vi "EC_Applied_XYZ_MM_BR_RES_2_NC_GR_pxi_Acc3_preset_LIM.vi"() -> ()   [LabVIEW 2009]
uses:
  <vilib>/Utility/file.llb/Read From Spreadsheet File (I64).vi
  <vilib>/Utility/file.llb/Read From Spreadsheet File (string).vi
  <vilib>/Instr/_visa.llb/VISA Configure Serial Port (Instr).vi
  <vilib>/Utility/file.llb/Write To Spreadsheet File (I64).vi
  <vilib>/Utility/file.llb/Write To Spreadsheet File (string).vi
panel:
  out "R Velocity MVdeg/sec":dbl format="%.3f"
  out "R Position MV deg":dbl
  out "Z Velocity MV mm/sec":dbl format="%.3f"
  out "Z Position MV mm":dbl
  out "Y Velocity MV mm/sec":dbl format="%.3f"
  out "Y Position MV mm":dbl
  out "X Velocity MV mm/sec":dbl format="%.3f"
  out "X Position MV mm":dbl
  out "Presets":i32[][](array[numeric])
  in  "stop":bool
  in  "Tab Control 3":enum32{"Status", "Reset"}(tab)
  out "Y in Range":bool
  out "Y Scan":bool
  out "Y in Motion":bool
  out "Y Backlash corr":bool
  out "X  in Range":bool
  out "X Scan":bool
  out "X  in Motion":bool
  out "X Backlash corr":bool
  out "Z in Range":bool
  out "Z Scan":bool
  out "Z in Motion":bool
  out "Z Backlash corr":bool
  out "R in Range":bool
  out "R Scan":bool
  out "R in Motion":bool
  out "R Backlash corr":bool
  out "X Ready":bool
  out "Y Ready":bool
  out "Z Ready":bool
  out "R Ready":bool
  in  "Reset Y Position mm":dbl
  out "Reset Y Motor Steps":i32
  in  "Reset X Position mm":dbl
  out "Reset X Motor Steps":i32
  in  "Reset Z Position mm":dbl
  out "Reset Z Motor Steps":i32
  in  "Reset R Position deg":dbl
  out "Reset R Motor Steps":i32
  in  "Reset":bool
  in  "Tab Control 2":enum32{"mm", "step"}(tab)
  in  "X Scan Length SP mm":dbl
  in  "X Scan Velocity SP mm/sec":dbl
  in  "X Scan set":bool
  in  "Y Scan Length SP mm":dbl
  in  "Y Scan Velocity SP mm/sec":dbl
  in  "Y Scan set":bool
  in  "Z Scan Length SP mm":dbl
  in  "Z Scan Velocity SP mm/sec":dbl
  in  "Z Scan set":bool
  in  "R Scan Length SP deg":dbl
  in  "R Scan Velocity SP deg/sec":dbl
  in  "R Scan set":bool
  in  "X Scan Velocity SP steps/sec":i32=1 min=1 max=102400 step=1
  in  "X Scan Length SP steps":i32 min=-500000 max=500000 step=100
  out "X Scan length MV mm":dbl
  out "X Scan velocity MV mm/sec":dbl format="%#_6f"
  in  "Y Scan Velocity SP steps/sec":i32=1 min=1 max=102400 step=1
  in  "Y Scan Length SP steps":i32 min=-1000000 max=0 step=100
  out "Y Scan length MV mm":dbl
  out "Y Scan velocity MV mm/sec":dbl format="%#_6f"
  in  "Z Scan Velocity SP steps/sec":i32=1 min=1 max=102400 step=1
  in  "Z Scan Length SP steps":i32 min=-204724 max=102195276 step=100
  out "Z Scan length MV mm":dbl
  out "Z Scan velocity MV mm/sec":dbl format="%#_6f"
  in  "R Scan Velocity SP steps/sec":i32=1 min=1 max=102400 step=1
  in  "R Scan Length SP steps":i32 min=-6144000 max=0 step=100
  out "R Scan length MV deg":dbl
  out "R Scan velocity MV deg/sec":dbl format="%#_6f"
  out "atan Y/Z":dbl
  in  "Tab Control":enum32{"mm", "preset", "step"}(tab)
  in  "X Position SP mm":dbl
  in  "X Velocity SP mm/sec":dbl
  in  "X Move Set":bool
  in  "Y Move Set":bool
  in  "Y Position SP mm":dbl
  in  "Y Velocity SP mm/sec":dbl
  in  "Z Position SP mm":dbl
  in  "Z Velocity SP mm/sec":dbl
  in  "Z Move Set":bool
  in  "R Position SP deg":dbl
  in  "R Velocity SP deg/sec":dbl
  in  "R Move Set":bool
  in  "Add Button":bool
  in  "String":string
  in  "Delete Button":bool
  in  "Preset positions":i32(ring) items=["ZERO", "Default", "CDOSE", "QMS", "test", "test2", "test3"]
  in  "Set Button":bool
  in  "X Velocity SP step/sec":i32 min=1 max=50000
  in  "Y Velocity SP step/sec":i32 min=1 max=50000
  in  "Z Velocity SP step/sec":i32 min=1 max=5000
  in  "R Velocity SP step/sec":i32 min=1 max=10000
  in  "Y Step SP":i32=-20000 min=-800000 max=800000 step=500
  in  "X Step SP":i32=-20000 min=-800000 max=800000 step=500
  in  "Z Step SP":i32=-20000 min=0 max=102400000 step=500
  in  "R Step SP":i32=-20000 min=-6144000 max=0 step=500
  out "X Step PV":i32 max=2000
  out "Y Step PV":i32 max=2000
  out "Z Step PV":i32 max=2000
  out "R Step PV":i32 max=2000
  in  "Clear ZY":bool
  out "ZY Graph":cluster{"Y":dbl[], "Y":dbl[]}[](graph)
  out "ZR Graph":cluster{"Y":dbl[], "Y":dbl[]}[](graph)
  out "XY Graph":cluster{"Y":dbl[], "Y":dbl[]}[](graph)
  out "X Scan Duration":dbl
  out "Y Scan Duration":dbl
  out "Z Scan Duration":dbl
  out "R Scan Duration":dbl
  out "R Backlash steps/sec":i32
  out "R Backlash":i32
  out "R Holding Current %":i32
  out "R Run Current %":i32
  out "R offset deg":dbl
  out "R deg/rev":dbl
  out "R steps/rev":u32
  out "R velocity PV step/sec":i32
  out "R MINPOS":i32=-94296
  out "R MAXPOS":i32=-34296
  out "R COM PORT":refnum<visa-resource-name>="COM5"
  in  "R Scan OK":bool
  in  "R Go":bool
  out "R Position deg PV":dbl
  out "Z COM PORT":refnum<visa-resource-name>="COM5"
  out "Z Backlash steps/sec":i32
  out "Z Backlash":i32
  out "Z Holding Current %":i32
  out "Z Run Current %":i32
  out "Z offset mm":dbl
  out "Z mm/rev":dbl
  out "Z steps/rev":u32
  out "Z  velocity PV step/sec":i32
  out "Z MINPOS":i32=-94296
  out "Z MAXPOS":i32=-34296
  in  "Z Scan OK":bool
  in  "Z Go":bool
  out "Z Position mm PV":dbl
  out "X Position mm PV":dbl
  out "X velocity PV step/sec":i32
  in  "X Scan OK":bool
  in  "X Go":bool
  out "X Backlash steps/sec":i32
  out "X Backlash":i32
  out "X Holding Current %":i32
  out "X Run Current %":i32
  out "X offset mm":dbl
  out "X mm/rev":dbl
  out "X steps/rev":u32
  out "X MAXPOS":i32=-34296
  out "X MINPOS":i32=-94296
  out "X COM PORT":refnum<visa-resource-name>="COM5"
  out "Y Backlash steps/sec":i32
  out "Y Backlash":i32
  out "Y Holding Current %":i32
  out "Y Run Current %":i32
  in  "Scan Cancel":bool
  out "Y Position mm PV":dbl
  out "Y offset mm":dbl
  out "Y mm/rev":dbl
  out "Y steps/rev":u32
  out "Y velocity PV step/sec":i32
  in  "Y Scan OK":bool
  in  "Scan Go":bool
  in  "Stop":bool
  in  "Y Go":bool
  out "Y MINPOS":i32=-94296
  out "Y MAXPOS":i32=-34296
  out "Y COM PORT":refnum<visa-resource-name>="COM5"
  # "Current position"
  # "Goto position"
  # "RX"
  # "RY"
  # "RZ"
  # "RR"
  # "L"
  # "M"
  # "B"
  # "S"
  # "R"
  # "Preset position"
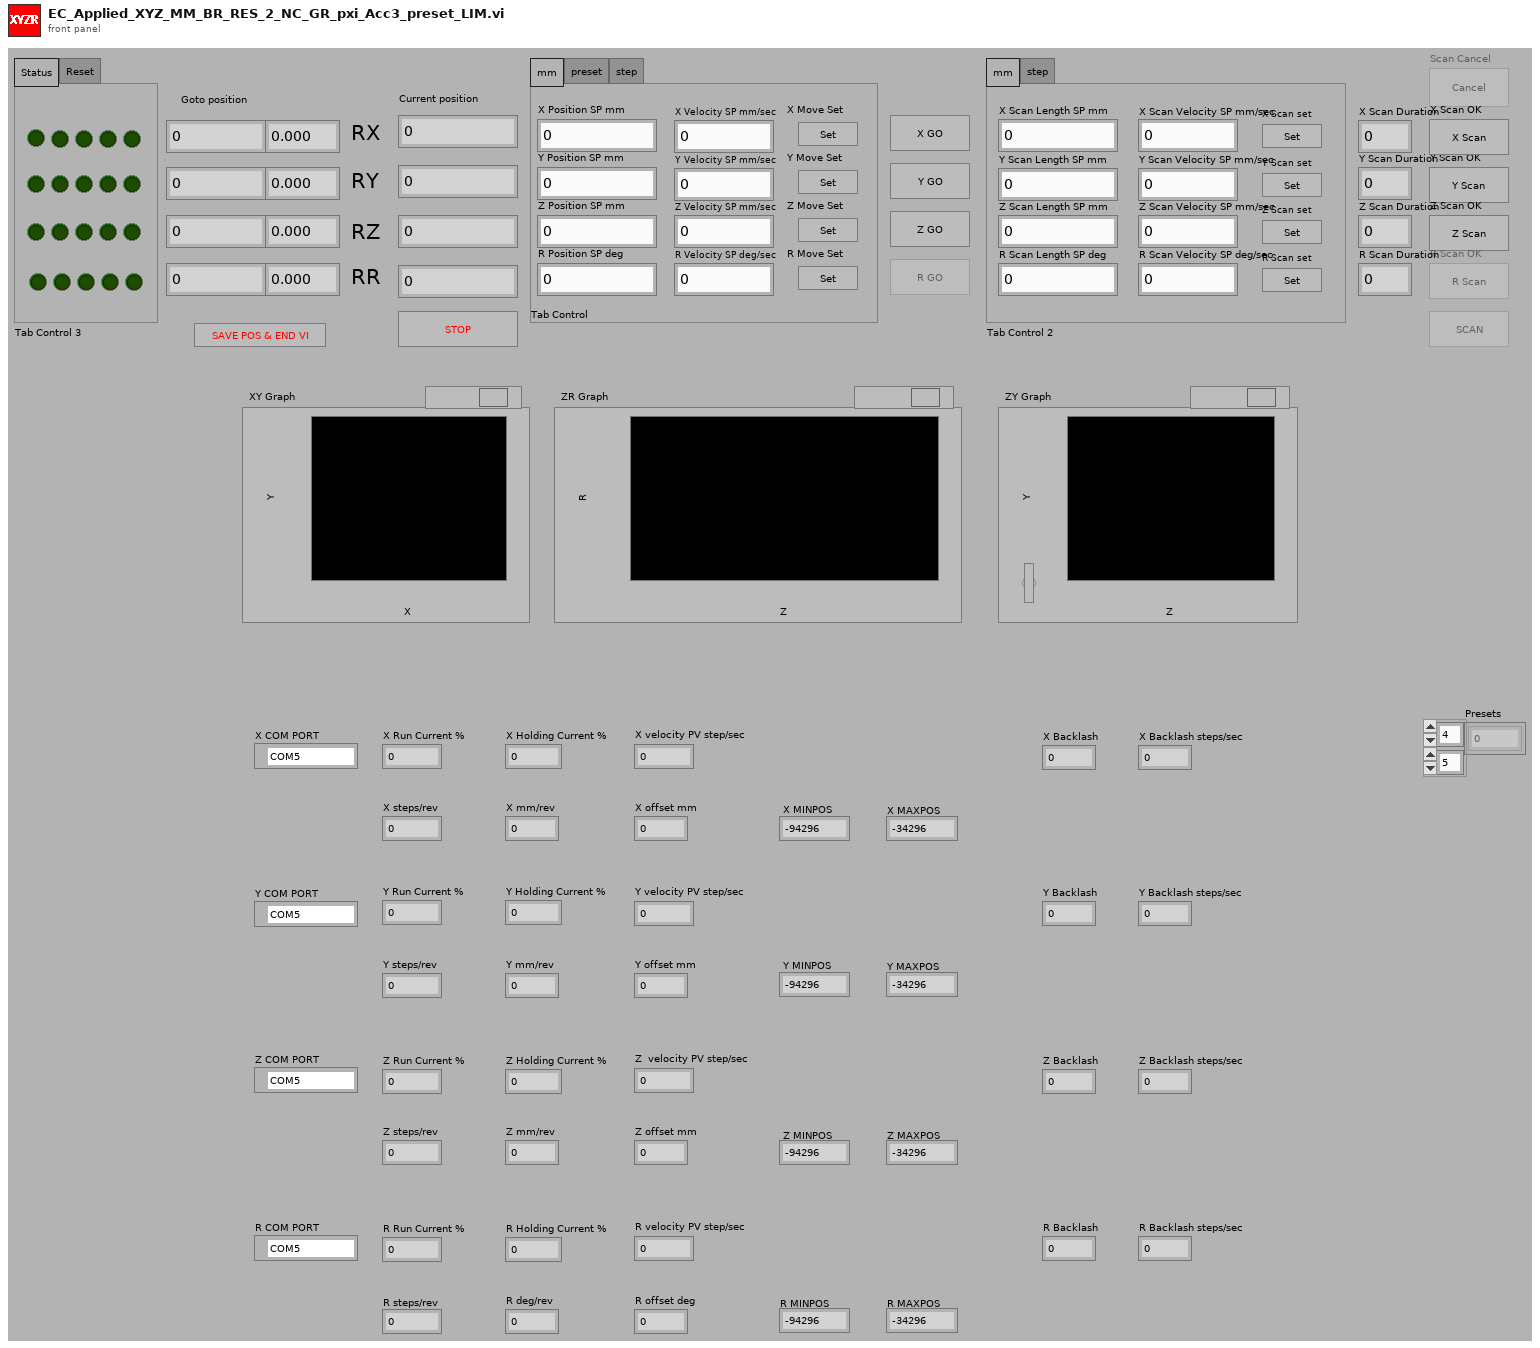
[diagram p1: front panel]
types:
  T1 = enum16{"Power-up Signature", "Accel Rate", "Accel Max", "Bit Rate", "Buffer Status", "Change Current", "Commence Jogging", "Change Jog Speed", "Continue", "Define Address", "Distance for FC,FM,FO,FY", "Decel Rate", "Distance or Position", "Define Limits", "Encoder Deadband", "Encoder Function", "Encoder Position", "Encoder Ratio", "Feed to Length with Speed Change", "Feed to Length", "Feed to Sensor with Mask Dist", "Feed to Length & Set Output", "Feed to Position", "Feed to Sensor", "Feed to Sensor w/safety", "Follow Handwheel", "Immediate Distance?", "Immediate Encoder?", "Immediate Low Output", "Immediate High Output", "Immediate Position?", "Input Status?", "Jog Accel/Decel", "Jog Disable", "Jog Enable", "Jog Speed", "Motor Disable", "Motor Enable", "Microstep Resolution", "Power up Current", "Power up Mode", "Pause", "Request Status", "Revision Level?", "Seek Home", "Stop Jogging", "Stop & Kill Buffer", "Set Output", "Set ABS Position", "Send String", "Stop", "Velocity for Speed Change", "Velocity Setting", "Wait for Input", "Wait Time"}
  T2 = enum8{"Enabled", "Disabled", "Disabled and Grayed Out"}
  T3 = cluster{"first row[0]":i64, "first row[1]":i64, "first row[2]":i64, "first row[3]":i64, "first row[4]":i64, "first row[5]":i64, "first row[6]":i64, "first row[7]":i64, "first row[8]":i64}
  T4 = cluster{"Value[0]":i32, "Value[1]":i32, "Value[2]":i32, "Value[3]":i32, "Value[4]":i32, "Value[5]":i32, "Value[6]":i32, "Value[7]":i32, "Value[8]":i32}
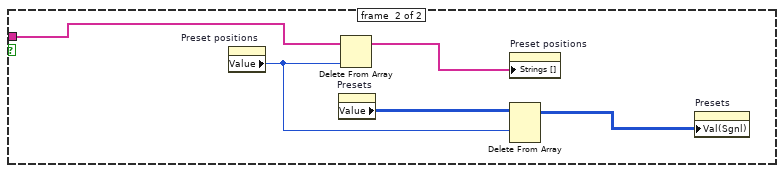
[diagram p2: hidden frame]
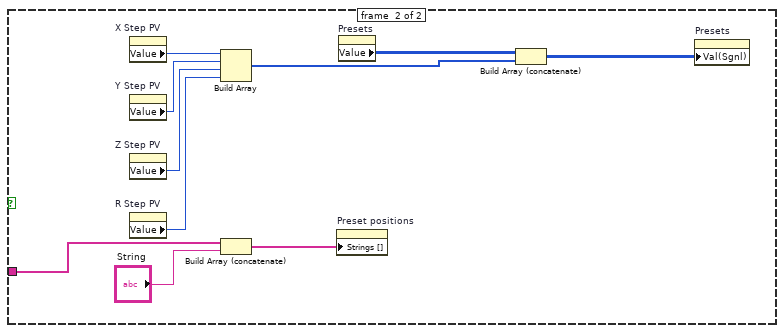
[diagram p3: hidden frame]
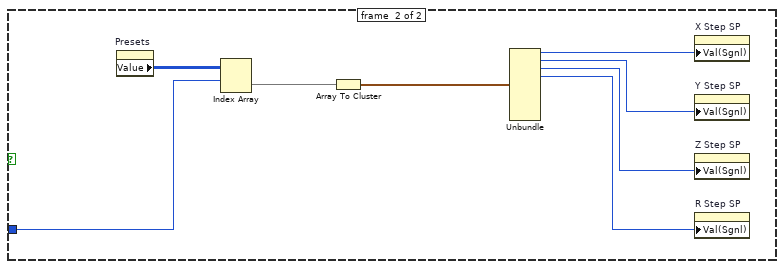
[diagram p4: hidden frame]
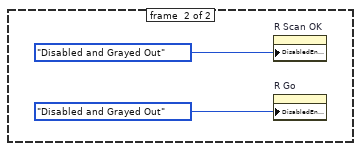
[diagram p5: hidden frame]
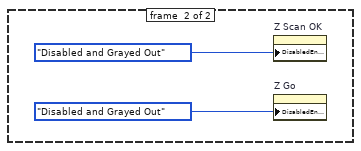
[diagram p8: hidden frame]
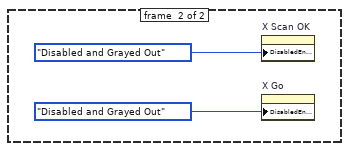
[diagram p11: hidden frame]
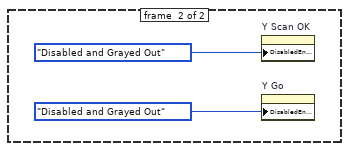
[diagram p14: hidden frame]
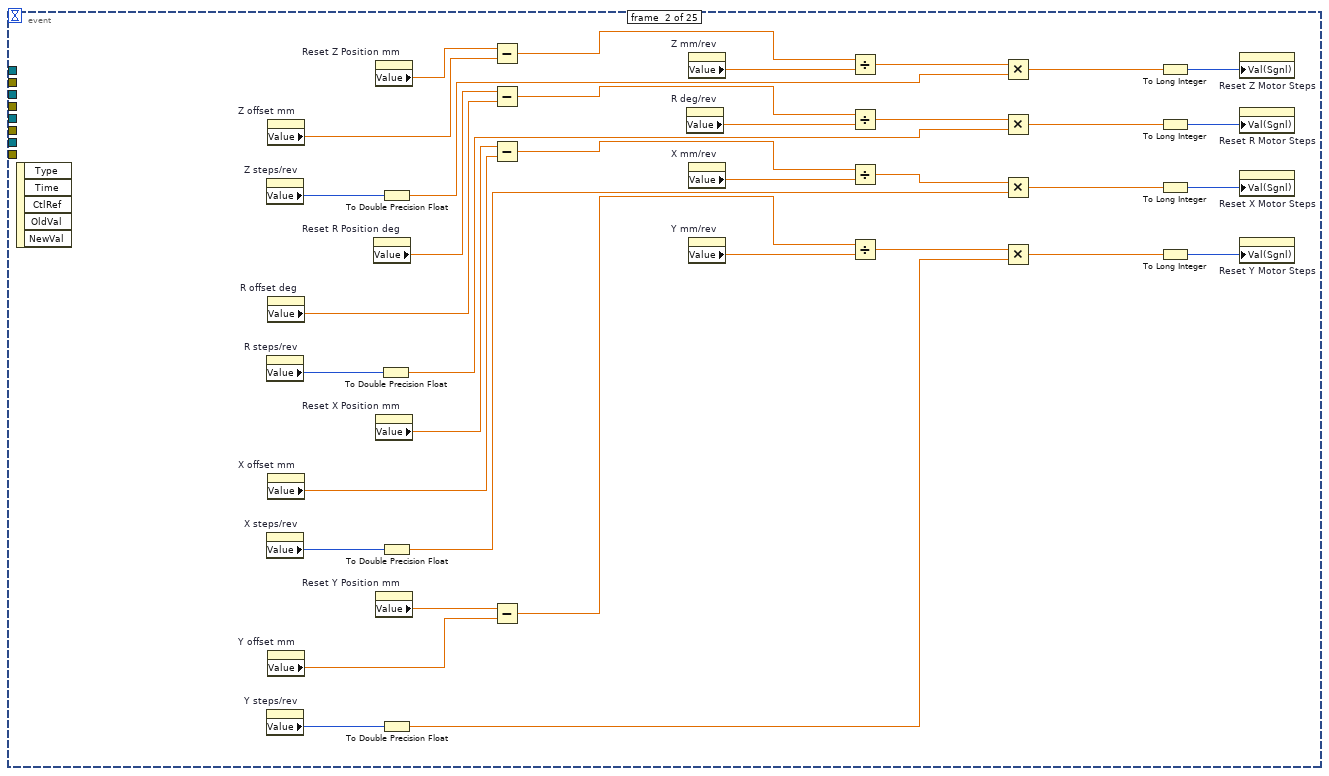
[diagram p17: hidden frame]
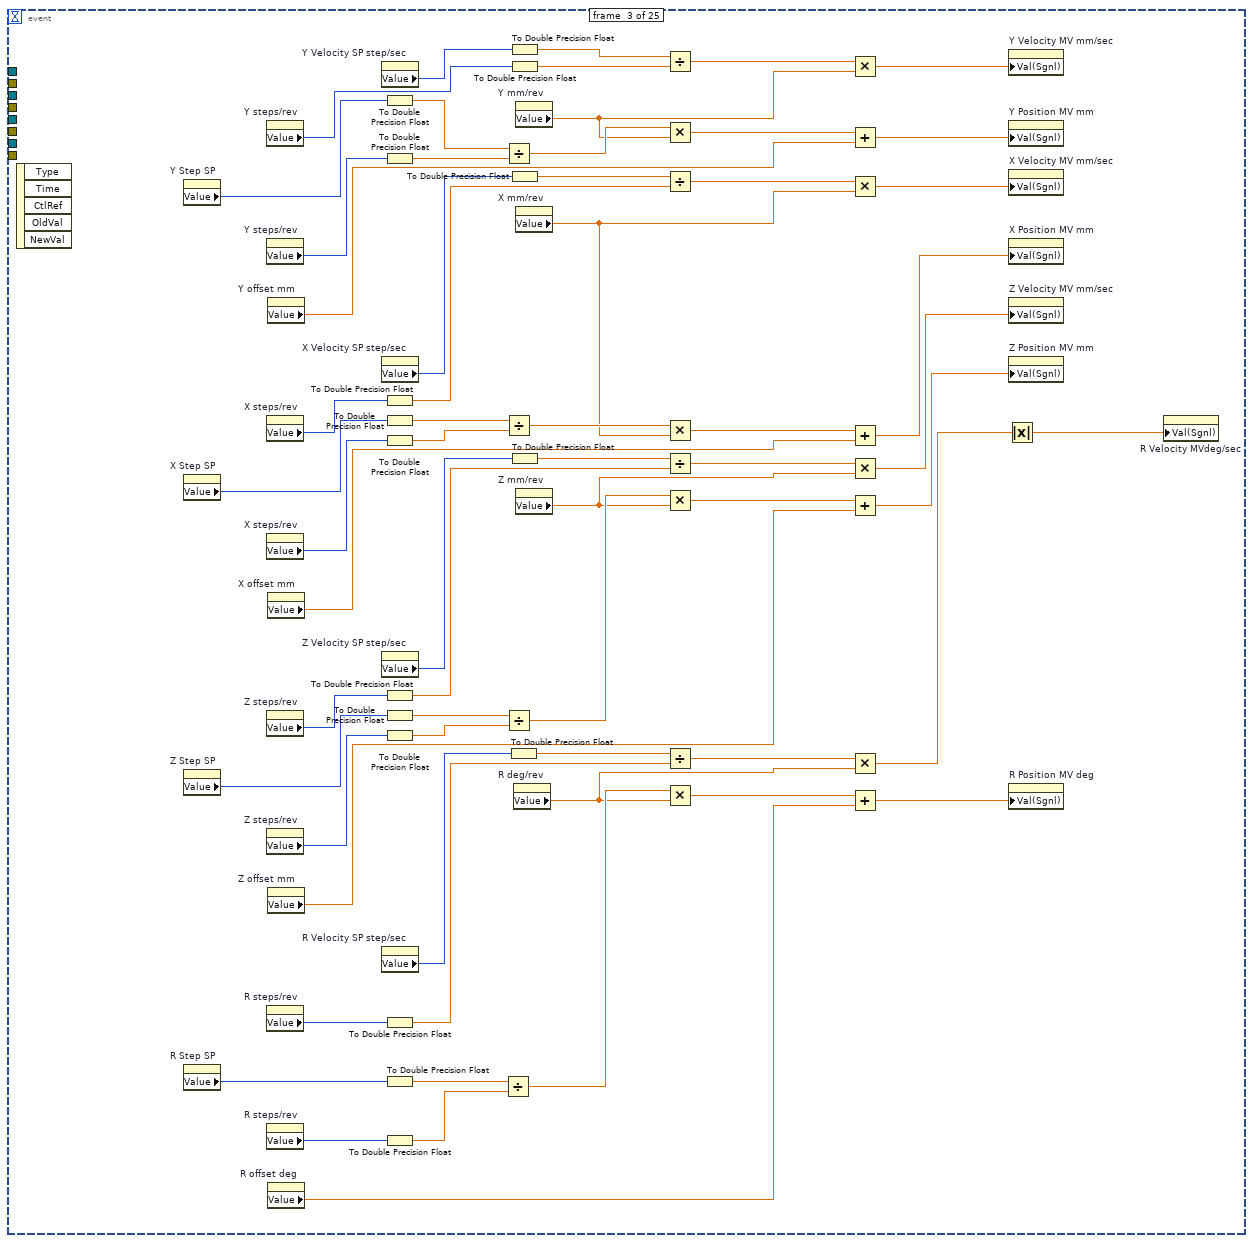
[diagram p18: hidden frame]
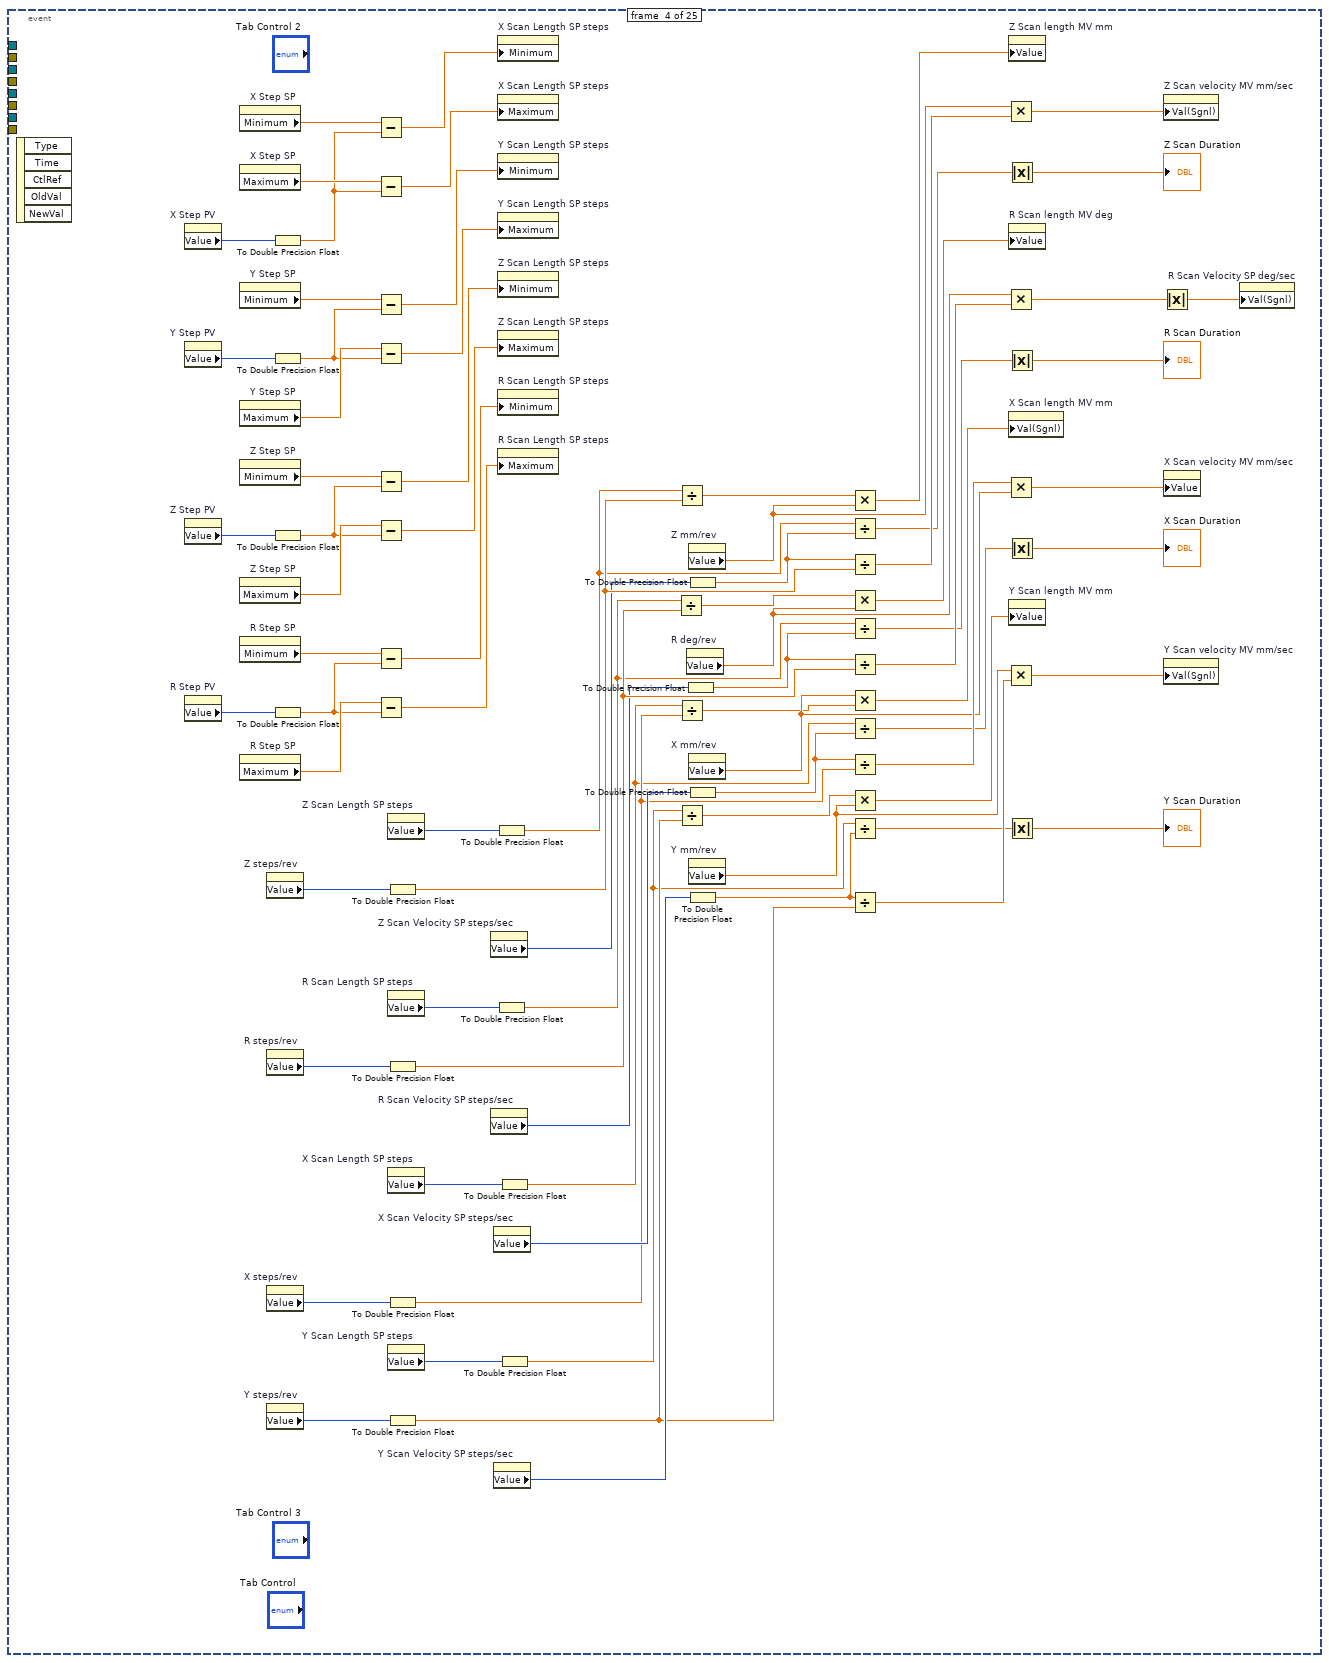
[diagram p19: hidden frame]
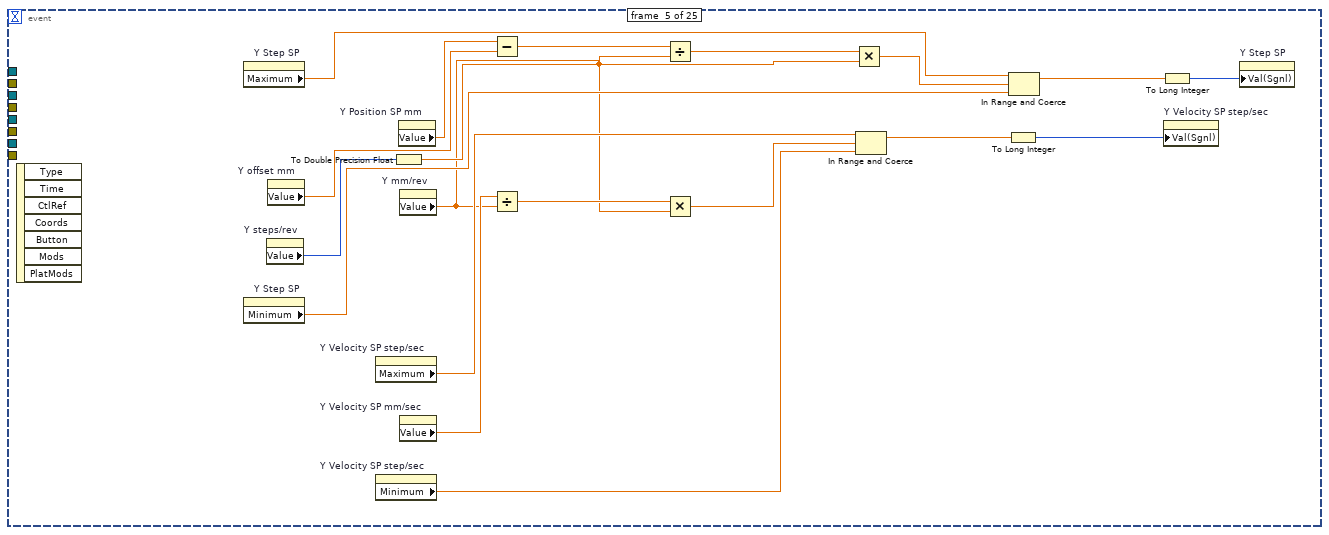
[diagram p20: hidden frame]
diagram:
  w24 = 0 ("dimension size")
  n1 = flat-sequence {
    tunnel: [w93] -> w10
    tunnel: [w92] -> w9
    tunnel: w10 -> [w104]
    tunnel: w9 -> [w103]
    tunnel: [w102] -> w8
    tunnel: [w101] -> w7
    tunnel: [w113] -> w64
    tunnel: [w112] -> w63
    tunnel: w8 -> [w115]
    tunnel: w7 -> [w114]
    tunnel: w64 -> [w130]
    tunnel: w63 -> [w129]
    tunnel: [w131] -> w62
    tunnel: [w132] -> w61
    tunnel: [w133] -> w6
    tunnel: [w144] -> w55
    tunnel: [w145] -> w56
    tunnel: w62 -> [w145]
    tunnel: w61 -> [w144]
    tunnel: w6 -> [w142]
    frame #0 {
      "Z Run Current %" <- 100 ("Z Run Current %")
      "Z Holding Current %" <- 50 ("Z Holding Current %")
    }
    frame #1 {
      "Z Backlash steps/sec" <- 1000 ("Z Backlash steps/sec")
      "Z Backlash" <- -5000 ("Z Backlash")
    }
    frame #2 {
      w83 = 2.54 ("Z mm/rev")
      w82 = u32 20000 ("step/rev")
      w84 = 5000 ("Value (Signaling)")
      n2 = property on="Z Velocity SP step/sec" class="DigNum (strict)"("Minimum"=1.0 ("Data Entry Limits:Minimum")) -> ()  [unwired: 2 in, 2 out]
      n3 = property on="Z Scan Velocity SP mm/sec" class="DigNum (strict)"("Val(Sgnl)"=0.1 ("Value (Signaling)")) -> ()  [unwired: 2 in, 2 out]
      n4 = property on="Z Velocity SP step/sec" class="DigNum (strict)"("Val(Sgnl)"=w84) -> ()  [unwired: 2 in, 2 out]
      n5 = To Double Precision Float(number=w82) -> (double precision float=w87:dbl)
      n6 = To Double Precision Float(number=w84) -> (double precision float=w88:dbl)
      n7 = Divide(x=w88, y=w87) -> (x/y=w85:dbl)
      n8 = property on="Z Velocity SP step/sec" class="DigNum (strict)"("Maximum"=w88) -> ()  [unwired: 2 in, 2 out]
      n9 = Multiply(x=w85, y=w83) -> (x*y=w86:dbl)
      n10 = property on="Z Velocity SP mm/sec" class="DigNum (strict)"("Val(Sgnl)"=w86) -> ()  [unwired: 2 in, 2 out]
      "Z mm/rev" <- w83
      "Z steps/rev" <- w82
    }
    frame #3 {
      w90 = 0 ("lower limit")
      w89 = 102400000 ("upper limit")
      n11 = property on="Z Step SP" class="DigNum (strict)"("Minimum"=w90) -> ()  [unwired: 2 in, 2 out]
      n12 = property on="Z Step SP" class="DigNum (strict)"("Maximum"=w89) -> ()  [unwired: 2 in, 2 out]
      "Z offset mm" <- 0.0 ("Z offset mm")
      "Z MINPOS" <- w90
      "Z MAXPOS" <- w89
    }
    frame #4 {
      w100 = refnum<visa-resource-name> "COM5" ("COM PORT")
      w98 = u16 0 items=["None", "XON/XOFF", "RTS/CTS", "XON/XOFF & RTS/CTS", "DTR/DSR", "XON/XOFF & DTR/DSR"] ("flow control (0:none)")
      w97 = u16 10 items=["1.0"=10, "1.5"=15, "2.0"=20] ("stop bits (10: 1 bit)")
      # "Stop bits"
      n13 = call-poly "VISA Configure Serial Port"("VISA resource name"=w100, "timeout (10sec)"=u32 10000, "baud rate (9600)"=u32 9600, "data bits (8)"=u16 8, "parity (0:none)"=enum16{"None", "Odd", "Even", "Mark", "Space"}."None", "stop bits (10: 1 bit)"=w97, "flow control (0:none)"=w98) -> ("VISA resource name out"=w93:refnum<visa-resource-name>, "error out"=w92:errorcluster)  [unwired: 7 in]
      "Z COM PORT" <- w100
    }
    frame #5 {
      # "Run Current %"
      n14 = property on="Z Run Current %" class="DigNum (strict)"() -> ("Value"=w105:i32)  [unwired: 2 in, 2 out]
      n15 = Divide(x=w105, y=3.5) -> (x/y=w107:dbl)
      n16 = Number To Fractional String(number=w107) -> (F-format string=w108:string)  [unwired: 3 in]
      n17 = call "Applied Send Command.vi"("error in (no error)"=w103, "Extra"=w108, "Command"=T1."Change Current", "VISA resource name"=w104) -> ("error out"=w101:errorcluster, "VISA resource name out"=w102:refnum<visa-resource-name>)  [unwired: 3 in, 1 out]
    }
    frame #6 {
      # "VELOCITY"
      n18 = property on="Z steps/rev" class="DigNum (strict)"() -> ("Value"=w111:u32)  [unwired: 2 in, 2 out]
      n19 = property on="Z Velocity SP step/sec" class="DigNum (strict)"() -> ("Value"=w110:i32)  [unwired: 2 in, 2 out]
      n20 = Divide(x=w110, y=w111) -> (x/y=w118:dbl)
      n21 = Number To Fractional String(number=w118) -> (F-format string=w120:string)  [unwired: 3 in]
      n22 = call "Applied Send Command.vi"("error in (no error)"=w114, "Extra"=w120, "Command"=T1."Velocity Setting", "VISA resource name"=w115) -> ("error out"=w121:errorcluster, "VISA resource name out"=w128:refnum<visa-resource-name>)  [unwired: 3 in, 1 out]
      n23 = call "Time Delay2"("error in (no error)"=w121, "Delay Time (s)"=0.1) -> ("error out"=w126:errorcluster)  [unwired: 9 in]
      n24 = call "Applied Send Command.vi"("error in (no error)"=w126, "Extra"="", "Command"=T1."Velocity Setting", "VISA resource name"=w128) -> ("error out"=w112:errorcluster, "read buffer"=w124:string, "VISA resource name out"=w113:refnum<visa-resource-name>)  [unwired: 3 in]
      n25 = Fract/Exp String To Number(string=w124, offset=3) -> (number=w119:dbl)  [unwired: 2 in, 1 out]
      n26 = Multiply(x=w119, y=w111) -> (x*y=w116:dbl)
      n27 = property on="Z  velocity PV step/sec" class="DigNum (strict)"("Val(Sgnl)"=w116) -> ()  [unwired: 2 in, 2 out]
    }
    frame #7 {
      # "GET CURRENT POSITION"
      n28 = call "Applied Send Command.vi"("error in (no error)"=w129, "Extra"="", "Command"=T1."Immediate Position?", "VISA resource name"=w130) -> ("error out"=w135:errorcluster, "read buffer"=w137:string, "VISA resource name out"=w131:refnum<visa-resource-name>)  [unwired: 3 in]
      n29 = call "Time Delay8"("error in (no error)"=w135, "Delay Time (s)"=0.1) -> ("error out"=w132:errorcluster)  [unwired: 9 in]
      n30 = Hexadecimal String To Number(string=w137, offset=3) -> (number=w133:u32)  [unwired: 1 in, 1 out]
    }
    frame #8 {
      n31 = property on="Z Step SP" class="DigNum (strict)"("Val(Sgnl)"=w142) -> ()  [unwired: 2 in, 2 out]
      n32 = property on="Z Step SP" class="DigNum (strict)"() -> ("Maximum"=w141:dbl)  [unwired: 2 in, 2 out]
      n33 = property on="Z Step SP" class="DigNum (strict)"() -> ("Minimum"=w140:dbl)  [unwired: 2 in, 2 out]
      n34 = In Range and Coerce(upper limit=w141, x=w142, lower limit=w140) -> (In Range?=w143:bool)  [unwired: 1 out]
      n35 = property on="Z in Range" class="Bool (strict)"("Val(Sgnl)"=w143) -> ()  [unwired: 2 in, 2 out]
    }
  }
  n36 = flat-sequence {
    tunnel: [w164] -> w3
    tunnel: [w163] -> w2
    tunnel: [w175] -> w5
    tunnel: [w174] -> w4
    tunnel: w3 -> [w173]
    tunnel: w2 -> [w172]
    tunnel: [w183] -> w60
    tunnel: [w184] -> w59
    tunnel: w5 -> [w181]
    tunnel: w4 -> [w182]
    tunnel: w60 -> [w201]
    tunnel: w59 -> [w200]
    tunnel: [w202] -> w58
    tunnel: [w204] -> w57
    tunnel: [w203] -> w1
    tunnel: [w215] -> w53
    tunnel: [w216] -> w54
    tunnel: w58 -> [w215]
    tunnel: w57 -> [w213]
    tunnel: w1 -> [w216]
    frame #0 {
      "R Run Current %" <- 100 ("R Run Current %")
      "R Holding Current %" <- 50 ("R Holding Current %")
    }
    frame #1 {
      "R Backlash" <- -12800 ("R Backlash")
      "R Backlash steps/sec" <- 6400 ("R Backlash steps/sec")
    }
    frame #2 {
      w154 = -3.0 ("R deg/rev")
      w156 = u32 20000 ("step/rev")
      w152 = 10000 ("Value (Signaling)")
      n37 = property on="R Velocity SP deg/sec" class="DigNum (strict)"("Val(Sgnl)"=0.1 ("Value (Signaling)")) -> ()  [unwired: 2 in, 2 out]
      n38 = property on="R Velocity SP step/sec" class="DigNum (strict)"("Val(Sgnl)"=w152) -> ()  [unwired: 2 in, 2 out]
      n39 = property on="R Velocity SP step/sec" class="DigNum (strict)"("Minimum"=1.0 ("Data Entry Limits:Minimum")) -> ()  [unwired: 2 in, 2 out]
      n40 = To Double Precision Float(number=w156) -> (double precision float=w155:dbl)
      n41 = To Double Precision Float(number=w152) -> (double precision float=w150:dbl)
      n42 = Divide(x=w150, y=w155) -> (x/y=w151:dbl)
      n43 = property on="R Velocity SP step/sec" class="DigNum (strict)"("Maximum"=w150) -> ()  [unwired: 2 in, 2 out]
      n44 = Multiply(x=w151, y=w154) -> (x*y=w153:dbl)
      n45 = Absolute Value(x=w153) -> (abs(x)=w158:dbl)
      n46 = property on="R Velocity SP deg/sec" class="DigNum (strict)"("Val(Sgnl)"=w158) -> ()  [unwired: 2 in, 2 out]
      "R deg/rev" <- w154
      "R steps/rev" <- w156
    }
    frame #3 {
      w161 = 0 ("upper limit")
      w162 = -6144000 ("lower limit")
      n47 = property on="R Step SP" class="DigNum (strict)"("Minimum"=w162) -> ()  [unwired: 2 in, 2 out]
      n48 = property on="R Step SP" class="DigNum (strict)"("Maximum"=w161) -> ()  [unwired: 2 in, 2 out]
      "R MINPOS" <- w161
      "R MAXPOS" <- w162
      "R offset deg" <- 0.0 ("R offset deg")
    }
    frame #4 {
      w171 = refnum<visa-resource-name> "COM6" ("COM PORT")
      w169 = u16 0 items=["None", "XON/XOFF", "RTS/CTS", "XON/XOFF & RTS/CTS", "DTR/DSR", "XON/XOFF & DTR/DSR"] ("flow control (0:none)")
      w168 = u16 10 items=["1.0"=10, "1.5"=15, "2.0"=20] ("stop bits (10: 1 bit)")
      # "Stop bits"
      n49 = call-poly "VISA Configure Serial Port"("VISA resource name"=w171, "timeout (10sec)"=u32 10000, "baud rate (9600)"=u32 9600, "data bits (8)"=u16 8, "parity (0:none)"=enum16{"None", "Odd", "Even", "Mark", "Space"}."None", "stop bits (10: 1 bit)"=w168, "flow control (0:none)"=w169) -> ("VISA resource name out"=w164:refnum<visa-resource-name>, "error out"=w163:errorcluster)  [unwired: 7 in]
      "R COM PORT" <- w171
    }
    frame #5 {
      # "Run Current %"
      n50 = property on="R Run Current %" class="DigNum (strict)"() -> ("Value"=w176:i32)  [unwired: 2 in, 2 out]
      n51 = Divide(x=w176, y=3.5) -> (x/y=w178:dbl)
      n52 = Number To Fractional String(number=w178) -> (F-format string=w179:string)  [unwired: 3 in]
      n53 = call "Applied Send Command.vi"("error in (no error)"=w172, "Extra"=w179, "Command"=T1."Change Current", "VISA resource name"=w173) -> ("error out"=w174:errorcluster, "VISA resource name out"=w175:refnum<visa-resource-name>)  [unwired: 3 in, 1 out]
    }
    frame #6 {
      # "VELOCITY"
      n54 = property on="R steps/rev" class="DigNum (strict)"() -> ("Value"=w187:u32)  [unwired: 2 in, 2 out]
      n55 = property on="R Velocity SP step/sec" class="DigNum (strict)"() -> ("Value"=w185:i32)  [unwired: 2 in, 2 out]
      n56 = Divide(x=w185, y=w187) -> (x/y=w189:dbl)
      n57 = Number To Fractional String(number=w189) -> (F-format string=w191:string)  [unwired: 3 in]
      n58 = call "Applied Send Command.vi"("error in (no error)"=w182, "Extra"=w191, "Command"=T1."Velocity Setting", "VISA resource name"=w181) -> ("error out"=w192:errorcluster, "VISA resource name out"=w199:refnum<visa-resource-name>)  [unwired: 3 in, 1 out]
      n59 = call "Time Delay43"("error in (no error)"=w192, "Delay Time (s)"=0.1) -> ("error out"=w197:errorcluster)  [unwired: 9 in]
      n60 = call "Applied Send Command.vi"("error in (no error)"=w197, "Extra"="", "Command"=T1."Velocity Setting", "VISA resource name"=w199) -> ("error out"=w184:errorcluster, "read buffer"=w195:string, "VISA resource name out"=w183:refnum<visa-resource-name>)  [unwired: 3 in]
      n61 = Fract/Exp String To Number(string=w195, offset=3) -> (number=w190:dbl)  [unwired: 2 in, 1 out]
      n62 = Multiply(x=w190, y=w187) -> (x*y=w186:dbl)
      n63 = property on="R velocity PV step/sec" class="DigNum (strict)"("Val(Sgnl)"=w186) -> ()  [unwired: 2 in, 2 out]
    }
    frame #7 {
      # "GET CURRENT POSITION"
      n64 = call "Applied Send Command.vi"("error in (no error)"=w200, "Extra"="", "Command"=T1."Immediate Position?", "VISA resource name"=w201) -> ("error out"=w206:errorcluster, "read buffer"=w208:string, "VISA resource name out"=w203:refnum<visa-resource-name>)  [unwired: 3 in]
      n65 = call "Time Delay42"("error in (no error)"=w206, "Delay Time (s)"=0.1) -> ("error out"=w202:errorcluster)  [unwired: 9 in]
      n66 = Hexadecimal String To Number(string=w208, offset=3) -> (number=w204:u32)  [unwired: 1 in, 1 out]
    }
    frame #8 {
      n67 = property on="R Step SP" class="DigNum (strict)"("Val(Sgnl)"=w213) -> ()  [unwired: 2 in, 2 out]
      n68 = property on="R Step SP" class="DigNum (strict)"() -> ("Maximum"=w211:dbl)  [unwired: 2 in, 2 out]
      n69 = property on="R Step SP" class="DigNum (strict)"() -> ("Minimum"=w212:dbl)  [unwired: 2 in, 2 out]
      n70 = In Range and Coerce(upper limit=w211, x=w213, lower limit=w212) -> (In Range?=w214:bool)  [unwired: 1 out]
      n71 = property on="R in Range" class="Bool (strict)"("Val(Sgnl)"=w214) -> ()  [unwired: 2 in, 2 out]
    }
  }
  n72 = flat-sequence {
    frame #0 {
      n73 = property on="R Scan" class="Bool (strict)"("Val(Sgnl)"=FALSE ("Value (Signaling)")) -> ()  [unwired: 2 in, 2 out]
      n74 = property on="Z Scan" class="Bool (strict)"("Val(Sgnl)"=FALSE ("Value (Signaling)")) -> ()  [unwired: 2 in, 2 out]
      n75 = property on="Y Scan" class="Bool (strict)"("Val(Sgnl)"=FALSE ("Value (Signaling)")) -> ()  [unwired: 2 in, 2 out]
      n76 = property on="X Scan" class="Bool (strict)"("Val(Sgnl)"=FALSE ("Value (Signaling)")) -> ()  [unwired: 2 in, 2 out]
      n77 = property on="Scan Cancel" class="Bool"("DisabledEnum"=T2."Disabled and Grayed Out" ("Disabled")) -> ()  [unwired: 2 in, 2 out]
      n78 = property on="Scan Go" class="Bool"("DisabledEnum"=T2."Disabled and Grayed Out" ("Disabled")) -> ()  [unwired: 2 in, 2 out]
    }
    frame #1 {
      n79 = property on="Z Backlash corr" class="Bool (strict)"("Val(Sgnl)"=FALSE ("Value (Signaling)")) -> ()  [unwired: 2 in, 2 out]
      n80 = property on="X Backlash corr" class="Bool (strict)"("Val(Sgnl)"=FALSE ("Value (Signaling)")) -> ()  [unwired: 2 in, 2 out]
      n81 = property on="R Backlash corr" class="Bool (strict)"("Val(Sgnl)"=FALSE ("Value (Signaling)")) -> ()  [unwired: 2 in, 2 out]
      n82 = property on="Y Backlash corr" class="Bool (strict)"("Val(Sgnl)"=FALSE ("Value (Signaling)")) -> ()  [unwired: 2 in, 2 out]
    }
  }
  n83 = flat-sequence {
    tunnel: [w244] -> w23
    tunnel: [w243] -> w22
    tunnel: w23 -> [w259]
    tunnel: w22 -> [w258]
    tunnel: [w257] -> w21
    tunnel: [w256] -> w20
    tunnel: [w262] -> w73
    tunnel: w21 -> [w270]
    tunnel: w20 -> [w269]
    tunnel: [w263] -> w19
    tunnel: w73 -> [w284]
    tunnel: [w283] -> w67
    tunnel: [w281] -> w66
    tunnel: [w286] -> w65
    tunnel: w19 -> [w285]
    tunnel: [w295] -> w71
    tunnel: [w296] -> w72
    tunnel: w67 -> [w296]
    tunnel: w66 -> [w295]
    tunnel: w65 -> [w291]
    frame #0 {
      "X Run Current %" <- 100 ("Run Current %")
      "X Holding Current %" <- 50 ("Holding Current %")
    }
    frame #1 {
      "X Backlash steps/sec" <- 10000 ("Value (Signaling)")
      "X Backlash" <- 5000 ("Backlash2")
    }
    frame #2 {
      w233 = 0.21167 ("MM/rev")
      w236 = u32 20000 ("step/rev")
      w231 = 50000 ("Value (Signaling)")
      n84 = property on="X Scan Velocity SP mm/sec" class="DigNum (strict)"("Val(Sgnl)"=0.1 ("Value (Signaling)")) -> ()  [unwired: 2 in, 2 out]
      n85 = property on="X Velocity SP step/sec" class="DigNum (strict)"("Minimum"=1.0 ("Data Entry Limits:Minimum")) -> ()  [unwired: 2 in, 2 out]
      n86 = property on="X Velocity SP step/sec" class="DigNum (strict)"("Val(Sgnl)"=w231) -> ()  [unwired: 2 in, 2 out]
      n87 = To Double Precision Float(number=w236) -> (double precision float=w235:dbl)
      n88 = To Double Precision Float(number=w231) -> (double precision float=w237:dbl)
      n89 = Divide(x=w237, y=w235) -> (x/y=w232:dbl)
      n90 = property on="X Velocity SP step/sec" class="DigNum (strict)"("Maximum"=w237) -> ()  [unwired: 2 in, 2 out]
      n91 = Multiply(x=w232, y=w233) -> (x*y=w234:dbl)
      n92 = property on="X Velocity SP mm/sec" class="DigNum (strict)"("Val(Sgnl)"=w234) -> ()  [unwired: 2 in, 2 out]
      "X steps/rev" <- w236
      "X mm/rev" <- w233
    }
    frame #3 {
      w242 = -750000 ("lower limit")
      w241 = 750000 ("upper limit")
      n93 = property on="X Step SP" class="DigNum (strict)"("Minimum"=w242) -> ()  [unwired: 2 in, 2 out]
      n94 = property on="X Step SP" class="DigNum (strict)"("Maximum"=w241) -> ()  [unwired: 2 in, 2 out]
      "X offset mm" <- 0.0 ("offset")
      "X MAXPOS" <- w241
      "X MINPOS" <- w242
    }
    frame #4 {
      w251 = refnum<visa-resource-name> "COM3" ("COM PORT")
      w249 = u16 0 items=["None", "XON/XOFF", "RTS/CTS", "XON/XOFF & RTS/CTS", "DTR/DSR", "XON/XOFF & DTR/DSR"] ("flow control (0:none)")
      w248 = u16 10 items=["1.0"=10, "1.5"=15, "2.0"=20] ("stop bits (10: 1 bit)")
      # "Stop bits"
      n95 = call-poly "VISA Configure Serial Port"("VISA resource name"=w251, "timeout (10sec)"=u32 10000, "baud rate (9600)"=u32 9600, "data bits (8)"=u16 8, "parity (0:none)"=enum16{"None", "Odd", "Even", "Mark", "Space"}."None", "stop bits (10: 1 bit)"=w248, "flow control (0:none)"=w249) -> ("VISA resource name out"=w244:refnum<visa-resource-name>, "error out"=w243:errorcluster)  [unwired: 7 in]
      "X COM PORT" <- w251
    }
    frame #5 {
      n96 = property on="X Run Current" class="DigNum (strict)"() -> ("Value"=w252:i32)  [unwired: 2 in, 2 out]
      n97 = Divide(x=w252, y=3.5) -> (x/y=w254:dbl)
      n98 = Number To Fractional String(number=w254) -> (F-format string=w255:string)  [unwired: 3 in]
      n99 = call "Applied Send Command.vi"("error in (no error)"=w258, "Extra"=w255, "Command"=T1."Change Current", "VISA resource name"=w259) -> ("error out"=w257:errorcluster, "VISA resource name out"=w256:refnum<visa-resource-name>)  [unwired: 3 in, 1 out]
    }
    frame #6 {
      # "VELOCITY"
      n100 = property on="X steps/rev" class="DigNum (strict)"() -> ("Value"=w265:u32)  [unwired: 2 in, 2 out]
      n101 = property on="X Velocity SP step/sec" class="DigNum (strict)"() -> ("Value"=w266:i32)  [unwired: 2 in, 2 out]
      n102 = Divide(x=w266, y=w265) -> (x/y=w264:dbl)
      n103 = Number To Fractional String(number=w264) -> (F-format string=w271:string)  [unwired: 3 in]
      n104 = call "Applied Send Command.vi"("error in (no error)"=w270, "Extra"=w271, "Command"=T1."Velocity Setting", "VISA resource name"=w269) -> ("error out"=w272:errorcluster, "VISA resource name out"=w279:refnum<visa-resource-name>)  [unwired: 3 in, 1 out]
      n105 = call "Time Delay30"("error in (no error)"=w272, "Delay Time (s)"=0.1) -> ("error out"=w277:errorcluster)  [unwired: 9 in]
      n106 = call "Applied Send Command.vi"("error in (no error)"=w277, "Extra"="", "Command"=T1."Velocity Setting", "VISA resource name"=w279) -> ("error out"=w262:errorcluster, "read buffer"=w275:string, "VISA resource name out"=w263:refnum<visa-resource-name>)  [unwired: 3 in]
      n107 = Fract/Exp String To Number(string=w275, offset=3) -> (number=w268:dbl)  [unwired: 2 in, 1 out]
      n108 = Multiply(x=w268, y=w265) -> (x*y=w267:dbl)
      n109 = property on="X velocity PV step/sec" class="DigNum (strict)"("Val(Sgnl)"=w267) -> ()  [unwired: 2 in, 2 out]
    }
    frame #7 {
      # "GET CURRENT POSITION"
      n110 = call "Applied Send Command.vi"("error in (no error)"=w284, "Extra"="", "Command"=T1."Immediate Position?", "VISA resource name"=w285) -> ("error out"=w282:errorcluster, "read buffer"=w288:string, "VISA resource name out"=w283:refnum<visa-resource-name>)  [unwired: 3 in]
      n111 = call "Time Delay13"("error in (no error)"=w282, "Delay Time (s)"=0.1) -> ("error out"=w281:errorcluster)  [unwired: 9 in]
      n112 = Hexadecimal String To Number(string=w288, offset=3) -> (number=w286:u32)  [unwired: 1 in, 1 out]
    }
    frame #8 {
      n113 = property on="X Step SP" class="DigNum (strict)"("Val(Sgnl)"=w291) -> ()  [unwired: 2 in, 2 out]
      n114 = property on="X Step SP" class="DigNum (strict)"() -> ("Maximum"=w294:dbl)  [unwired: 2 in, 2 out]
      n115 = property on="X Step SP" class="DigNum (strict)"() -> ("Minimum"=w293:dbl)  [unwired: 2 in, 2 out]
      n116 = In Range and Coerce(upper limit=w294, x=w291, lower limit=w293) -> (In Range?=w292:bool)  [unwired: 1 out]
      n117 = property on="X  in Range" class="Bool (strict)"("Val(Sgnl)"=w292) -> ()  [unwired: 2 in, 2 out]
    }
  }
  n118 = flat-sequence {
    tunnel: [w314] -> w18
    tunnel: [w313] -> w17
    tunnel: w18 -> [w325]
    tunnel: w17 -> [w324]
    tunnel: [w323] -> w16
    tunnel: [w322] -> w15
    tunnel: w16 -> [w334]
    tunnel: w15 -> [w333]
    tunnel: [w332] -> w14
    tunnel: [w331] -> w13
    tunnel: [w351] -> w68
    tunnel: w14 -> [w354]
    tunnel: w13 -> [w353]
    tunnel: [w352] -> w12
    tunnel: [w350] -> w11
    tunnel: [w363] -> w74
    tunnel: [w366] -> w75
    tunnel: w68 -> [w363]
    tunnel: w12 -> [w366]
    tunnel: w11 -> [w364]
    frame #0 {
      "Y Run Current %" <- 100 ("Run Current %")
      "Y Holding Current %" <- 50 ("Holding Current %")
    }
    frame #1 {
      "Y Backlash" <- 5000 ("Backlash2")
      "Y Backlash steps/sec" <- 10000 ("Value (Signaling)")
    }
    frame #2 {
      w304 = 0.21167 ("MM/rev")
      w307 = u32 20000 ("step/rev")
      w302 = 50000 ("Value (Signaling)")
      n119 = property on="Y Velocity SP step/sec" class="DigNum (strict)"("Minimum"=1.0 ("Data Entry Limits:Minimum")) -> ()  [unwired: 2 in, 2 out]
      n120 = property on="Y Scan Velocity SP mm/sec" class="DigNum (strict)"("Val(Sgnl)"=0.1 ("Value (Signaling)")) -> ()  [unwired: 2 in, 2 out]
      n121 = property on="Y Velocity SP step/sec" class="DigNum (strict)"("Val(Sgnl)"=w302) -> ()  [unwired: 2 in, 2 out]
      n122 = To Double Precision Float(number=w307) -> (double precision float=w306:dbl)
      n123 = To Double Precision Float(number=w302) -> (double precision float=w308:dbl)
      n124 = Divide(x=w308, y=w306) -> (x/y=w303:dbl)
      n125 = property on="Y Velocity SP step/sec" class="DigNum (strict)"("Maximum"=w308) -> ()  [unwired: 2 in, 2 out]
      n126 = Multiply(x=w303, y=w304) -> (x*y=w305:dbl)
      n127 = property on="Y Velocity SP mm/sec" class="DigNum (strict)"("Val(Sgnl)"=w305) -> ()  [unwired: 2 in, 2 out]
      "Y steps/rev" <- w307
      "Y mm/rev" <- w304
    }
    frame #3 {
      w311 = -750000 ("lower limit")
      w312 = 750000 ("upper limit")
      n128 = property on="Y Step SP" class="DigNum (strict)"("Minimum"=w311) -> ()  [unwired: 2 in, 2 out]
      n129 = property on="Y Step SP" class="DigNum (strict)"("Maximum"=w312) -> ()  [unwired: 2 in, 2 out]
      "Y MAXPOS" <- w312
      "Y MINPOS" <- w311
      "Y offset mm" <- 0.0 ("offset")
    }
    frame #4 {
      w321 = refnum<visa-resource-name> "COM4" ("COM PORT")
      w319 = u16 0 items=["None", "XON/XOFF", "RTS/CTS", "XON/XOFF & RTS/CTS", "DTR/DSR", "XON/XOFF & DTR/DSR"] ("flow control (0:none)")
      w318 = u16 10 items=["1.0"=10, "1.5"=15, "2.0"=20] ("stop bits (10: 1 bit)")
      # "Stop bits"
      n130 = call-poly "VISA Configure Serial Port"("VISA resource name"=w321, "timeout (10sec)"=u32 10000, "baud rate (9600)"=u32 9600, "data bits (8)"=u16 8, "parity (0:none)"=enum16{"None", "Odd", "Even", "Mark", "Space"}."None", "stop bits (10: 1 bit)"=w318, "flow control (0:none)"=w319) -> ("VISA resource name out"=w314:refnum<visa-resource-name>, "error out"=w313:errorcluster)  [unwired: 7 in]
      "Y COM PORT" <- w321
    }
    frame #5 {
      n131 = property on="Y Run Current %" class="DigNum (strict)"() -> ("Value"=w326:i32)  [unwired: 2 in, 2 out]
      n132 = Divide(x=w326, y=3.5) -> (x/y=w328:dbl)
      n133 = Number To Fractional String(number=w328) -> (F-format string=w329:string)  [unwired: 3 in]
      n134 = call "Applied Send Command.vi"("error in (no error)"=w324, "Extra"=w329, "Command"=T1."Change Current", "VISA resource name"=w325) -> ("error out"=w322:errorcluster, "VISA resource name out"=w323:refnum<visa-resource-name>)  [unwired: 3 in, 1 out]
    }
    frame #6 {
      # "VELOCITY"
      n135 = property on="Y steps/rev" class="DigNum (strict)"() -> ("Value"=w338:u32)  [unwired: 2 in, 2 out]
      n136 = property on="Y Velocity SP step/sec" class="DigNum (strict)"() -> ("Value"=w335:i32)  [unwired: 2 in, 2 out]
      n137 = Divide(x=w335, y=w338) -> (x/y=w337:dbl)
      n138 = Number To Fractional String(number=w337) -> (F-format string=w341:string)  [unwired: 3 in]
      n139 = call "Applied Send Command.vi"("error in (no error)"=w333, "Extra"=w341, "Command"=T1."Velocity Setting", "VISA resource name"=w334) -> ("error out"=w342:errorcluster, "VISA resource name out"=w349:refnum<visa-resource-name>)  [unwired: 3 in, 1 out]
      n140 = call "Time Delay36"("error in (no error)"=w342, "Delay Time (s)"=0.1) -> ("error out"=w347:errorcluster)  [unwired: 9 in]
      n141 = call "Applied Send Command.vi"("error in (no error)"=w347, "Extra"="", "Command"=T1."Velocity Setting", "VISA resource name"=w349) -> ("error out"=w331:errorcluster, "read buffer"=w345:string, "VISA resource name out"=w332:refnum<visa-resource-name>)  [unwired: 3 in]
      n142 = Fract/Exp String To Number(string=w345, offset=3) -> (number=w340:dbl)  [unwired: 2 in, 1 out]
      n143 = Multiply(x=w340, y=w338) -> (x*y=w339:dbl)
      n144 = property on="Y velocity PV step/sec" class="DigNum (strict)"("Val(Sgnl)"=w339) -> ()  [unwired: 2 in, 2 out]
    }
    frame #7 {
      # "GET CURRENT POSITION"
      n145 = call "Applied Send Command.vi"("error in (no error)"=w353, "Extra"="", "Command"=T1."Immediate Position?", "VISA resource name"=w354) -> ("error out"=w356:errorcluster, "read buffer"=w358:string, "VISA resource name out"=w352:refnum<visa-resource-name>)  [unwired: 3 in]
      n146 = call "Time Delay37"("error in (no error)"=w356, "Delay Time (s)"=0.1) -> ("error out"=w351:errorcluster)  [unwired: 9 in]
      n147 = Hexadecimal String To Number(string=w358, offset=3) -> (number=w350:u32)  [unwired: 1 in, 1 out]
    }
    frame #8 {
      n148 = property on="Y Step SP" class="DigNum (strict)"("Val(Sgnl)"=w364) -> ()  [unwired: 2 in, 2 out]
      n149 = property on="Y Step SP" class="DigNum (strict)"() -> ("Maximum"=w362:dbl)  [unwired: 2 in, 2 out]
      n150 = property on="Y Step SP" class="DigNum (strict)"() -> ("Minimum"=w361:dbl)  [unwired: 2 in, 2 out]
      n151 = In Range and Coerce(upper limit=w362, x=w364, lower limit=w361) -> (In Range?=w365:bool)  [unwired: 1 out]
      n152 = property on="Y in Range" class="Bool (strict)"("Val(Sgnl)"=w365) -> ()  [unwired: 2 in, 2 out]
    }
  }
  n153 = call-poly <vilib>:"Read From Spreadsheet File.vi"("file path (dialog if empty)"=path "S:/LV codes/SCL2/POS.TXT") -> ("first row"=w42:i64[])  [unwired: 6 in, 4 out]
  n154 = call-poly <vilib>:"Read From Spreadsheet File.vi"("file path (dialog if empty)"=path "S:/LV codes/SCL2/PRESET.TXT") -> ("all rows"=w30:string[][])  [unwired: 6 in, 4 out]
  n155 = Array To Cluster(array=w42) -> (cluster=w41:T3)
  n156 = Transpose 2D Array(2D array=w30) -> (transposed array=w31:string[][])
  n157 = Unbundle(w41) -> ("first row[0]"=w39:i64, "first row[1]"=w38:i64, "first row[2]"=w37:i64, "first row[3]"=w36:i64)  [unwired: 5 out]
  n158 = Delete From Array(array=w31, index (row)=0) -> (deleted portion=w32:string[], array with subset deleted=w34:string[][])  [unwired: 2 in]
  n159 = property on="Reset X Motor Steps" class="DigNum (strict)"("Val(Sgnl)"=w39) -> ()  [unwired: 2 in, 2 out]
  n160 = property on="Reset Y Motor Steps" class="DigNum (strict)"("Val(Sgnl)"=w38) -> ()  [unwired: 2 in, 2 out]
  n161 = property on="Reset Z Motor Steps" class="DigNum (strict)"("Val(Sgnl)"=w37) -> ()  [unwired: 2 in, 2 out]
  n162 = property on="Reset R Motor Steps" class="DigNum (strict)"("Val(Sgnl)"=w36) -> ()  [unwired: 2 in, 2 out]
  n163 = Transpose 2D Array(2D array=w34) -> (transposed array=w35:string[][])
  n164 = property on="Preset positions" class="Ring (strict)"("Strings []"=w32) -> ()  [unwired: 2 in, 2 out]
  n165 = Decimal String To Number(string=w35) -> (number=w33:i32[][])  [unwired: 2 in, 1 out]
  n166 = Initialize Array(w24, w24, 4 ("dimension size")) -> (w27:i32[][])
  n167 = Build Array (concatenate)(w27, w33) -> (→"Presets":i32[][])
  n168 = while {
    tunnel: w75 -> [w385]
    tunnel: w74 -> [w388]
    tunnel: [w389] -> w49
    tunnel: [w387] -> w50
    tunnel: w72 -> [w384]
    tunnel: w71 -> [w383]
    tunnel: [w382] -> w70
    tunnel: [w381] -> w69
    tunnel: w56 -> [w380]
    tunnel: w55 -> [w379]
    tunnel: [w378] -> w52
    tunnel: [w377] -> w51
    tunnel: w54 -> [w376]
    tunnel: w53 -> [w375]
    tunnel: [w374] -> w48
    tunnel: [w373] -> w47
    stop <- "stop" stop-if-true
    n169 = flat-sequence {
      frame #0 {
      }
      frame #1 {
      }
    }
    n170 = flat-sequence {
      frame #0 {
      }
      frame #1 {
      }
    }
    n171 = property on="Preset positions" class="Ring (strict)"() -> ("Strings []"=w369:string[])  [unwired: 2 in, 2 out]
    n172 = event shown="[0] Timeout" {
      selector: _ -> [_ _ _ _ _ _ _ _ _ _ _ _ _ _ _ _ _ _ _ _ _ _ _ _ _]
      dyn-events: _ -> [_ _ _ _ _ _ _ _ _ _ _ _ _ _ _ _ _ _ _ _ _ _ _ _ _]
      timeout: 200 -> [_ _ _ _ _ _ _ _ _ _ _ _ _ _ _ _ _ _ _ _ _ _ _ _ _]
      tunnel: w388 -> [w509 _ _ _ _ _ _ _ _ _ _ _ w1239 _ _ _ _ w1532 _ _ w1636 w1652 w1696 w1784 w1929]
      tunnel: [w508 _ _ _ _ _ _ _ _ _ _ _ w1245 _ _ _ _ w1530 _ _ w1636 w1650 w1698 w1778 w1927] -> w389
      tunnel: w385 -> [w447 _ _ _ _ _ _ _ _ _ _ _ w1240 _ _ _ _ w1531 _ _ w1637 w1653 w1697 w1785 w1930]
      tunnel: [w507 _ _ _ _ _ _ _ _ _ _ _ w1246 _ _ _ _ w1527 _ _ w1637 w1651 w1699 w1779 w1928] -> w387
      tunnel: w384 -> [w446 _ _ _ _ _ _ _ _ _ _ _ _ _ _ w1433 w1493 _ _ _ _ w1647 w1689 w1787 w1926]
      tunnel: w383 -> [w484 _ _ _ _ _ _ _ _ _ _ _ _ _ _ w1432 w1492 _ _ _ _ w1646 w1688 w1786 w1925]
      tunnel: [w483 _ _ _ _ _ _ _ _ _ _ _ _ _ _ w1431 w1491 _ _ _ _ w1649 w1687 w1773 w1924] -> w382
      tunnel: [w482 _ _ _ _ _ _ _ _ _ _ _ _ _ _ w1430 w1490 _ _ _ _ w1648 w1686 w1772 w1923] -> w381
      tunnel: w380 -> [w456 _ _ _ _ _ _ _ _ _ _ _ _ w1302 _ _ _ _ w1565 _ _ w1645 w1683 w1783 w1922]
      tunnel: w379 -> [w459 _ _ _ _ _ _ _ _ _ _ _ _ w1301 _ _ _ _ w1564 _ _ w1644 w1682 w1782 w1921]
      tunnel: [w458 _ _ _ _ _ _ _ _ _ _ _ _ w1299 _ _ _ _ w1562 _ _ w1643 w1681 w1777 w1918] -> w378
      tunnel: [w457 _ _ _ _ _ _ _ _ _ _ _ _ w1300 _ _ _ _ w1563 _ _ w1642 w1680 w1776 w1917] -> w377
      tunnel: w376 -> [w455 _ _ _ _ _ _ _ _ _ _ _ _ _ w1366 _ _ _ _ w1602 _ w1641 w1677 w1781 w1920]
      tunnel: w375 -> [w454 _ _ _ _ _ _ _ _ _ _ _ _ _ w1365 _ _ _ _ w1601 _ w1640 w1676 w1780 w1919]
      tunnel: [w453 _ _ _ _ _ _ _ _ _ _ _ _ _ w1363 _ _ _ _ w1600 _ w1639 w1675 w1775 w1916] -> w374
      tunnel: [w452 _ _ _ _ _ _ _ _ _ _ _ _ _ w1364 _ _ _ _ w1599 _ w1638 w1674 w1774 w1915] -> w373
      event #0 {
        n173 = event-data() -> ()  [unwired: 1 in, 2 out]
        n174 = flat-sequence {
          tunnel: [w618] -> w481
          tunnel: [w631] -> w480
          tunnel: [w641] -> w479
          tunnel: [w611] -> w478
          tunnel: w456 -> [w626]
          tunnel: w459 -> [w627]
          tunnel: w481 -> [w651]
          tunnel: [w651] -> w477
          tunnel: w480 -> [w650]
          tunnel: [w650] -> w476
          tunnel: w479 -> [w649]
          tunnel: [w649] -> w475
          tunnel: w478 -> [w646]
          tunnel: [w646] -> w474
          tunnel: w477 -> [w658]
          tunnel: [w659] -> w473
          tunnel: w476 -> [w661]
          tunnel: [w660] -> w472
          tunnel: w475 -> [w657]
          tunnel: [w656] -> w471
          tunnel: w474 -> [w656]
          tunnel: w473 -> [w671]
          tunnel: w472 -> [w672]
          tunnel: w471 -> [w674]
          tunnel: [w670] -> w457
          tunnel: [w669] -> w458
          frame #0 {
            w630 = 0.2 ("Delay Time (s)")
            n175 = property on="Z Step SP" class="DigNum (strict)"() -> ("Maximum"=w643:dbl)  [unwired: 2 in, 2 out]
            n176 = property on="Z Step SP" class="DigNum (strict)"() -> ("Minimum"=w645:dbl)  [unwired: 2 in, 2 out]
            n177 = property on="Z steps/rev" class="DigNum (strict)"() -> ("Value"=w639:u32)  [unwired: 2 in, 2 out]
            n178 = property on="Z offset mm" class="DigNum (strict)"() -> ("Value"=w635:dbl)  [unwired: 2 in, 2 out]
            n179 = To Long Integer(number=w643) -> (32bit integer=w642:i32)
            n180 = To Long Integer(number=w645) -> (32bit integer=w644:i32)
            n181 = To Double Precision Float(number=w639) -> (double precision float=w640:dbl)
            n182 = call "Applied Send Command.vi"("error in (no error)"=w627, "Command"=T1."Immediate Position?", "VISA resource name"=w626) -> ("error out"=w625:errorcluster, "read buffer"=w622:string, "VISA resource name out"=w620:refnum<visa-resource-name>)  [unwired: 4 in]
            n183 = call "Time Delay17"("error in (no error)"=w625, "Delay Time (s)"=w630) -> ("error out"=w610:errorcluster)  [unwired: 9 in]
            n184 = Hexadecimal String To Number(string=w622, offset=3) -> (number=w623:u32)  [unwired: 1 in, 1 out]
            n185 = To Long Integer(number=w623) -> (32bit integer=w633:i32)
            n186 = call "Applied Send Command.vi"("error in (no error)"=w610, "Command"=T1."Request Status", "VISA resource name"=w620) -> ("error out"=w619:errorcluster, "read buffer"=w615:string, "VISA resource name out"=w618:refnum<visa-resource-name>)  [unwired: 4 in]
            n187 = property on="Z Step PV" class="DigNum (strict)"("Val(Sgnl)"=w633) -> ()  [unwired: 2 in, 2 out]
            n188 = call "Time Delay16"("error in (no error)"=w619, "Delay Time (s)"=w630) -> ("error out"=w631:errorcluster)  [unwired: 9 in]
            n189 = String Subset(string=w615, offset (0)=0, length (rest)=1 ("length (rest)")) -> (substring=w612:string)
            n190 = In Range and Coerce(upper limit=w642, x=w633, lower limit=w644) -> (In Range?=w641:bool)  [unwired: 1 out]
            n191 = To Double Precision Float(number=w633) -> (double precision float=w634:dbl)
            n192 = Not Equal?(x=w612, y="R") -> (x != y?=w611:bool)
            n193 = Equal?(x=w612, y="R") -> (x = y?=w629:bool)
            n194 = property on="Z in Range" class="Bool (strict)"("Val(Sgnl)"=w641) -> ()  [unwired: 2 in, 2 out]
            n195 = property on="Z in Motion" class="Bool (strict)"("Val(Sgnl)"=w611) -> ()  [unwired: 2 in, 2 out]
            n196 = property on="Z Ready" class="Bool (strict)"("Val(Sgnl)"=w629) -> ()  [unwired: 2 in, 2 out]
            n197 = Divide(x=w634, y=w640) -> (x/y=w638:dbl)
            n198 = property on="Z mm/rev" class="DigNum (strict)"() -> ("Value"=w637:dbl)  [unwired: 2 in, 2 out]
            n199 = Multiply(x=w638, y=w637) -> (x*y=w636:dbl)
            n200 = Add(x=w636, y=w635) -> (x+y=w632:dbl)
            n201 = property on="Z Position mm PV" class="DigNum (strict)"("Val(Sgnl)"=w632) -> ()  [unwired: 2 in, 2 out]
          }
          frame #1 {
            n202 = property on="Z Scan" class="Bool (strict)"() -> ("Value"=w647:bool)  [unwired: 2 in, 2 out]
            n203 = Or(x=w646, y=w647) -> (x .or. y?=w648:bool)
            n204 = case shown="True" w648 {
              frame #0 {
                n205 = property on="Z Scan OK" class="Bool"("DisabledEnum"=T2."Enabled" ("Disabled")) -> ()  [unwired: 2 in, 2 out]
                n206 = property on="Z Go" class="Bool"("DisabledEnum"=T2."Enabled" ("Disabled")) -> ()  [unwired: 2 in, 2 out]
              }
              frame #1 {
                n207 = property on="Z Scan OK" class="Bool"("DisabledEnum"=T2."Disabled and Grayed Out" ("Disabled")) -> ()  [unwired: 2 in, 2 out]
                n208 = property on="Z Go" class="Bool"("DisabledEnum"=T2."Disabled and Grayed Out" ("Disabled")) -> ()  [unwired: 2 in, 2 out]
              }
            }
          }
          frame #2 {
            n209 = case shown="False" w657 {
              tunnel: w658 -> [w665 w668]
              tunnel: [w663 w668] -> w659
              tunnel: [w662 w667] -> w660
              tunnel: w661 -> [w664 w667]
              frame #0 {
                n210 = call "Applied Send Command.vi"("error in (no error)"=w664, "Command"=T1."Stop & Kill Buffer", "VISA resource name"=w665) -> ("error out"=w662:errorcluster, "VISA resource name out"=w663:refnum<visa-resource-name>)  [unwired: 4 in, 1 out]
              }
              frame #1 {
              }
            }
          }
          frame #3 {
            n211 = property on="Z Backlash corr" class="Bool (strict)"() -> ("Value"=w675:bool)  [unwired: 2 in, 2 out]
            n212 = Implies(1:w674, 2:w675) -> (0:w673:bool)
            n213 = case shown="False" w673 {
              tunnel: w672 -> [w676 w708]
              tunnel: w671 -> [w677 w709]
              tunnel: [w678 w708] -> w670
              tunnel: [w679 w709] -> w669
              frame #0 {
                w705 = 0.1 ("Delay Time (s)")
                # "Backlash"
                # "Backlash"
                n214 = property on="Z Backlash" class="DigNum (strict)"() -> ("Value"=w683:i32)  [unwired: 2 in, 2 out]
                n215 = property on="Z steps/rev" class="DigNum (strict)"() -> ("Value"=w681:u32)  [unwired: 2 in, 2 out]
                n216 = To Long Integer(number=w683) -> (32bit integer=w686:i32)
                n217 = property on="Z Backlash corr" class="Bool (strict)"("Val(Sgnl)"=FALSE ("Value (Signaling)")) -> ()  [unwired: 2 in, 2 out]
                n218 = Number To Decimal String(number=w683) -> (decimal integer string=w691:string)  [unwired: 1 in]
                n219 = property on="Z Backlash steps/sec" class="DigNum (strict)"() -> ("Value"=w682:i32)  [unwired: 2 in, 2 out]
                n220 = Negate(x=w686) -> (-x=w685:i32)
                n221 = Divide(x=w682, y=w681) -> (x/y=w706:dbl)
                n222 = Number To Decimal String(number=w685) -> (decimal integer string=w692:string)  [unwired: 1 in]
                n223 = Number To Fractional String(number=w706) -> (F-format string=w707:string)  [unwired: 3 in]
                n224 = call "Applied Send Command.vi"("error in (no error)"=w676, "Extra"=w707, "Command"=T1."Velocity Setting", "VISA resource name"=w677) -> ("error out"=w703:errorcluster, "VISA resource name out"=w696:refnum<visa-resource-name>)  [unwired: 3 in, 1 out]
                n225 = call "Time Delay47"("error in (no error)"=w703, "Delay Time (s)"=w705) -> ("error out"=w704:errorcluster)  [unwired: 9 in]
                n226 = call "Applied Send Command.vi"("error in (no error)"=w704, "Extra"=w691, "Command"=T1."Distance or Position", "VISA resource name"=w696) -> ("error out"=w697:errorcluster, "VISA resource name out"=w690:refnum<visa-resource-name>)  [unwired: 3 in, 1 out]
                n227 = call "Time Delay44"("error in (no error)"=w697, "Delay Time (s)"=w705) -> ("error out"=w698:errorcluster)  [unwired: 9 in]
                n228 = call "Applied Send Command.vi"("error in (no error)"=w698, "Command"=T1."Feed to Length", "VISA resource name"=w690) -> ("error out"=w699:errorcluster, "VISA resource name out"=w693:refnum<visa-resource-name>)  [unwired: 4 in, 1 out]
                n229 = call "Time Delay45"("error in (no error)"=w699, "Delay Time (s)"=w705) -> ("error out"=w700:errorcluster)  [unwired: 9 in]
                n230 = call "Applied Send Command.vi"("error in (no error)"=w700, "Extra"=w692, "Command"=T1."Distance or Position", "VISA resource name"=w693) -> ("error out"=w701:errorcluster, "VISA resource name out"=w694:refnum<visa-resource-name>)  [unwired: 3 in, 1 out]
                n231 = call "Time Delay46"("error in (no error)"=w701, "Delay Time (s)"=w705) -> ("error out"=w702:errorcluster)  [unwired: 9 in]
                n232 = call "Applied Send Command.vi"("error in (no error)"=w702, "Command"=T1."Feed to Length", "VISA resource name"=w694) -> ("error out"=w678:errorcluster, "VISA resource name out"=w679:refnum<visa-resource-name>)  [unwired: 4 in, 1 out]
              }
              frame #1 {
              }
            }
          }
        }
        n233 = flat-sequence {
          tunnel: [w519] -> w470
          tunnel: [w531] -> w469
          tunnel: [w541] -> w468
          tunnel: [w510] -> w467
          tunnel: w455 -> [w528]
          tunnel: w454 -> [w527]
          tunnel: w470 -> [w551]
          tunnel: [w551] -> w466
          tunnel: w469 -> [w550]
          tunnel: [w550] -> w465
          tunnel: w468 -> [w549]
          tunnel: [w549] -> w464
          tunnel: w467 -> [w546]
          tunnel: [w546] -> w463
          tunnel: w466 -> [w558]
          tunnel: [w559] -> w462
          tunnel: w465 -> [w561]
          tunnel: [w560] -> w461
          tunnel: w464 -> [w557]
          tunnel: [w556] -> w460
          tunnel: w463 -> [w556]
          tunnel: w462 -> [w571]
          tunnel: w461 -> [w572]
          tunnel: w460 -> [w574]
          tunnel: [w570] -> w452
          tunnel: [w569] -> w453
          frame #0 {
            w530 = 0.2 ("Delay Time (s)")
            n234 = property on="R Step SP" class="DigNum (strict)"() -> ("Maximum"=w543:dbl)  [unwired: 2 in, 2 out]
            n235 = property on="R Step SP" class="DigNum (strict)"() -> ("Minimum"=w545:dbl)  [unwired: 2 in, 2 out]
            n236 = property on="R steps/rev" class="DigNum (strict)"() -> ("Value"=w539:u32)  [unwired: 2 in, 2 out]
            n237 = property on="R offset deg" class="DigNum (strict)"() -> ("Value"=w535:dbl)  [unwired: 2 in, 2 out]
            n238 = To Long Integer(number=w543) -> (32bit integer=w542:i32)
            n239 = To Long Integer(number=w545) -> (32bit integer=w544:i32)
            n240 = To Double Precision Float(number=w539) -> (double precision float=w540:dbl)
            n241 = call "Applied Send Command.vi"("error in (no error)"=w527, "Command"=T1."Immediate Position?", "VISA resource name"=w528) -> ("error out"=w523:errorcluster, "read buffer"=w524:string, "VISA resource name out"=w521:refnum<visa-resource-name>)  [unwired: 4 in]
            n242 = call "Time Delay21"("error in (no error)"=w523, "Delay Time (s)"=w530) -> ("error out"=w520:errorcluster)  [unwired: 9 in]
            n243 = Hexadecimal String To Number(string=w524, offset=3) -> (number=w525:u32)  [unwired: 1 in, 1 out]
            n244 = To Long Integer(number=w525) -> (32bit integer=w533:i32)
            n245 = call "Applied Send Command.vi"("error in (no error)"=w520, "Command"=T1."Request Status", "VISA resource name"=w521) -> ("error out"=w518:errorcluster, "read buffer"=w515:string, "VISA resource name out"=w519:refnum<visa-resource-name>)  [unwired: 4 in]
            n246 = property on="R Step PV" class="DigNum (strict)"("Val(Sgnl)"=w533) -> ()  [unwired: 2 in, 2 out]
            n247 = call "Time Delay20"("error in (no error)"=w518, "Delay Time (s)"=w530) -> ("error out"=w531:errorcluster)  [unwired: 9 in]
            n248 = String Subset(string=w515, offset (0)=0, length (rest)=1 ("length (rest)")) -> (substring=w511:string)
            n249 = In Range and Coerce(upper limit=w542, x=w533, lower limit=w544) -> (In Range?=w541:bool)  [unwired: 1 out]
            n250 = To Double Precision Float(number=w533) -> (double precision float=w534:dbl)
            n251 = Not Equal?(x=w511, y="R") -> (x != y?=w510:bool)
            n252 = Equal?(x=w511, y="R") -> (x = y?=w512:bool)
            n253 = property on="R in Range" class="Bool (strict)"("Val(Sgnl)"=w541) -> ()  [unwired: 2 in, 2 out]
            n254 = property on="R in Motion" class="Bool (strict)"("Val(Sgnl)"=w510) -> ()  [unwired: 2 in, 2 out]
            n255 = property on="R Ready" class="Bool (strict)"("Val(Sgnl)"=w512) -> ()  [unwired: 2 in, 2 out]
            n256 = Divide(x=w534, y=w540) -> (x/y=w538:dbl)
            n257 = property on="R deg/rev" class="DigNum (strict)"() -> ("Value"=w537:dbl)  [unwired: 2 in, 2 out]
            n258 = Multiply(x=w538, y=w537) -> (x*y=w536:dbl)
            n259 = Add(x=w536, y=w535) -> (x+y=w532:dbl)
            n260 = property on="R Position deg PV" class="DigNum (strict)"("Val(Sgnl)"=w532) -> ()  [unwired: 2 in, 2 out]
          }
          frame #1 {
            n261 = property on="R Scan" class="Bool (strict)"() -> ("Value"=w547:bool)  [unwired: 2 in, 2 out]
            n262 = Or(x=w546, y=w547) -> (x .or. y?=w548:bool)
            n263 = case shown="True" w548 {
              frame #0 {
                n264 = property on="R Scan OK" class="Bool"("DisabledEnum"=T2."Enabled" ("Disabled")) -> ()  [unwired: 2 in, 2 out]
                n265 = property on="R Go" class="Bool"("DisabledEnum"=T2."Enabled" ("Disabled")) -> ()  [unwired: 2 in, 2 out]
              }
              frame #1 {
                n266 = property on="R Scan OK" class="Bool"("DisabledEnum"=T2."Disabled and Grayed Out" ("Disabled")) -> ()  [unwired: 2 in, 2 out]
                n267 = property on="R Go" class="Bool"("DisabledEnum"=T2."Disabled and Grayed Out" ("Disabled")) -> ()  [unwired: 2 in, 2 out]
              }
            }
          }
          frame #2 {
            n268 = case shown="False" w557 {
              tunnel: w558 -> [w565 w568]
              tunnel: [w563 w568] -> w559
              tunnel: [w562 w567] -> w560
              tunnel: w561 -> [w564 w567]
              frame #0 {
                n269 = call "Applied Send Command.vi"("error in (no error)"=w564, "Command"=T1."Stop & Kill Buffer", "VISA resource name"=w565) -> ("error out"=w562:errorcluster, "VISA resource name out"=w563:refnum<visa-resource-name>)  [unwired: 4 in, 1 out]
              }
              frame #1 {
              }
            }
          }
          frame #3 {
            n270 = property on="R Backlash corr" class="Bool (strict)"() -> ("Value"=w575:bool)  [unwired: 2 in, 2 out]
            n271 = Implies(1:w574, 2:w575) -> (0:w573:bool)
            n272 = case shown="False" w573 {
              tunnel: w572 -> [w579 w608]
              tunnel: w571 -> [w578 w609]
              tunnel: [w576 w608] -> w570
              tunnel: [w577 w609] -> w569
              frame #0 {
                w586 = 0.1 ("Delay Time (s)")
                # "Backlash"
                # "Backlash"
                n273 = property on="R Backlash" class="DigNum (strict)"() -> ("Value"=w580:i32)  [unwired: 2 in, 2 out]
                n274 = property on="R steps/rev" class="DigNum (strict)"() -> ("Value"=w581:u32)  [unwired: 2 in, 2 out]
                n275 = To Long Integer(number=w580) -> (32bit integer=w605:i32)
                n276 = property on="R Backlash corr" class="Bool (strict)"("Val(Sgnl)"=FALSE ("Value (Signaling)")) -> ()  [unwired: 2 in, 2 out]
                n277 = Number To Decimal String(number=w580) -> (decimal integer string=w600:string)  [unwired: 1 in]
                n278 = property on="R Backlash steps/sec" class="DigNum (strict)"() -> ("Value"=w583:i32)  [unwired: 2 in, 2 out]
                n279 = Negate(x=w605) -> (-x=w606:i32)
                n280 = Divide(x=w583, y=w581) -> (x/y=w582:dbl)
                n281 = Number To Decimal String(number=w606) -> (decimal integer string=w599:string)  [unwired: 1 in]
                n282 = Number To Fractional String(number=w582) -> (F-format string=w585:string)  [unwired: 3 in]
                n283 = call "Applied Send Command.vi"("error in (no error)"=w579, "Extra"=w585, "Command"=T1."Velocity Setting", "VISA resource name"=w578) -> ("error out"=w588:errorcluster, "VISA resource name out"=w595:refnum<visa-resource-name>)  [unwired: 3 in, 1 out]
                n284 = call "Time Delay49"("error in (no error)"=w588, "Delay Time (s)"=w586) -> ("error out"=w587:errorcluster)  [unwired: 9 in]
                n285 = call "Applied Send Command.vi"("error in (no error)"=w587, "Extra"=w600, "Command"=T1."Distance or Position", "VISA resource name"=w595) -> ("error out"=w594:errorcluster, "VISA resource name out"=w601:refnum<visa-resource-name>)  [unwired: 3 in, 1 out]
                n286 = call "Time Delay18"("error in (no error)"=w594, "Delay Time (s)"=w586) -> ("error out"=w593:errorcluster)  [unwired: 9 in]
                n287 = call "Applied Send Command.vi"("error in (no error)"=w593, "Command"=T1."Feed to Length", "VISA resource name"=w601) -> ("error out"=w592:errorcluster, "VISA resource name out"=w598:refnum<visa-resource-name>)  [unwired: 4 in, 1 out]
                n288 = call "Time Delay19"("error in (no error)"=w592, "Delay Time (s)"=w586) -> ("error out"=w591:errorcluster)  [unwired: 9 in]
                n289 = call "Applied Send Command.vi"("error in (no error)"=w591, "Extra"=w599, "Command"=T1."Distance or Position", "VISA resource name"=w598) -> ("error out"=w590:errorcluster, "VISA resource name out"=w597:refnum<visa-resource-name>)  [unwired: 3 in, 1 out]
                n290 = call "Time Delay48"("error in (no error)"=w590, "Delay Time (s)"=w586) -> ("error out"=w589:errorcluster)  [unwired: 9 in]
                n291 = call "Applied Send Command.vi"("error in (no error)"=w589, "Command"=T1."Feed to Length", "VISA resource name"=w597) -> ("error out"=w576:errorcluster, "VISA resource name out"=w577:refnum<visa-resource-name>)  [unwired: 4 in, 1 out]
              }
              frame #1 {
              }
            }
          }
        }
        n292 = property on="X Step PV" class="DigNum (strict)"() -> ("Value"=w423:i32)  [unwired: 2 in, 2 out]
        n293 = property on="Y Step PV" class="DigNum (strict)"() -> ("Value"=w422:i32)  [unwired: 2 in, 2 out]
        n294 = property on="X Step SP" class="DigNum (strict)"() -> ("Maximum"=w424:dbl)  [unwired: 2 in, 2 out]
        n295 = property on="X Step SP" class="DigNum (strict)"() -> ("Minimum"=w425:dbl)  [unwired: 2 in, 2 out]
        n296 = property on="Y Step SP" class="DigNum (strict)"() -> ("Maximum"=w429:dbl)  [unwired: 2 in, 2 out]
        n297 = property on="Y Step SP" class="DigNum (strict)"() -> ("Minimum"=w428:dbl)  [unwired: 2 in, 2 out]
        n298 = Absolute Value(x=w423) -> (abs(x)=w420:i32)
        n299 = Absolute Value(x=w422) -> (abs(x)=w421:i32)
        n300 = property on="X Position mm PV" class="DigNum (strict)"() -> ("Value"=w448:dbl)  [unwired: 2 in, 2 out]
        n301 = property on="Y Position mm PV" class="DigNum (strict)"() -> ("Value"=w441:dbl)  [unwired: 2 in, 2 out]
        n302 = property on="Z Position mm PV" class="DigNum (strict)"() -> ("Value"=w442:dbl)  [unwired: 2 in, 2 out]
        n303 = property on="R Position deg PV" class="DigNum (strict)"() -> ("Value"=w449:dbl)  [unwired: 2 in, 2 out]
        n304 = Subtract(x=w424, y=w425) -> (x-y=w426:dbl)
        n305 = Multiply(x=w420, y=w421) -> (x*y=w415:i32)
        n306 = Subtract(x=w429, y=w428) -> (x-y=w430:dbl)
        n307 = property on="Y Scan Length SP steps" class="DigNum (strict)"() -> ("Value"=w433:i32)  [unwired: 2 in, 2 out]
        n308 = property on="Z Scan Length SP steps" class="DigNum (strict)"() -> ("Value"=w434:i32)  [unwired: 2 in, 2 out]
        n309 = Divide(x=w430, y=2.0) -> (x/y=w418:dbl)
        n310 = Divide(x=w426, y=2.0) -> (x/y=w419:dbl)
        n311 = Divide(x=w433, y=w434) -> (x/y=w435:dbl)
        n312 = call "Build XY Graph"("Reset"=TRUE, "Y Input"=w441, "X Input"=w448) -> ("XY Graph"=→"XY Graph":cluster{"Y":dbl[], "Y":dbl[]}[])  [unwired: 7 in, 1 out]
        n313 = call "Build XY Graph2"("Reset"=TRUE, "Y Input"=w449, "X Input"=w442) -> ("XY Graph"=→"ZR Graph":cluster{"Y":dbl[], "Y":dbl[]}[])  [unwired: 7 in, 1 out]
        n314 = property on="Clear ZY" class="Bool (strict)"() -> ("Value"=w432:bool)  [unwired: 2 in, 2 out]
        n315 = Absolute Value(x=w418) -> (abs(x)=w416:dbl)
        n316 = Absolute Value(x=w419) -> (abs(x)=w417:dbl)
        n317 = call "Build XY Graph3"("Reset"=w432, "Y Input"=w441, "X Input"=w442) -> ("XY Graph"=→"ZY Graph":cluster{"Y":dbl[], "Y":dbl[]}[])  [unwired: 7 in, 1 out]
        n318 = Inverse Tangent(1:w435) -> (0:w436:dbl)
        n319 = Multiply(x=w416, y=w417) -> (x*y=w414:dbl)
        n320 = Divide(x=w436, y=6.283185307179586) -> (x/y=w437:dbl)
        n321 = Less Or Equal?(x=w415, y=w414) -> (x <= y?=w413:bool)
        n322 = Multiply(x=360.0, y=w437) -> (x*y=w440:dbl)
        n323 = property on="atan Y/Z" class="DigNum (strict)"("Val(Sgnl)"=w440) -> ()  [unwired: 2 in, 2 out]
        n324 = flat-sequence {
          tunnel: [w722] -> w495
          tunnel: [w733] -> w494
          tunnel: [w711] -> w493
          tunnel: [w718] -> w492
          tunnel: w446 -> [w729]
          tunnel: w484 -> [w717]
          tunnel: w424 -> [w713]
          tunnel: w425 -> [w712]
          tunnel: w413 -> [w710]
          tunnel: w495 -> [w753]
          tunnel: [w753] -> w491
          tunnel: w494 -> [w752]
          tunnel: [w752] -> w490
          tunnel: w493 -> [w751]
          tunnel: [w751] -> w489
          tunnel: w492 -> [w748]
          tunnel: [w748] -> w488
          tunnel: w491 -> [w762]
          tunnel: [w759] -> w487
          tunnel: w490 -> [w761]
          tunnel: [w760] -> w486
          tunnel: w489 -> [w758]
          tunnel: [w763] -> w485
          tunnel: w488 -> [w763]
          tunnel: w487 -> [w774]
          tunnel: w486 -> [w775]
          tunnel: w485 -> [w776]
          tunnel: [w773] -> w482
          tunnel: [w772] -> w483
          frame #0 {
            w732 = 0.2 ("Delay Time (s)")
            n325 = To Long Integer(number=w713) -> (32bit integer=w745:i32)
            n326 = To Long Integer(number=w712) -> (32bit integer=w746:i32)
            n327 = property on="X steps/rev" class="DigNum (strict)"() -> ("Value"=w742:u32)  [unwired: 2 in, 2 out]
            n328 = property on="X offset mm" class="DigNum (strict)"() -> ("Value"=w738:dbl)  [unwired: 2 in, 2 out]
            n329 = To Double Precision Float(number=w742) -> (double precision float=w743:dbl)
            n330 = call "Applied Send Command.vi"("error in (no error)"=w717, "Command"=T1."Immediate Position?", "VISA resource name"=w729) -> ("error out"=w727:errorcluster, "read buffer"=w728:string, "VISA resource name out"=w723:refnum<visa-resource-name>)  [unwired: 4 in]
            n331 = call "Time Delay12"("error in (no error)"=w727, "Delay Time (s)"=w732) -> ("error out"=w720:errorcluster)  [unwired: 9 in]
            n332 = Hexadecimal String To Number(string=w728, offset=3) -> (number=w734:u32)  [unwired: 1 in, 1 out]
            n333 = To Long Integer(number=w734) -> (32bit integer=w736:i32)
            n334 = call "Applied Send Command.vi"("error in (no error)"=w720, "Command"=T1."Request Status", "VISA resource name"=w723) -> ("error out"=w721:errorcluster, "read buffer"=w725:string, "VISA resource name out"=w722:refnum<visa-resource-name>)  [unwired: 4 in]
            n335 = property on="X Step PV" class="DigNum (strict)"("Val(Sgnl)"=w736) -> ()  [unwired: 2 in, 2 out]
            n336 = call "Time Delay11"("error in (no error)"=w721, "Delay Time (s)"=w732) -> ("error out"=w733:errorcluster)  [unwired: 9 in]
            n337 = String Subset(string=w725, offset (0)=0, length (rest)=1 ("length (rest)")) -> (substring=w714:string)
            n338 = In Range and Coerce(upper limit=w745, x=w736, lower limit=w746) -> (In Range?=w744:bool)  [unwired: 1 out]
            n339 = To Double Precision Float(number=w736) -> (double precision float=w737:dbl)
            n340 = Not Equal?(x=w714, y="R") -> (x != y?=w718:bool)
            n341 = Equal?(x=w714, y="R") -> (x = y?=w731:bool)
            n342 = property on="X  in Motion" class="Bool (strict)"("Val(Sgnl)"=w718) -> ()  [unwired: 2 in, 2 out]
            n343 = property on="X Ready" class="Bool (strict)"("Val(Sgnl)"=w731) -> ()  [unwired: 2 in, 2 out]
            n344 = Divide(x=w737, y=w743) -> (x/y=w741:dbl)
            n345 = And(x=w710, y=w744) -> (x .and. y?=w711:bool)
            n346 = property on="X  in Range" class="Bool (strict)"("Val(Sgnl)"=w711) -> ()  [unwired: 2 in, 2 out]
            n347 = property on="X mm/rev" class="DigNum (strict)"() -> ("Value"=w740:dbl)  [unwired: 2 in, 2 out]
            n348 = Multiply(x=w741, y=w740) -> (x*y=w739:dbl)
            n349 = Add(x=w739, y=w738) -> (x+y=w735:dbl)
            n350 = property on="X Position mm PV" class="DigNum (strict)"("Val(Sgnl)"=w735) -> ()  [unwired: 2 in, 2 out]
          }
          frame #1 {
            n351 = property on="X Scan" class="Bool (strict)"() -> ("Value"=w749:bool)  [unwired: 2 in, 2 out]
            n352 = Or(x=w748, y=w749) -> (x .or. y?=w750:bool)
            n353 = case shown="True" w750 {
              frame #0 {
                n354 = property on="X Scan OK" class="Bool"("DisabledEnum"=T2."Enabled" ("Disabled")) -> ()  [unwired: 2 in, 2 out]
                n355 = property on="X Go" class="Bool"("DisabledEnum"=T2."Enabled" ("Disabled")) -> ()  [unwired: 2 in, 2 out]
              }
              frame #1 {
                n356 = property on="X Scan OK" class="Bool"("DisabledEnum"=T2."Disabled and Grayed Out" ("Disabled")) -> ()  [unwired: 2 in, 2 out]
                n357 = property on="X Go" class="Bool"("DisabledEnum"=T2."Disabled and Grayed Out" ("Disabled")) -> ()  [unwired: 2 in, 2 out]
              }
            }
          }
          frame #2 {
            n358 = case shown="False" w758 {
              tunnel: w762 -> [w765 w770]
              tunnel: [w767 w770] -> w759
              tunnel: [w768 w769] -> w760
              tunnel: w761 -> [w764 w769]
              frame #0 {
                n359 = call "Applied Send Command.vi"("error in (no error)"=w764, "Command"=T1."Stop & Kill Buffer", "VISA resource name"=w765) -> ("error out"=w768:errorcluster, "VISA resource name out"=w767:refnum<visa-resource-name>)  [unwired: 4 in, 1 out]
              }
              frame #1 {
              }
            }
          }
          frame #3 {
            n360 = property on="X Backlash corr" class="Bool (strict)"() -> ("Value"=w777:bool)  [unwired: 2 in, 2 out]
            n361 = Implies(1:w776, 2:w777) -> (0:w771:bool)
            n362 = case shown="False" w771 {
              tunnel: w775 -> [w791 w810]
              tunnel: w774 -> [w792 w811]
              tunnel: [w794 w810] -> w773
              tunnel: [w793 w811] -> w772
              frame #0 {
                w782 = 0.1 ("Delay Time (s)")
                # "Backlash"
                n363 = property on="X Backlash" class="DigNum (strict)"() -> ("Value"=w797:i32)  [unwired: 2 in, 2 out]
                n364 = property on="X steps/rev" class="DigNum (strict)"() -> ("Value"=w780:u32)  [unwired: 2 in, 2 out]
                n365 = To Long Integer(number=w797) -> (32bit integer=w806:i32)
                n366 = property on="X Backlash corr" class="Bool (strict)"("Val(Sgnl)"=FALSE ("Value (Signaling)")) -> ()  [unwired: 2 in, 2 out]
                n367 = Number To Decimal String(number=w797) -> (decimal integer string=w801:string)  [unwired: 1 in]
                n368 = property on="X Backlash steps/sec" class="DigNum (strict)"() -> ("Value"=w781:i32)  [unwired: 2 in, 2 out]
                n369 = Negate(x=w806) -> (-x=w807:i32)
                n370 = Divide(x=w781, y=w780) -> (x/y=w779:dbl)
                n371 = Number To Decimal String(number=w807) -> (decimal integer string=w800:string)  [unwired: 1 in]
                n372 = Number To Fractional String(number=w779) -> (F-format string=w778:string)  [unwired: 3 in]
                n373 = call "Applied Send Command.vi"("error in (no error)"=w791, "Extra"=w778, "Command"=T1."Velocity Setting", "VISA resource name"=w792) -> ("error out"=w784:errorcluster, "VISA resource name out"=w795:refnum<visa-resource-name>)  [unwired: 3 in, 1 out]
                n374 = call "Time Delay35"("error in (no error)"=w784, "Delay Time (s)"=w782) -> ("error out"=w783:errorcluster)  [unwired: 9 in]
                n375 = call "Applied Send Command.vi"("error in (no error)"=w783, "Extra"=w801, "Command"=T1."Distance or Position", "VISA resource name"=w795) -> ("error out"=w790:errorcluster, "VISA resource name out"=w802:refnum<visa-resource-name>)  [unwired: 3 in, 1 out]
                n376 = call "Time Delay32"("error in (no error)"=w790, "Delay Time (s)"=w782) -> ("error out"=w789:errorcluster)  [unwired: 9 in]
                n377 = call "Applied Send Command.vi"("error in (no error)"=w789, "Command"=T1."Feed to Length", "VISA resource name"=w802) -> ("error out"=w788:errorcluster, "VISA resource name out"=w799:refnum<visa-resource-name>)  [unwired: 4 in, 1 out]
                n378 = call "Time Delay33"("error in (no error)"=w788, "Delay Time (s)"=w782) -> ("error out"=w787:errorcluster)  [unwired: 9 in]
                n379 = call "Applied Send Command.vi"("error in (no error)"=w787, "Extra"=w800, "Command"=T1."Distance or Position", "VISA resource name"=w799) -> ("error out"=w786:errorcluster, "VISA resource name out"=w798:refnum<visa-resource-name>)  [unwired: 3 in, 1 out]
                n380 = call "Time Delay34"("error in (no error)"=w786, "Delay Time (s)"=w782) -> ("error out"=w785:errorcluster)  [unwired: 9 in]
                n381 = call "Applied Send Command.vi"("error in (no error)"=w785, "Command"=T1."Feed to Length", "VISA resource name"=w798) -> ("error out"=w794:errorcluster, "VISA resource name out"=w793:refnum<visa-resource-name>)  [unwired: 4 in, 1 out]
              }
              frame #1 {
              }
            }
          }
        }
        n382 = flat-sequence {
          tunnel: w509 -> [w828]
          tunnel: w447 -> [w829]
          tunnel: [w825] -> w506
          tunnel: [w835] -> w504
          tunnel: [w814] -> w502
          tunnel: [w816] -> w500
          tunnel: w429 -> [w815]
          tunnel: w428 -> [w812]
          tunnel: w413 -> [w813]
          tunnel: w506 -> [w855]
          tunnel: [w855] -> w505
          tunnel: w504 -> [w854]
          tunnel: [w854] -> w503
          tunnel: w502 -> [w853]
          tunnel: [w853] -> w501
          tunnel: w500 -> [w850]
          tunnel: [w850] -> w496
          tunnel: w505 -> [w862]
          tunnel: [w863] -> w499
          tunnel: w503 -> [w865]
          tunnel: [w864] -> w498
          tunnel: w501 -> [w861]
          tunnel: [w860] -> w497
          tunnel: w496 -> [w860]
          tunnel: w499 -> [w875]
          tunnel: w498 -> [w876]
          tunnel: w497 -> [w878]
          tunnel: [w874] -> w508
          tunnel: [w873] -> w507
          frame #0 {
            w834 = 0.2 ("Delay Time (s)")
            n383 = To Long Integer(number=w815) -> (32bit integer=w847:i32)
            n384 = To Long Integer(number=w812) -> (32bit integer=w848:i32)
            n385 = property on="Y steps/rev" class="DigNum (strict)"() -> ("Value"=w844:u32)  [unwired: 2 in, 2 out]
            n386 = property on="Y offset mm" class="DigNum (strict)"() -> ("Value"=w840:dbl)  [unwired: 2 in, 2 out]
            n387 = To Double Precision Float(number=w844) -> (double precision float=w845:dbl)
            n388 = call "Applied Send Command.vi"("error in (no error)"=w828, "Command"=T1."Immediate Position?", "VISA resource name"=w829) -> ("error out"=w831:errorcluster, "read buffer"=w832:string, "VISA resource name out"=w826:refnum<visa-resource-name>)  [unwired: 4 in]
            n389 = call "Time Delay4"("error in (no error)"=w831, "Delay Time (s)"=w834) -> ("error out"=w824:errorcluster)  [unwired: 9 in]
            n390 = Hexadecimal String To Number(string=w832, offset=3) -> (number=w836:u32)  [unwired: 1 in, 1 out]
            n391 = To Long Integer(number=w836) -> (32bit integer=w838:i32)
            n392 = call "Applied Send Command.vi"("error in (no error)"=w824, "Command"=T1."Request Status", "VISA resource name"=w826) -> ("error out"=w823:errorcluster, "read buffer"=w820:string, "VISA resource name out"=w825:refnum<visa-resource-name>)  [unwired: 4 in]
            n393 = property on="Y Step PV" class="DigNum (strict)"("Val(Sgnl)"=w838) -> ()  [unwired: 2 in, 2 out]
            n394 = call "Time Delay3"("error in (no error)"=w823, "Delay Time (s)"=w834) -> ("error out"=w835:errorcluster)  [unwired: 9 in]
            n395 = String Subset(string=w820, offset (0)=0, length (rest)=1 ("length (rest)")) -> (substring=w818:string)
            n396 = In Range and Coerce(upper limit=w847, x=w838, lower limit=w848) -> (In Range?=w846:bool)  [unwired: 1 out]
            n397 = To Double Precision Float(number=w838) -> (double precision float=w839:dbl)
            n398 = Not Equal?(x=w818, y="R") -> (x != y?=w816:bool)
            n399 = Equal?(x=w818, y="R") -> (x = y?=w833:bool)
            n400 = property on="Y in Motion" class="Bool (strict)"("Val(Sgnl)"=w816) -> ()  [unwired: 2 in, 2 out]
            n401 = property on="Y Ready" class="Bool (strict)"("Val(Sgnl)"=w833) -> ()  [unwired: 2 in, 2 out]
            n402 = Divide(x=w839, y=w845) -> (x/y=w843:dbl)
            n403 = And(x=w846, y=w813) -> (x .and. y?=w814:bool)
            n404 = property on="Y in Range" class="Bool (strict)"("Val(Sgnl)"=w814) -> ()  [unwired: 2 in, 2 out]
            n405 = property on="Y mm/rev" class="DigNum (strict)"() -> ("Value"=w842:dbl)  [unwired: 2 in, 2 out]
            n406 = Multiply(x=w843, y=w842) -> (x*y=w841:dbl)
            n407 = Add(x=w841, y=w840) -> (x+y=w837:dbl)
            n408 = property on="Y Position mm PV" class="DigNum (strict)"("Val(Sgnl)"=w837) -> ()  [unwired: 2 in, 2 out]
          }
          frame #1 {
            n409 = property on="Y Scan" class="Bool (strict)"() -> ("Value"=w851:bool)  [unwired: 2 in, 2 out]
            n410 = Or(x=w850, y=w851) -> (x .or. y?=w852:bool)
            n411 = case shown="True" w852 {
              frame #0 {
                n412 = property on="Y Scan OK" class="Bool"("DisabledEnum"=T2."Enabled" ("Disabled")) -> ()  [unwired: 2 in, 2 out]
                n413 = property on="Y Go" class="Bool"("DisabledEnum"=T2."Enabled" ("Disabled")) -> ()  [unwired: 2 in, 2 out]
              }
              frame #1 {
                n414 = property on="Y Scan OK" class="Bool"("DisabledEnum"=T2."Disabled and Grayed Out" ("Disabled")) -> ()  [unwired: 2 in, 2 out]
                n415 = property on="Y Go" class="Bool"("DisabledEnum"=T2."Disabled and Grayed Out" ("Disabled")) -> ()  [unwired: 2 in, 2 out]
              }
            }
          }
          frame #2 {
            n416 = case shown="False" w861 {
              tunnel: w862 -> [w867 w872]
              tunnel: [w869 w872] -> w863
              tunnel: [w868 w871] -> w864
              tunnel: w865 -> [w866 w871]
              frame #0 {
                n417 = call "Applied Send Command.vi"("error in (no error)"=w866, "Command"=T1."Stop & Kill Buffer", "VISA resource name"=w867) -> ("error out"=w868:errorcluster, "VISA resource name out"=w869:refnum<visa-resource-name>)  [unwired: 4 in, 1 out]
              }
              frame #1 {
              }
            }
          }
          frame #3 {
            n418 = property on="Y Backlash corr" class="Bool (strict)"() -> ("Value"=w879:bool)  [unwired: 2 in, 2 out]
            n419 = Implies(1:w878, 2:w879) -> (0:w877:bool)
            n420 = case shown="False" w877 {
              tunnel: w876 -> [w882 w911]
              tunnel: w875 -> [w883 w912]
              tunnel: [w880 w911] -> w874
              tunnel: [w881 w912] -> w873
              frame #0 {
                w889 = 0.1 ("Delay Time (s)")
                # "Backlash"
                n421 = property on="Y Backlash" class="DigNum (strict)"() -> ("Value"=w884:i32)  [unwired: 2 in, 2 out]
                n422 = property on="Y steps/rev" class="DigNum (strict)"() -> ("Value"=w888:u32)  [unwired: 2 in, 2 out]
                n423 = To Long Integer(number=w884) -> (32bit integer=w907:i32)
                n424 = property on="Y Backlash corr" class="Bool (strict)"("Val(Sgnl)"=FALSE ("Value (Signaling)")) -> ()  [unwired: 2 in, 2 out]
                n425 = Number To Decimal String(number=w884) -> (decimal integer string=w902:string)  [unwired: 1 in]
                n426 = property on="Y Backlash steps/sec" class="DigNum (strict)"() -> ("Value"=w885:i32)  [unwired: 2 in, 2 out]
                n427 = Negate(x=w907) -> (-x=w908:i32)
                n428 = Divide(x=w885, y=w888) -> (x/y=w887:dbl)
                n429 = Number To Decimal String(number=w908) -> (decimal integer string=w901:string)  [unwired: 1 in]
                n430 = Number To Fractional String(number=w887) -> (F-format string=w886:string)  [unwired: 3 in]
                n431 = call "Applied Send Command.vi"("error in (no error)"=w882, "Extra"=w886, "Command"=T1."Velocity Setting", "VISA resource name"=w883) -> ("error out"=w891:errorcluster, "VISA resource name out"=w897:refnum<visa-resource-name>)  [unwired: 3 in, 1 out]
                n432 = call "Time Delay41"("error in (no error)"=w891, "Delay Time (s)"=w889) -> ("error out"=w890:errorcluster)  [unwired: 9 in]
                n433 = call "Applied Send Command.vi"("error in (no error)"=w890, "Extra"=w902, "Command"=T1."Distance or Position", "VISA resource name"=w897) -> ("error out"=w896:errorcluster, "VISA resource name out"=w903:refnum<visa-resource-name>)  [unwired: 3 in, 1 out]
                n434 = call "Time Delay38"("error in (no error)"=w896, "Delay Time (s)"=w889) -> ("error out"=w895:errorcluster)  [unwired: 9 in]
                n435 = call "Applied Send Command.vi"("error in (no error)"=w895, "Command"=T1."Feed to Length", "VISA resource name"=w903) -> ("error out"=w894:errorcluster, "VISA resource name out"=w900:refnum<visa-resource-name>)  [unwired: 4 in, 1 out]
                n436 = call "Applied Send Command.vi"("Extra"=w901, "Command"=T1."Distance or Position", "VISA resource name"=w900) -> ("error out"=w893:errorcluster, "VISA resource name out"=w899:refnum<visa-resource-name>)  [unwired: 4 in, 1 out]
                n437 = call "Time Delay39"("error in (no error)"=w894, "Delay Time (s)"=w889) -> ()  [unwired: 9 in, 1 out]
                n438 = call "Time Delay40"("error in (no error)"=w893, "Delay Time (s)"=w889) -> ("error out"=w892:errorcluster)  [unwired: 9 in]
                n439 = call "Applied Send Command.vi"("error in (no error)"=w892, "Command"=T1."Feed to Length", "VISA resource name"=w899) -> ("error out"=w880:errorcluster, "VISA resource name out"=w881:refnum<visa-resource-name>)  [unwired: 4 in, 1 out]
              }
              frame #1 {
              }
            }
          }
        }
      }
      event #1 {
        n440 = event-data() -> ()  [unwired: 1 in, 5 out]
        n441 = property on="Z steps/rev" class="DigNum (strict)"() -> ("Value"=w924:u32)  [unwired: 2 in, 2 out]
        n442 = property on="R steps/rev" class="DigNum (strict)"() -> ("Value"=w915:u32)  [unwired: 2 in, 2 out]
        n443 = property on="X steps/rev" class="DigNum (strict)"() -> ("Value"=w933:u32)  [unwired: 2 in, 2 out]
        n444 = property on="Y steps/rev" class="DigNum (strict)"() -> ("Value"=w942:u32)  [unwired: 2 in, 2 out]
        n445 = property on="Z offset mm" class="DigNum (strict)"() -> ("Value"=w922:dbl)  [unwired: 2 in, 2 out]
        n446 = property on="R offset deg" class="DigNum (strict)"() -> ("Value"=w913:dbl)  [unwired: 2 in, 2 out]
        n447 = property on="X offset mm" class="DigNum (strict)"() -> ("Value"=w931:dbl)  [unwired: 2 in, 2 out]
        n448 = property on="Y offset mm" class="DigNum (strict)"() -> ("Value"=w940:dbl)  [unwired: 2 in, 2 out]
        n449 = property on="Reset R Position deg" class="DigNum (strict)"() -> ("Value"=w921:dbl)  [unwired: 2 in, 2 out]
        n450 = property on="Reset Z Position mm" class="DigNum (strict)"() -> ("Value"=w930:dbl)  [unwired: 2 in, 2 out]
        n451 = property on="Reset X Position mm" class="DigNum (strict)"() -> ("Value"=w939:dbl)  [unwired: 2 in, 2 out]
        n452 = property on="Reset Y Position mm" class="DigNum (strict)"() -> ("Value"=w948:dbl)  [unwired: 2 in, 2 out]
        n453 = To Double Precision Float(number=w915) -> (double precision float=w918:dbl)
        n454 = To Double Precision Float(number=w924) -> (double precision float=w927:dbl)
        n455 = To Double Precision Float(number=w933) -> (double precision float=w936:dbl)
        n456 = To Double Precision Float(number=w942) -> (double precision float=w945:dbl)
        n457 = Subtract(x=w930, y=w922) -> (x-y=w929:dbl)
        n458 = Subtract(x=w921, y=w913) -> (x-y=w920:dbl)
        n459 = Subtract(x=w939, y=w931) -> (x-y=w938:dbl)
        n460 = Subtract(x=w948, y=w940) -> (x-y=w947:dbl)
        n461 = property on="R deg/rev" class="DigNum (strict)"() -> ("Value"=w914:dbl)  [unwired: 2 in, 2 out]
        n462 = property on="Z mm/rev" class="DigNum (strict)"() -> ("Value"=w923:dbl)  [unwired: 2 in, 2 out]
        n463 = property on="X mm/rev" class="DigNum (strict)"() -> ("Value"=w932:dbl)  [unwired: 2 in, 2 out]
        n464 = property on="Y mm/rev" class="DigNum (strict)"() -> ("Value"=w941:dbl)  [unwired: 2 in, 2 out]
        n465 = Divide(x=w929, y=w923) -> (x/y=w928:dbl)
        n466 = Divide(x=w920, y=w914) -> (x/y=w919:dbl)
        n467 = Divide(x=w938, y=w932) -> (x/y=w937:dbl)
        n468 = Divide(x=w947, y=w941) -> (x/y=w946:dbl)
        n469 = Multiply(x=w928, y=w927) -> (x*y=w926:dbl)
        n470 = Multiply(x=w919, y=w918) -> (x*y=w917:dbl)
        n471 = Multiply(x=w937, y=w936) -> (x*y=w935:dbl)
        n472 = Multiply(x=w946, y=w945) -> (x*y=w944:dbl)
        n473 = To Long Integer(number=w926) -> (32bit integer=w925:i32)
        n474 = To Long Integer(number=w917) -> (32bit integer=w916:i32)
        n475 = To Long Integer(number=w935) -> (32bit integer=w934:i32)
        n476 = To Long Integer(number=w944) -> (32bit integer=w943:i32)
        n477 = property on="Reset Z Motor Steps" class="DigNum (strict)"("Val(Sgnl)"=w925) -> ()  [unwired: 2 in, 2 out]
        n478 = property on="Reset R Motor Steps" class="DigNum (strict)"("Val(Sgnl)"=w916) -> ()  [unwired: 2 in, 2 out]
        n479 = property on="Reset X Motor Steps" class="DigNum (strict)"("Val(Sgnl)"=w934) -> ()  [unwired: 2 in, 2 out]
        n480 = property on="Reset Y Motor Steps" class="DigNum (strict)"("Val(Sgnl)"=w943) -> ()  [unwired: 2 in, 2 out]
      }
      event #2 {
        n481 = event-data() -> ()  [unwired: 1 in, 5 out]
        n482 = property on="Y Step SP" class="DigNum (strict)"() -> ("Value"=w981:i32)  [unwired: 2 in, 2 out]
        n483 = property on="X Step SP" class="DigNum (strict)"() -> ("Value"=w973:i32)  [unwired: 2 in, 2 out]
        n484 = property on="Z Step SP" class="DigNum (strict)"() -> ("Value"=w965:i32)  [unwired: 2 in, 2 out]
        n485 = property on="R Step SP" class="DigNum (strict)"() -> ("Value"=w957:i32)  [unwired: 2 in, 2 out]
        n486 = property on="Y steps/rev" class="DigNum (strict)"() -> ("Value"=w1004:u32)  [unwired: 2 in, 2 out]
        n487 = property on="Y steps/rev" class="DigNum (strict)"() -> ("Value"=w979:u32)  [unwired: 2 in, 2 out]
        n488 = property on="X steps/rev" class="DigNum (strict)"() -> ("Value"=w998:u32)  [unwired: 2 in, 2 out]
        n489 = property on="X steps/rev" class="DigNum (strict)"() -> ("Value"=w971:u32)  [unwired: 2 in, 2 out]
        n490 = property on="Z steps/rev" class="DigNum (strict)"() -> ("Value"=w992:u32)  [unwired: 2 in, 2 out]
        n491 = property on="Z steps/rev" class="DigNum (strict)"() -> ("Value"=w963:u32)  [unwired: 2 in, 2 out]
        n492 = property on="R steps/rev" class="DigNum (strict)"() -> ("Value"=w986:u32)  [unwired: 2 in, 2 out]
        n493 = property on="R steps/rev" class="DigNum (strict)"() -> ("Value"=w955:u32)  [unwired: 2 in, 2 out]
        n494 = property on="Y offset mm" class="DigNum (strict)"() -> ("Value"=w978:dbl)  [unwired: 2 in, 2 out]
        n495 = property on="X offset mm" class="DigNum (strict)"() -> ("Value"=w970:dbl)  [unwired: 2 in, 2 out]
        n496 = property on="Z offset mm" class="DigNum (strict)"() -> ("Value"=w962:dbl)  [unwired: 2 in, 2 out]
        n497 = property on="R offset deg" class="DigNum (strict)"() -> ("Value"=w954:dbl)  [unwired: 2 in, 2 out]
        n498 = property on="Y Velocity SP step/sec" class="DigNum (strict)"() -> ("Value"=w1006:i32)  [unwired: 2 in, 2 out]
        n499 = property on="X Velocity SP step/sec" class="DigNum (strict)"() -> ("Value"=w1000:i32)  [unwired: 2 in, 2 out]
        n500 = property on="Z Velocity SP step/sec" class="DigNum (strict)"() -> ("Value"=w994:i32)  [unwired: 2 in, 2 out]
        n501 = property on="R Velocity SP step/sec" class="DigNum (strict)"() -> ("Value"=w988:i32)  [unwired: 2 in, 2 out]
        n502 = To Double Precision Float(number=w981) -> (double precision float=w982:dbl)
        n503 = To Double Precision Float(number=w979) -> (double precision float=w985:dbl)
        n504 = To Double Precision Float(number=w998) -> (double precision float=w1003:dbl)
        n505 = To Double Precision Float(number=w973) -> (double precision float=w974:dbl)
        n506 = To Double Precision Float(number=w971) -> (double precision float=w977:dbl)
        n507 = To Double Precision Float(number=w992) -> (double precision float=w997:dbl)
        n508 = To Double Precision Float(number=w965) -> (double precision float=w966:dbl)
        n509 = To Double Precision Float(number=w963) -> (double precision float=w969:dbl)
        n510 = To Double Precision Float(number=w986) -> (double precision float=w991:dbl)
        n511 = To Double Precision Float(number=w957) -> (double precision float=w958:dbl)
        n512 = To Double Precision Float(number=w955) -> (double precision float=w961:dbl)
        n513 = Divide(x=w958, y=w961) -> (x/y=w960:dbl)
        n514 = Divide(x=w982, y=w985) -> (x/y=w984:dbl)
        n515 = Divide(x=w974, y=w977) -> (x/y=w976:dbl)
        n516 = Divide(x=w966, y=w969) -> (x/y=w968:dbl)
        n517 = To Double Precision Float(number=w988) -> (double precision float=w989:dbl)
        n518 = To Double Precision Float(number=w1006) -> (double precision float=w1007:dbl)
        n519 = To Double Precision Float(number=w1004) -> (double precision float=w1009:dbl)
        n520 = To Double Precision Float(number=w1000) -> (double precision float=w1001:dbl)
        n521 = To Double Precision Float(number=w994) -> (double precision float=w995:dbl)
        n522 = property on="R deg/rev" class="DigNum (strict)"() -> ("Value"=w953:dbl)  [unwired: 2 in, 2 out]
        n523 = property on="Y mm/rev" class="DigNum (strict)"() -> ("Value"=w950:dbl)  [unwired: 2 in, 2 out]
        n524 = property on="X mm/rev" class="DigNum (strict)"() -> ("Value"=w951:dbl)  [unwired: 2 in, 2 out]
        n525 = property on="Z mm/rev" class="DigNum (strict)"() -> ("Value"=w952:dbl)  [unwired: 2 in, 2 out]
        n526 = Divide(x=w1007, y=w1009) -> (x/y=w1008:dbl)
        n527 = Multiply(x=w984, y=w950) -> (x*y=w983:dbl)
        n528 = Divide(x=w1001, y=w1003) -> (x/y=w1002:dbl)
        n529 = Multiply(x=w976, y=w951) -> (x*y=w975:dbl)
        n530 = Divide(x=w995, y=w997) -> (x/y=w996:dbl)
        n531 = Multiply(x=w968, y=w952) -> (x*y=w967:dbl)
        n532 = Divide(x=w989, y=w991) -> (x/y=w990:dbl)
        n533 = Multiply(x=w960, y=w953) -> (x*y=w959:dbl)
        n534 = Multiply(x=w1008, y=w950) -> (x*y=w1005:dbl)
        n535 = Add(x=w983, y=w978) -> (x+y=w980:dbl)
        n536 = Multiply(x=w1002, y=w951) -> (x*y=w999:dbl)
        n537 = Add(x=w975, y=w970) -> (x+y=w972:dbl)
        n538 = Multiply(x=w996, y=w952) -> (x*y=w993:dbl)
        n539 = Add(x=w967, y=w962) -> (x+y=w964:dbl)
        n540 = Multiply(x=w990, y=w953) -> (x*y=w987:dbl)
        n541 = Add(x=w959, y=w954) -> (x+y=w956:dbl)
        n542 = Absolute Value(x=w987) -> (abs(x)=w949:dbl)
        n543 = property on="Y Velocity MV mm/sec" class="DigNum (strict)"("Val(Sgnl)"=w1005) -> ()  [unwired: 2 in, 2 out]
        n544 = property on="Y Position MV mm" class="DigNum (strict)"("Val(Sgnl)"=w980) -> ()  [unwired: 2 in, 2 out]
        n545 = property on="X Velocity MV mm/sec" class="DigNum (strict)"("Val(Sgnl)"=w999) -> ()  [unwired: 2 in, 2 out]
        n546 = property on="X Position MV mm" class="DigNum (strict)"("Val(Sgnl)"=w972) -> ()  [unwired: 2 in, 2 out]
        n547 = property on="Z Velocity MV mm/sec" class="DigNum (strict)"("Val(Sgnl)"=w993) -> ()  [unwired: 2 in, 2 out]
        n548 = property on="Z Position MV mm" class="DigNum (strict)"("Val(Sgnl)"=w964) -> ()  [unwired: 2 in, 2 out]
        n549 = property on="R Position MV deg" class="DigNum (strict)"("Val(Sgnl)"=w956) -> ()  [unwired: 2 in, 2 out]
        n550 = property on="R Velocity MVdeg/sec" class="DigNum (strict)"("Val(Sgnl)"=w949) -> ()  [unwired: 2 in, 2 out]
      }
      event #3 {
        n551 = event-data() -> ()  [unwired: 1 in, 5 out]
        n552 = property on="X Step PV" class="DigNum (strict)"() -> ("Value"=w1078:i32)  [unwired: 2 in, 2 out]
        n553 = property on="Y Step PV" class="DigNum (strict)"() -> ("Value"=w1064:i32)  [unwired: 2 in, 2 out]
        n554 = property on="Z Step PV" class="DigNum (strict)"() -> ("Value"=w1051:i32)  [unwired: 2 in, 2 out]
        n555 = property on="R Step PV" class="DigNum (strict)"() -> ("Value"=w1037:i32)  [unwired: 2 in, 2 out]
        n556 = property on="X Step SP" class="DigNum (strict)"() -> ("Minimum"=w1085:dbl)  [unwired: 2 in, 2 out]
        n557 = property on="X Step SP" class="DigNum (strict)"() -> ("Maximum"=w1084:dbl)  [unwired: 2 in, 2 out]
        n558 = property on="Y Step SP" class="DigNum (strict)"() -> ("Minimum"=w1071:dbl)  [unwired: 2 in, 2 out]
        n559 = property on="Y Step SP" class="DigNum (strict)"() -> ("Maximum"=w1070:dbl)  [unwired: 2 in, 2 out]
        n560 = property on="Z Step SP" class="DigNum (strict)"() -> ("Minimum"=w1058:dbl)  [unwired: 2 in, 2 out]
        n561 = property on="Z Step SP" class="DigNum (strict)"() -> ("Maximum"=w1057:dbl)  [unwired: 2 in, 2 out]
        n562 = property on="R Step SP" class="DigNum (strict)"() -> ("Minimum"=w1042:dbl)  [unwired: 2 in, 2 out]
        n563 = property on="R Step SP" class="DigNum (strict)"() -> ("Maximum"=w1045:dbl)  [unwired: 2 in, 2 out]
        n564 = property on="Z steps/rev" class="DigNum (strict)"() -> ("Value"=w1053:u32)  [unwired: 2 in, 2 out]
        n565 = property on="R steps/rev" class="DigNum (strict)"() -> ("Value"=w1039:u32)  [unwired: 2 in, 2 out]
        n566 = property on="X steps/rev" class="DigNum (strict)"() -> ("Value"=w1080:u32)  [unwired: 2 in, 2 out]
        n567 = property on="Y steps/rev" class="DigNum (strict)"() -> ("Value"=w1066:u32)  [unwired: 2 in, 2 out]
        n568 = To Double Precision Float(number=w1078) -> (double precision float=w1031:dbl)
        n569 = To Double Precision Float(number=w1064) -> (double precision float=w1030:dbl)
        n570 = To Double Precision Float(number=w1051) -> (double precision float=w1029:dbl)
        n571 = To Double Precision Float(number=w1037) -> (double precision float=w1028:dbl)
        n572 = Subtract(x=w1085, y=w1031) -> (x-y=w1086:dbl)
        n573 = Subtract(x=w1084, y=w1031) -> (x-y=w1083:dbl)
        n574 = Subtract(x=w1071, y=w1030) -> (x-y=w1072:dbl)
        n575 = Subtract(x=w1070, y=w1030) -> (x-y=w1069:dbl)
        n576 = Subtract(x=w1058, y=w1029) -> (x-y=w1059:dbl)
        n577 = Subtract(x=w1057, y=w1029) -> (x-y=w1056:dbl)
        n578 = Subtract(x=w1042, y=w1028) -> (x-y=w1043:dbl)
        n579 = Subtract(x=w1045, y=w1028) -> (x-y=w1044:dbl)
        n580 = property on="Z Scan Length SP steps" class="DigNum (strict)"() -> ("Value"=w1054:i32)  [unwired: 2 in, 2 out]
        n581 = To Double Precision Float(number=w1053) -> (double precision float=w1050:dbl)
        n582 = property on="R Scan Length SP steps" class="DigNum (strict)"() -> ("Value"=w1040:i32)  [unwired: 2 in, 2 out]
        n583 = To Double Precision Float(number=w1039) -> (double precision float=w1036:dbl)
        n584 = property on="X Scan Length SP steps" class="DigNum (strict)"() -> ("Value"=w1076:i32)  [unwired: 2 in, 2 out]
        n585 = To Double Precision Float(number=w1080) -> (double precision float=w1077:dbl)
        n586 = property on="Y Scan Length SP steps" class="DigNum (strict)"() -> ("Value"=w1067:i32)  [unwired: 2 in, 2 out]
        n587 = To Double Precision Float(number=w1066) -> (double precision float=w1021:dbl)
        n588 = property on="Z Scan Velocity SP steps/sec" class="DigNum (strict)"() -> ("Value"=w1049:i32)  [unwired: 2 in, 2 out]
        n589 = property on="R Scan Velocity SP steps/sec" class="DigNum (strict)"() -> ("Value"=w1035:i32)  [unwired: 2 in, 2 out]
        n590 = property on="X Scan Velocity SP steps/sec" class="DigNum (strict)"() -> ("Value"=w1081:i32)  [unwired: 2 in, 2 out]
        n591 = property on="Y Scan Velocity SP steps/sec" class="DigNum (strict)"() -> ("Value"=w1063:i32)  [unwired: 2 in, 2 out]
        n592 = To Double Precision Float(number=w1054) -> (double precision float=w1027:dbl)
        n593 = To Double Precision Float(number=w1040) -> (double precision float=w1025:dbl)
        n594 = property on="X Scan Length SP steps" class="DigNum (strict)"("Minimum"=w1086) -> ()  [unwired: 2 in, 2 out]
        n595 = property on="X Scan Length SP steps" class="DigNum (strict)"("Maximum"=w1083) -> ()  [unwired: 2 in, 2 out]
        n596 = property on="Y Scan Length SP steps" class="DigNum (strict)"("Minimum"=w1072) -> ()  [unwired: 2 in, 2 out]
        n597 = property on="Y Scan Length SP steps" class="DigNum (strict)"("Maximum"=w1069) -> ()  [unwired: 2 in, 2 out]
        n598 = property on="Z Scan Length SP steps" class="DigNum (strict)"("Minimum"=w1059) -> ()  [unwired: 2 in, 2 out]
        n599 = property on="Z Scan Length SP steps" class="DigNum (strict)"("Maximum"=w1056) -> ()  [unwired: 2 in, 2 out]
        n600 = property on="R Scan Length SP steps" class="DigNum (strict)"("Minimum"=w1043) -> ()  [unwired: 2 in, 2 out]
        n601 = property on="R Scan Length SP steps" class="DigNum (strict)"("Maximum"=w1044) -> ()  [unwired: 2 in, 2 out]
        n602 = To Double Precision Float(number=w1076) -> (double precision float=w1016:dbl)
        n603 = To Double Precision Float(number=w1067) -> (double precision float=w1020:dbl)
        n604 = Divide(x=w1025, y=w1036) -> (x/y=w1041:dbl)
        n605 = Divide(x=w1027, y=w1050) -> (x/y=w1055:dbl)
        n606 = Divide(x=w1016, y=w1077) -> (x/y=w1075:dbl)
        n607 = Divide(x=w1020, y=w1021) -> (x/y=w1068:dbl)
        n608 = To Double Precision Float(number=w1035) -> (double precision float=w1024:dbl)
        n609 = property on="R deg/rev" class="DigNum (strict)"() -> ("Value"=w1038:dbl)  [unwired: 2 in, 2 out]
        n610 = To Double Precision Float(number=w1049) -> (double precision float=w1026:dbl)
        n611 = To Double Precision Float(number=w1081) -> (double precision float=w1015:dbl)
        n612 = To Double Precision Float(number=w1063) -> (double precision float=w1019:dbl)
        n613 = property on="Z mm/rev" class="DigNum (strict)"() -> ("Value"=w1052:dbl)  [unwired: 2 in, 2 out]
        n614 = property on="X mm/rev" class="DigNum (strict)"() -> ("Value"=w1079:dbl)  [unwired: 2 in, 2 out]
        n615 = property on="Y mm/rev" class="DigNum (strict)"() -> ("Value"=w1065:dbl)  [unwired: 2 in, 2 out]
        n616 = Multiply(x=w1055, y=w1052) -> (x*y=w1047:dbl)
        n617 = Divide(x=w1027, y=w1026) -> (x/y=w1022:dbl)
        n618 = Divide(x=w1026, y=w1050) -> (x/y=w1048:dbl)
        n619 = Multiply(x=w1041, y=w1038) -> (x*y=w1033:dbl)
        n620 = Divide(x=w1025, y=w1024) -> (x/y=w1023:dbl)
        n621 = Divide(x=w1024, y=w1036) -> (x/y=w1034:dbl)
        n622 = Multiply(x=w1079, y=w1075) -> (x*y=w1073:dbl)
        n623 = Divide(x=w1016, y=w1015) -> (x/y=w1017:dbl)
        n624 = Divide(x=w1015, y=w1077) -> (x/y=w1082:dbl)
        n625 = Multiply(x=w1068, y=w1065) -> (x*y=w1061:dbl)
        n626 = Divide(x=w1020, y=w1019) -> (x/y=w1018:dbl)
        n627 = Divide(x=w1019, y=w1021) -> (x/y=w1062:dbl)
        n628 = Multiply(x=w1052, y=w1048) -> (x*y=w1046:dbl)
        n629 = Multiply(x=w1038, y=w1034) -> (x*y=w1032:dbl)
        n630 = Multiply(x=w1082, y=w1079) -> (x*y=w1074:dbl)
        n631 = Multiply(x=w1065, y=w1062) -> (x*y=w1060:dbl)
        n632 = Absolute Value(x=w1022) -> (abs(x)=→"Z Scan Duration":dbl)
        n633 = Absolute Value(x=w1023) -> (abs(x)=→"R Scan Duration":dbl)
        n634 = Absolute Value(x=w1017) -> (abs(x)=→"X Scan Duration":dbl)
        n635 = Absolute Value(x=w1018) -> (abs(x)=→"Y Scan Duration":dbl)
        n636 = property on="Z Scan length MV mm" class="DigNum (strict)"("Value"=w1047) -> ()  [unwired: 2 in, 2 out]
        n637 = property on="R Scan length MV deg" class="DigNum (strict)"("Value"=w1033) -> ()  [unwired: 2 in, 2 out]
        n638 = property on="X Scan length MV mm" class="DigNum (strict)"("Val(Sgnl)"=w1073) -> ()  [unwired: 2 in, 2 out]
        n639 = property on="Y Scan length MV mm" class="DigNum (strict)"("Value"=w1061) -> ()  [unwired: 2 in, 2 out]
        n640 = Absolute Value(x=w1032) -> (abs(x)=w1014:dbl)
        n641 = property on="Z Scan velocity MV mm/sec" class="DigNum (strict)"("Val(Sgnl)"=w1046) -> ()  [unwired: 2 in, 2 out]
        n642 = property on="X Scan velocity MV mm/sec" class="DigNum (strict)"("Value"=w1074) -> ()  [unwired: 2 in, 2 out]
        n643 = property on="Y Scan velocity MV mm/sec" class="DigNum (strict)"("Val(Sgnl)"=w1060) -> ()  [unwired: 2 in, 2 out]
        n644 = property on="R Scan Velocity SP deg/sec" class="DigNum (strict)"("Val(Sgnl)"=w1014) -> ()  [unwired: 2 in, 2 out]
      }
      event #4 {
        n645 = event-data() -> ()  [unwired: 1 in, 7 out]
        n646 = property on="Y Step SP" class="DigNum (strict)"() -> ("Maximum"=w1097:dbl)  [unwired: 2 in, 2 out]
        n647 = property on="Y Step SP" class="DigNum (strict)"() -> ("Minimum"=w1096:dbl)  [unwired: 2 in, 2 out]
        n648 = property on="Y steps/rev" class="DigNum (strict)"() -> ("Value"=w1103:u32)  [unwired: 2 in, 2 out]
        n649 = property on="Y offset mm" class="DigNum (strict)"() -> ("Value"=w1101:dbl)  [unwired: 2 in, 2 out]
        n650 = property on="Y Velocity SP step/sec" class="DigNum (strict)"() -> ("Maximum"=w1090:dbl)  [unwired: 2 in, 2 out]
        n651 = property on="Y Velocity SP step/sec" class="DigNum (strict)"() -> ("Minimum"=w1089:dbl)  [unwired: 2 in, 2 out]
        n652 = To Double Precision Float(number=w1103) -> (double precision float=w1088:dbl)
        n653 = property on="Y Position SP mm" class="DigNum (strict)"() -> ("Value"=w1100:dbl)  [unwired: 2 in, 2 out]
        n654 = property on="Y mm/rev" class="DigNum (strict)"() -> ("Value"=w1087:dbl)  [unwired: 2 in, 2 out]
        n655 = property on="Y Velocity SP mm/sec" class="DigNum (strict)"() -> ("Value"=w1094:dbl)  [unwired: 2 in, 2 out]
        n656 = Subtract(x=w1100, y=w1101) -> (x-y=w1104:dbl)
        n657 = Divide(x=w1094, y=w1087) -> (x/y=w1095:dbl)
        n658 = Divide(x=w1104, y=w1087) -> (x/y=w1105:dbl)
        n659 = Multiply(x=w1095, y=w1088) -> (x*y=w1092:dbl)
        n660 = Multiply(x=w1105, y=w1088) -> (x*y=w1099:dbl)
        n661 = In Range and Coerce(upper limit=w1090, x=w1092, lower limit=w1089) -> (coerced(x)=w1091:dbl)  [unwired: 1 out]
        n662 = To Long Integer(number=w1091) -> (32bit integer=w1093:i32)
        n663 = In Range and Coerce(upper limit=w1097, x=w1099, lower limit=w1096) -> (coerced(x)=w1098:dbl)  [unwired: 1 out]
        n664 = To Long Integer(number=w1098) -> (32bit integer=w1102:i32)
        n665 = property on="Y Velocity SP step/sec" class="DigNum (strict)"("Val(Sgnl)"=w1093) -> ()  [unwired: 2 in, 2 out]
        n666 = property on="Y Step SP" class="DigNum (strict)"("Val(Sgnl)"=w1102) -> ()  [unwired: 2 in, 2 out]
      }
      event #5 {
        n667 = event-data() -> ()  [unwired: 1 in, 7 out]
        n668 = property on="X Step SP" class="DigNum (strict)"() -> ("Maximum"=w1116:dbl)  [unwired: 2 in, 2 out]
        n669 = property on="X Step SP" class="DigNum (strict)"() -> ("Minimum"=w1115:dbl)  [unwired: 2 in, 2 out]
        n670 = property on="X steps/rev" class="DigNum (strict)"() -> ("Value"=w1122:u32)  [unwired: 2 in, 2 out]
        n671 = property on="X offset mm" class="DigNum (strict)"() -> ("Value"=w1120:dbl)  [unwired: 2 in, 2 out]
        n672 = property on="X Velocity SP step/sec" class="DigNum (strict)"() -> ("Maximum"=w1109:dbl)  [unwired: 2 in, 2 out]
        n673 = property on="X Velocity SP step/sec" class="DigNum (strict)"() -> ("Minimum"=w1108:dbl)  [unwired: 2 in, 2 out]
        n674 = property on="X Position SP mm" class="DigNum (strict)"() -> ("Value"=w1119:dbl)  [unwired: 2 in, 2 out]
        n675 = property on="X mm/rev" class="DigNum (strict)"() -> ("Value"=w1106:dbl)  [unwired: 2 in, 2 out]
        n676 = property on="X Velocity SP mm/sec" class="DigNum (strict)"() -> ("Value"=w1113:dbl)  [unwired: 2 in, 2 out]
        n677 = Subtract(x=w1119, y=w1120) -> (x-y=w1123:dbl)
        n678 = Divide(x=w1113, y=w1106) -> (x/y=w1114:dbl)
        n679 = To Double Precision Float(number=w1122) -> (double precision float=w1107:dbl)
        n680 = Divide(x=w1123, y=w1106) -> (x/y=w1124:dbl)
        n681 = Multiply(x=w1114, y=w1107) -> (x*y=w1111:dbl)
        n682 = Multiply(x=w1124, y=w1107) -> (x*y=w1118:dbl)
        n683 = In Range and Coerce(upper limit=w1109, x=w1111, lower limit=w1108) -> (coerced(x)=w1110:dbl)  [unwired: 1 out]
        n684 = To Long Integer(number=w1110) -> (32bit integer=w1112:i32)
        n685 = In Range and Coerce(upper limit=w1116, x=w1118, lower limit=w1115) -> (coerced(x)=w1117:dbl)  [unwired: 1 out]
        n686 = To Long Integer(number=w1117) -> (32bit integer=w1121:i32)
        n687 = property on="X Velocity SP step/sec" class="DigNum (strict)"("Val(Sgnl)"=w1112) -> ()  [unwired: 2 in, 2 out]
        n688 = property on="X Step SP" class="DigNum (strict)"("Val(Sgnl)"=w1121) -> ()  [unwired: 2 in, 2 out]
      }
      event #6 {
        n689 = event-data() -> ()  [unwired: 1 in, 7 out]
        n690 = property on="Z Step SP" class="DigNum (strict)"() -> ("Maximum"=w1133:dbl)  [unwired: 2 in, 2 out]
        n691 = property on="Z Step SP" class="DigNum (strict)"() -> ("Minimum"=w1132:dbl)  [unwired: 2 in, 2 out]
        n692 = property on="Z steps/rev" class="DigNum (strict)"() -> ("Value"=w1139:u32)  [unwired: 2 in, 2 out]
        n693 = property on="Z offset mm" class="DigNum (strict)"() -> ("Value"=w1137:dbl)  [unwired: 2 in, 2 out]
        n694 = property on="Z Velocity SP step/sec" class="DigNum (strict)"() -> ("Maximum"=w1126:dbl)  [unwired: 2 in, 2 out]
        n695 = property on="Z Velocity SP step/sec" class="DigNum (strict)"() -> ("Minimum"=w1125:dbl)  [unwired: 2 in, 2 out]
        n696 = property on="Z Position SP mm" class="DigNum (strict)"() -> ("Value"=w1136:dbl)  [unwired: 2 in, 2 out]
        n697 = property on="Z mm/rev" class="DigNum (strict)"() -> ("Value"=w1142:dbl)  [unwired: 2 in, 2 out]
        n698 = property on="Z Velocity SP mm/sec" class="DigNum (strict)"() -> ("Value"=w1130:dbl)  [unwired: 2 in, 2 out]
        n699 = Subtract(x=w1136, y=w1137) -> (x-y=w1140:dbl)
        n700 = Divide(x=w1130, y=w1142) -> (x/y=w1131:dbl)
        n701 = To Double Precision Float(number=w1139) -> (double precision float=w1143:dbl)
        n702 = Divide(x=w1140, y=w1142) -> (x/y=w1141:dbl)
        n703 = Multiply(x=w1131, y=w1143) -> (x*y=w1128:dbl)
        n704 = Multiply(x=w1141, y=w1143) -> (x*y=w1135:dbl)
        n705 = In Range and Coerce(upper limit=w1126, x=w1128, lower limit=w1125) -> (coerced(x)=w1127:dbl)  [unwired: 1 out]
        n706 = To Long Integer(number=w1127) -> (32bit integer=w1129:i32)
        n707 = In Range and Coerce(upper limit=w1133, x=w1135, lower limit=w1132) -> (coerced(x)=w1134:dbl)  [unwired: 1 out]
        n708 = To Long Integer(number=w1134) -> (32bit integer=w1138:i32)
        n709 = property on="Z Velocity SP step/sec" class="DigNum (strict)"("Val(Sgnl)"=w1129) -> ()  [unwired: 2 in, 2 out]
        n710 = property on="Z Step SP" class="DigNum (strict)"("Val(Sgnl)"=w1138) -> ()  [unwired: 2 in, 2 out]
      }
      event #7 {
        n711 = event-data() -> ()  [unwired: 1 in, 7 out]
        n712 = property on="R Step SP" class="DigNum (strict)"() -> ("Maximum"=w1155:dbl)  [unwired: 2 in, 2 out]
        n713 = property on="R Step SP" class="DigNum (strict)"() -> ("Minimum"=w1154:dbl)  [unwired: 2 in, 2 out]
        n714 = property on="R steps/rev" class="DigNum (strict)"() -> ("Value"=w1161:u32)  [unwired: 2 in, 2 out]
        n715 = property on="R offset deg" class="DigNum (strict)"() -> ("Value"=w1159:dbl)  [unwired: 2 in, 2 out]
        n716 = property on="R Velocity SP step/sec" class="DigNum (strict)"() -> ("Maximum"=w1148:dbl)  [unwired: 2 in, 2 out]
        n717 = property on="R Velocity SP step/sec" class="DigNum (strict)"() -> ("Minimum"=w1147:dbl)  [unwired: 2 in, 2 out]
        n718 = To Double Precision Float(number=w1161) -> (double precision float=w1146:dbl)
        n719 = property on="R Position SP deg" class="DigNum (strict)"() -> ("Value"=w1158:dbl)  [unwired: 2 in, 2 out]
        n720 = property on="R deg/rev" class="DigNum (strict)"() -> ("Value"=w1145:dbl)  [unwired: 2 in, 2 out]
        n721 = property on="R Velocity SP deg/sec" class="DigNum (strict)"() -> ("Value"=w1152:dbl)  [unwired: 2 in, 2 out]
        n722 = Subtract(x=w1158, y=w1159) -> (x-y=w1162:dbl)
        n723 = Divide(x=w1152, y=w1145) -> (x/y=w1153:dbl)
        n724 = Divide(x=w1162, y=w1145) -> (x/y=w1163:dbl)
        n725 = Multiply(x=w1153, y=w1146) -> (x*y=w1150:dbl)
        n726 = Multiply(x=w1163, y=w1146) -> (x*y=w1157:dbl)
        n727 = Absolute Value(x=w1150) -> (abs(x)=w1144:dbl)
        n728 = In Range and Coerce(upper limit=w1155, x=w1157, lower limit=w1154) -> (coerced(x)=w1156:dbl)  [unwired: 1 out]
        n729 = In Range and Coerce(upper limit=w1148, x=w1144, lower limit=w1147) -> (coerced(x)=w1149:dbl)  [unwired: 1 out]
        n730 = To Long Integer(number=w1156) -> (32bit integer=w1160:i32)
        n731 = To Long Integer(number=w1149) -> (32bit integer=w1151:i32)
        n732 = property on="R Step SP" class="DigNum (strict)"("Val(Sgnl)"=w1160) -> ()  [unwired: 2 in, 2 out]
        n733 = property on="R Velocity SP step/sec" class="DigNum (strict)"("Val(Sgnl)"=w1151) -> ()  [unwired: 2 in, 2 out]
      }
      event #8 {
        n734 = event-data() -> ()  [unwired: 1 in, 7 out]
        n735 = property on="Y Step SP" class="DigNum (strict)"() -> ("Maximum"=w1173:dbl)  [unwired: 2 in, 2 out]
        n736 = property on="Y Step SP" class="DigNum (strict)"() -> ("Minimum"=w1174:dbl)  [unwired: 2 in, 2 out]
        n737 = property on="Y steps/rev" class="DigNum (strict)"() -> ("Value"=w1179:u32)  [unwired: 2 in, 2 out]
        n738 = To Double Precision Float(number=w1179) -> (double precision float=w1165:dbl)
        n739 = property on="Y Scan Length SP mm" class="DigNum (strict)"() -> ("Value"=w1177:dbl)  [unwired: 2 in, 2 out]
        n740 = property on="Y mm/rev" class="DigNum (strict)"() -> ("Value"=w1164:dbl)  [unwired: 2 in, 2 out]
        n741 = property on="Y Scan Velocity SP steps/sec" class="DigNum (strict)"() -> ("Maximum"=w1167:dbl)  [unwired: 2 in, 2 out]
        n742 = property on="Y Scan Velocity SP steps/sec" class="DigNum (strict)"() -> ("Minimum"=w1166:dbl)  [unwired: 2 in, 2 out]
        n743 = property on="Y Scan Velocity SP mm/sec" class="DigNum (strict)"() -> ("Value"=w1171:dbl)  [unwired: 2 in, 2 out]
        n744 = Divide(x=w1177, y=w1164) -> (x/y=w1180:dbl)
        n745 = Multiply(x=w1180, y=w1165) -> (x*y=w1176:dbl)
        n746 = Divide(x=w1171, y=w1164) -> (x/y=w1172:dbl)
        n747 = Multiply(x=w1172, y=w1165) -> (x*y=w1169:dbl)
        n748 = In Range and Coerce(upper limit=w1173, x=w1176, lower limit=w1174) -> (coerced(x)=w1175:dbl)  [unwired: 1 out]
        n749 = To Long Integer(number=w1175) -> (32bit integer=w1178:i32)
        n750 = In Range and Coerce(upper limit=w1167, x=w1169, lower limit=w1166) -> (coerced(x)=w1168:dbl)  [unwired: 1 out]
        n751 = To Long Integer(number=w1168) -> (32bit integer=w1170:i32)
        n752 = property on="Y Scan Length SP steps" class="DigNum (strict)"("Val(Sgnl)"=w1178) -> ()  [unwired: 2 in, 2 out]
        n753 = property on="Y Scan Velocity SP steps/sec" class="DigNum (strict)"("Val(Sgnl)"=w1170) -> ()  [unwired: 2 in, 2 out]
      }
      event #9 {
        n754 = event-data() -> ()  [unwired: 1 in, 7 out]
        n755 = property on="X Step SP" class="DigNum (strict)"() -> ("Maximum"=w1190:dbl)  [unwired: 2 in, 2 out]
        n756 = property on="X Step SP" class="DigNum (strict)"() -> ("Minimum"=w1191:dbl)  [unwired: 2 in, 2 out]
        n757 = property on="X steps/rev" class="DigNum (strict)"() -> ("Value"=w1196:u32)  [unwired: 2 in, 2 out]
        n758 = To Double Precision Float(number=w1196) -> (double precision float=w1182:dbl)
        n759 = property on="X Scan Length SP mm" class="DigNum (strict)"() -> ("Value"=w1194:dbl)  [unwired: 2 in, 2 out]
        n760 = property on="X mm/rev" class="DigNum (strict)"() -> ("Value"=w1181:dbl)  [unwired: 2 in, 2 out]
        n761 = property on="X Scan Velocity SP steps/sec" class="DigNum (strict)"() -> ("Maximum"=w1184:dbl)  [unwired: 2 in, 2 out]
        n762 = property on="X Scan Velocity SP steps/sec" class="DigNum (strict)"() -> ("Minimum"=w1183:dbl)  [unwired: 2 in, 2 out]
        n763 = property on="X Scan Velocity SP mm/sec" class="DigNum (strict)"() -> ("Value"=w1188:dbl)  [unwired: 2 in, 2 out]
        n764 = Divide(x=w1194, y=w1181) -> (x/y=w1197:dbl)
        n765 = Multiply(x=w1197, y=w1182) -> (x*y=w1193:dbl)
        n766 = Divide(x=w1188, y=w1181) -> (x/y=w1189:dbl)
        n767 = Multiply(x=w1189, y=w1182) -> (x*y=w1186:dbl)
        n768 = In Range and Coerce(upper limit=w1190, x=w1193, lower limit=w1191) -> (coerced(x)=w1192:dbl)  [unwired: 1 out]
        n769 = To Long Integer(number=w1192) -> (32bit integer=w1195:i32)
        n770 = In Range and Coerce(upper limit=w1184, x=w1186, lower limit=w1183) -> (coerced(x)=w1185:dbl)  [unwired: 1 out]
        n771 = To Long Integer(number=w1185) -> (32bit integer=w1187:i32)
        n772 = property on="X Scan Length SP steps" class="DigNum (strict)"("Val(Sgnl)"=w1195) -> ()  [unwired: 2 in, 2 out]
        n773 = property on="X Scan Velocity SP steps/sec" class="DigNum (strict)"("Val(Sgnl)"=w1187) -> ()  [unwired: 2 in, 2 out]
      }
      event #10 {
        n774 = event-data() -> ()  [unwired: 1 in, 7 out]
        n775 = property on="Z Step SP" class="DigNum (strict)"() -> ("Maximum"=w1207:dbl)  [unwired: 2 in, 2 out]
        n776 = property on="Z Step SP" class="DigNum (strict)"() -> ("Minimum"=w1208:dbl)  [unwired: 2 in, 2 out]
        n777 = property on="Z steps/rev" class="DigNum (strict)"() -> ("Value"=w1213:u32)  [unwired: 2 in, 2 out]
        n778 = To Double Precision Float(number=w1213) -> (double precision float=w1199:dbl)
        n779 = property on="Z Scan Length SP mm" class="DigNum (strict)"() -> ("Value"=w1211:dbl)  [unwired: 2 in, 2 out]
        n780 = property on="Z mm/rev" class="DigNum (strict)"() -> ("Value"=w1198:dbl)  [unwired: 2 in, 2 out]
        n781 = property on="Z Scan Velocity SP steps/sec" class="DigNum (strict)"() -> ("Maximum"=w1201:dbl)  [unwired: 2 in, 2 out]
        n782 = property on="Z Scan Velocity SP steps/sec" class="DigNum (strict)"() -> ("Minimum"=w1200:dbl)  [unwired: 2 in, 2 out]
        n783 = property on="Z Scan Velocity SP mm/sec" class="DigNum (strict)"() -> ("Value"=w1205:dbl)  [unwired: 2 in, 2 out]
        n784 = Divide(x=w1211, y=w1198) -> (x/y=w1214:dbl)
        n785 = Multiply(x=w1214, y=w1199) -> (x*y=w1210:dbl)
        n786 = Divide(x=w1205, y=w1198) -> (x/y=w1206:dbl)
        n787 = Multiply(x=w1206, y=w1199) -> (x*y=w1203:dbl)
        n788 = In Range and Coerce(upper limit=w1207, x=w1210, lower limit=w1208) -> (coerced(x)=w1209:dbl)  [unwired: 1 out]
        n789 = To Long Integer(number=w1209) -> (32bit integer=w1212:i32)
        n790 = In Range and Coerce(upper limit=w1201, x=w1203, lower limit=w1200) -> (coerced(x)=w1202:dbl)  [unwired: 1 out]
        n791 = To Long Integer(number=w1202) -> (32bit integer=w1204:i32)
        n792 = property on="Z Scan Length SP steps" class="DigNum (strict)"("Val(Sgnl)"=w1212) -> ()  [unwired: 2 in, 2 out]
        n793 = property on="Z Scan Velocity SP steps/sec" class="DigNum (strict)"("Val(Sgnl)"=w1204) -> ()  [unwired: 2 in, 2 out]
      }
      event #11 {
        n794 = event-data() -> ()  [unwired: 1 in, 7 out]
        n795 = property on="R Step SP" class="DigNum (strict)"() -> ("Maximum"=w1225:dbl)  [unwired: 2 in, 2 out]
        n796 = property on="R Step SP" class="DigNum (strict)"() -> ("Minimum"=w1226:dbl)  [unwired: 2 in, 2 out]
        n797 = property on="R steps/rev" class="DigNum (strict)"() -> ("Value"=w1231:u32)  [unwired: 2 in, 2 out]
        n798 = property on="R Velocity SP step/sec" class="DigNum (strict)"() -> ("Maximum"=w1219:dbl)  [unwired: 2 in, 2 out]
        n799 = To Double Precision Float(number=w1231) -> (double precision float=w1217:dbl)
        n800 = property on="R Scan Length SP deg" class="DigNum (strict)"() -> ("Value"=w1229:dbl)  [unwired: 2 in, 2 out]
        n801 = property on="R deg/rev" class="DigNum (strict)"() -> ("Value"=w1216:dbl)  [unwired: 2 in, 2 out]
        n802 = property on="R Scan Velocity SP steps/sec" class="DigNum (strict)"() -> ("Minimum"=w1218:dbl)  [unwired: 2 in, 2 out]
        n803 = property on="R Scan Velocity SP deg/sec" class="DigNum (strict)"() -> ("Value"=w1223:dbl)  [unwired: 2 in, 2 out]
        n804 = Divide(x=w1229, y=w1216) -> (x/y=w1232:dbl)
        n805 = Multiply(x=w1232, y=w1217) -> (x*y=w1228:dbl)
        n806 = Divide(x=w1223, y=w1216) -> (x/y=w1224:dbl)
        n807 = Multiply(x=w1224, y=w1217) -> (x*y=w1221:dbl)
        n808 = In Range and Coerce(upper limit=w1225, x=w1228, lower limit=w1226) -> (coerced(x)=w1227:dbl)  [unwired: 1 out]
        n809 = To Long Integer(number=w1227) -> (32bit integer=w1230:i32)
        n810 = Absolute Value(x=w1221) -> (abs(x)=w1215:dbl)
        n811 = property on="R Scan Length SP steps" class="DigNum (strict)"("Val(Sgnl)"=w1230) -> ()  [unwired: 2 in, 2 out]
        n812 = In Range and Coerce(upper limit=w1219, x=w1215, lower limit=w1218) -> (coerced(x)=w1220:dbl)  [unwired: 1 out]
        n813 = To Long Integer(number=w1220) -> (32bit integer=w1222:i32)
        n814 = property on="R Scan Velocity SP steps/sec" class="DigNum (strict)"("Val(Sgnl)"=w1222) -> ()  [unwired: 2 in, 2 out]
      }
      event #12 {
        n815 = event-data() -> ()  [unwired: 1 in, 7 out]
        n816 = flat-sequence {
          tunnel: w1239 -> [w1249]
          tunnel: w1240 -> [w1250]
          tunnel: [w1250] -> w1236
          tunnel: [w1249] -> w1235
          tunnel: [w1253] -> w1238
          tunnel: [w1252] -> w1237
          tunnel: w1236 -> [w1255]
          tunnel: w1235 -> [w1254]
          tunnel: [w1276] -> w1242
          tunnel: [w1271] -> w1241
          tunnel: w1238 -> [w1275]
          tunnel: w1237 -> [w1274]
          tunnel: [w1270] -> w1234
          tunnel: [w1287] -> w1244
          tunnel: [w1282] -> w1243
          tunnel: w1242 -> [w1285]
          tunnel: w1241 -> [w1286]
          tunnel: w1234 -> [w1283]
          tunnel: [w1283] -> w1233
          tunnel: [w1290] -> w1245
          tunnel: [w1293] -> w1246
          tunnel: w1244 -> [w1292]
          tunnel: w1243 -> [w1291]
          tunnel: w1233 -> [w1294]
          frame #0 {
            n817 = property on="Y Go" class="Bool"("DisabledEnum"=T2."Disabled and Grayed Out" ("Disabled")) -> ()  [unwired: 2 in, 2 out]
            n818 = property on="Scan Go" class="Bool"("DisabledEnum"=T2."Disabled and Grayed Out" ("Disabled")) -> ()  [unwired: 2 in, 2 out]
          }
          frame #1 {
            n819 = property on="Y Step SP" class="DigNum (strict)"() -> ("Value"=w1263:i32)  [unwired: 2 in, 2 out]
            n820 = property on="Y Step PV" class="DigNum (strict)"() -> ("Value"=w1262:i32)  [unwired: 2 in, 2 out]
            n821 = property on="Y Backlash" class="DigNum (strict)"() -> ("Value"=w1251:i32)  [unwired: 2 in, 2 out]
            n822 = Subtract(x=w1263, y=w1262) -> (x-y=w1261:i32)
            n823 = Sign(1:w1251) -> (0:w1259:i32)
            n824 = Sign(1:w1261) -> (0:w1260:i32)
            n825 = Multiply(x=w1260, y=w1259) -> (x*y=w1258:i32)
            n826 = Equal?(x=w1258, y=1) -> (x = y?=w1256:bool)
            n827 = case shown="False" w1256 {
              tunnel: w1255 -> [w1266 w1268]
              tunnel: w1254 -> [w1265 w1267]
              tunnel: [w1265 w1267] -> w1253
              tunnel: [w1266 w1268] -> w1252
              frame #0 {
                n828 = property on="Y Backlash corr" class="Bool (strict)"("Val(Sgnl)"=FALSE ("Value (Signaling)")) -> ()  [unwired: 2 in, 2 out]
              }
              frame #1 {
                n829 = property on="Y Backlash corr" class="Bool (strict)"("Val(Sgnl)"=TRUE ("Value (Signaling)")) -> ()  [unwired: 2 in, 2 out]
              }
            }
          }
          frame #2 {
            w1270 = 0.1 ("Delay Time (s)")
            # "Velocity Setting"
            n830 = property on="Y steps/rev" class="DigNum (strict)"() -> ("Value"=w1278:u32)  [unwired: 2 in, 2 out]
            n831 = property on="Y Velocity SP step/sec" class="DigNum (strict)"() -> ("Value"=w1279:i32)  [unwired: 2 in, 2 out]
            n832 = Number To Decimal String(number=w1279) -> ()  [unwired: 1 in, 1 out]
            n833 = Divide(x=w1279, y=w1278) -> (x/y=w1280:dbl)
            n834 = Number To Fractional String(number=w1280) -> (F-format string=w1273:string)  [unwired: 3 in]
            n835 = call "Applied Send Command.vi"("error in (no error)"=w1275, "Extra"=w1273, "Command"=T1."Velocity Setting", "VISA resource name"=w1274) -> ("error out"=w1272:errorcluster, "VISA resource name out"=w1276:refnum<visa-resource-name>)  [unwired: 3 in, 1 out]
            n836 = call "Time Delay22"("error in (no error)"=w1272, "Delay Time (s)"=w1270) -> ("error out"=w1271:errorcluster)  [unwired: 9 in]
          }
          frame #3 {
            # "Move to Abs Position"
            n837 = property on="Y Step SP" class="DigNum (strict)"() -> ("Value"=w1289:i32)  [unwired: 2 in, 2 out]
            n838 = Number To Decimal String(number=w1289) -> (decimal integer string=w1284:string)  [unwired: 1 in]
            n839 = call "Applied Send Command.vi"("error in (no error)"=w1286, "Extra"=w1284, "Command"=T1."Distance or Position", "VISA resource name"=w1285) -> ("error out"=w1281:errorcluster, "VISA resource name out"=w1287:refnum<visa-resource-name>)  [unwired: 3 in, 1 out]
            n840 = call "Time Delay"("error in (no error)"=w1281, "Delay Time (s)"=w1283) -> ("error out"=w1282:errorcluster)  [unwired: 9 in]
          }
          frame #4 {
            n841 = call "Applied Send Command.vi"("error in (no error)"=w1291, "Command"=T1."Feed to Position", "VISA resource name"=w1292) -> ("error out"=w1295:errorcluster, "VISA resource name out"=w1293:refnum<visa-resource-name>)  [unwired: 4 in, 1 out]
            n842 = call "Time Delay23"("error in (no error)"=w1295, "Delay Time (s)"=w1294) -> ("error out"=w1290:errorcluster)  [unwired: 9 in]
          }
        }
      }
      event #13 {
        n843 = event-data() -> ()  [unwired: 1 in, 7 out]
        n844 = flat-sequence {
          tunnel: w1301 -> [w1313]
          tunnel: w1302 -> [w1314]
          tunnel: [w1314] -> w1304
          tunnel: [w1313] -> w1303
          tunnel: [w1317] -> w1306
          tunnel: [w1316] -> w1305
          tunnel: w1304 -> [w1319]
          tunnel: w1303 -> [w1318]
          tunnel: [w1337] -> w1308
          tunnel: [w1335] -> w1307
          tunnel: w1306 -> [w1338]
          tunnel: w1305 -> [w1339]
          tunnel: [w1334] -> w1298
          tunnel: [w1348] -> w1310
          tunnel: [w1347] -> w1309
          tunnel: w1308 -> [w1349]
          tunnel: w1307 -> [w1351]
          tunnel: w1298 -> [w1345]
          tunnel: [w1345] -> w1297
          tunnel: [w1360] -> w1300
          tunnel: [w1356] -> w1299
          tunnel: w1310 -> [w1357]
          tunnel: w1309 -> [w1354]
          tunnel: w1297 -> [w1359]
          frame #0 {
            n845 = property on="Z Go" class="Bool"("DisabledEnum"=T2."Disabled and Grayed Out" ("Disabled")) -> ()  [unwired: 2 in, 2 out]
            n846 = property on="Scan Go" class="Bool"("DisabledEnum"=T2."Disabled and Grayed Out" ("Disabled")) -> ()  [unwired: 2 in, 2 out]
          }
          frame #1 {
            n847 = property on="Z Step SP" class="DigNum (strict)"() -> ("Value"=w1327:i32)  [unwired: 2 in, 2 out]
            n848 = property on="Z Step PV" class="DigNum (strict)"() -> ("Value"=w1326:i32)  [unwired: 2 in, 2 out]
            n849 = property on="Z Backlash" class="DigNum (strict)"() -> ("Value"=w1315:i32)  [unwired: 2 in, 2 out]
            n850 = Subtract(x=w1327, y=w1326) -> (x-y=w1325:i32)
            n851 = Sign(1:w1315) -> (0:w1323:i32)
            n852 = Sign(1:w1325) -> (0:w1324:i32)
            n853 = Multiply(x=w1324, y=w1323) -> (x*y=w1322:i32)
            n854 = Equal?(x=w1322, y=1) -> (x = y?=w1320:bool)
            n855 = case shown="True" w1320 {
              tunnel: w1319 -> [w1330 w1332]
              tunnel: w1318 -> [w1329 w1331]
              tunnel: [w1329 w1331] -> w1317
              tunnel: [w1330 w1332] -> w1316
              frame #0 {
                n856 = property on="Z Backlash corr" class="Bool (strict)"("Val(Sgnl)"=FALSE ("Value (Signaling)")) -> ()  [unwired: 2 in, 2 out]
              }
              frame #1 {
                n857 = property on="Z Backlash corr" class="Bool (strict)"("Val(Sgnl)"=TRUE ("Value (Signaling)")) -> ()  [unwired: 2 in, 2 out]
              }
            }
          }
          frame #2 {
            w1334 = 0.1 ("Delay Time (s)")
            n858 = property on="Z steps/rev" class="DigNum (strict)"() -> ("Value"=w1340:u32)  [unwired: 2 in, 2 out]
            n859 = property on="Z Velocity SP step/sec" class="DigNum (strict)"() -> ("Value"=w1341:i32)  [unwired: 2 in, 2 out]
            n860 = Divide(x=w1341, y=w1340) -> (x/y=w1342:dbl)
            n861 = Number To Fractional String(number=w1342) -> (F-format string=w1343:string)  [unwired: 3 in]
            n862 = call "Applied Send Command.vi"("error in (no error)"=w1338, "Extra"=w1343, "Command"=T1."Velocity Setting", "VISA resource name"=w1339) -> ("error out"=w1336:errorcluster, "VISA resource name out"=w1337:refnum<visa-resource-name>)  [unwired: 3 in, 1 out]
            n863 = call "Time Delay52"("error in (no error)"=w1336, "Delay Time (s)"=w1334) -> ("error out"=w1335:errorcluster)  [unwired: 9 in]
          }
          frame #3 {
            # "Move to Abs Position"
            n864 = property on="Z Step SP" class="DigNum (strict)"() -> ("Value"=w1353:i32)  [unwired: 2 in, 2 out]
            n865 = Number To Decimal String(number=w1353) -> (decimal integer string=w1350:string)  [unwired: 1 in]
            n866 = call "Applied Send Command.vi"("error in (no error)"=w1351, "Extra"=w1350, "Command"=T1."Distance or Position", "VISA resource name"=w1349) -> ("error out"=w1346:errorcluster, "VISA resource name out"=w1348:refnum<visa-resource-name>)  [unwired: 3 in, 1 out]
            n867 = call "Time Delay51"("error in (no error)"=w1346, "Delay Time (s)"=w1345) -> ("error out"=w1347:errorcluster)  [unwired: 9 in]
          }
          frame #4 {
            n868 = call "Applied Send Command.vi"("error in (no error)"=w1354, "Command"=T1."Feed to Position", "VISA resource name"=w1357) -> ("error out"=w1355:errorcluster, "VISA resource name out"=w1356:refnum<visa-resource-name>)  [unwired: 4 in, 1 out]
            n869 = call "Time Delay28"("error in (no error)"=w1355, "Delay Time (s)"=w1359) -> ("error out"=w1360:errorcluster)  [unwired: 9 in]
          }
        }
      }
      event #14 {
        n870 = event-data() -> ()  [unwired: 1 in, 7 out]
        n871 = flat-sequence {
          tunnel: w1365 -> [w1377]
          tunnel: w1366 -> [w1378]
          tunnel: [w1378] -> w1368
          tunnel: [w1377] -> w1367
          tunnel: [w1381] -> w1370
          tunnel: [w1380] -> w1369
          tunnel: w1368 -> [w1383]
          tunnel: w1367 -> [w1382]
          tunnel: [w1399] -> w1372
          tunnel: [w1400] -> w1371
          tunnel: w1370 -> [w1401]
          tunnel: w1369 -> [w1402]
          tunnel: [w1398] -> w1362
          tunnel: [w1412] -> w1374
          tunnel: [w1410] -> w1373
          tunnel: w1372 -> [w1411]
          tunnel: w1371 -> [w1413]
          tunnel: w1362 -> [w1408]
          tunnel: [w1408] -> w1361
          tunnel: [w1423] -> w1364
          tunnel: [w1419] -> w1363
          tunnel: w1374 -> [w1420]
          tunnel: w1373 -> [w1417]
          tunnel: w1361 -> [w1422]
          frame #0 {
            n872 = property on="R Go" class="Bool"("DisabledEnum"=T2."Disabled and Grayed Out" ("Disabled")) -> ()  [unwired: 2 in, 2 out]
            n873 = property on="Scan Go" class="Bool"("DisabledEnum"=T2."Disabled and Grayed Out" ("Disabled")) -> ()  [unwired: 2 in, 2 out]
          }
          frame #1 {
            n874 = property on="R Step SP" class="DigNum (strict)"() -> ("Value"=w1391:i32)  [unwired: 2 in, 2 out]
            n875 = property on="R Step PV" class="DigNum (strict)"() -> ("Value"=w1390:i32)  [unwired: 2 in, 2 out]
            n876 = property on="R Backlash" class="DigNum (strict)"() -> ("Value"=w1379:i32)  [unwired: 2 in, 2 out]
            n877 = Subtract(x=w1391, y=w1390) -> (x-y=w1389:i32)
            n878 = Sign(1:w1379) -> (0:w1387:i32)
            n879 = Sign(1:w1389) -> (0:w1388:i32)
            n880 = Multiply(x=w1388, y=w1387) -> (x*y=w1386:i32)
            n881 = Equal?(x=w1386, y=1) -> (x = y?=w1384:bool)
            n882 = case shown="True" w1384 {
              tunnel: w1383 -> [w1394 w1396]
              tunnel: w1382 -> [w1393 w1395]
              tunnel: [w1393 w1395] -> w1381
              tunnel: [w1394 w1396] -> w1380
              frame #0 {
                n883 = property on="R Backlash corr" class="Bool (strict)"("Val(Sgnl)"=FALSE ("Value (Signaling)")) -> ()  [unwired: 2 in, 2 out]
              }
              frame #1 {
                n884 = property on="R Backlash corr" class="Bool (strict)"("Val(Sgnl)"=TRUE ("Value (Signaling)")) -> ()  [unwired: 2 in, 2 out]
              }
            }
          }
          frame #2 {
            w1398 = 0.1 ("Delay Time (s)")
            # "Velocity Setting"
            n885 = property on="R steps/rev" class="DigNum (strict)"() -> ("Value"=w1403:u32)  [unwired: 2 in, 2 out]
            n886 = property on="R Velocity SP step/sec" class="DigNum (strict)"() -> ("Value"=w1404:i32)  [unwired: 2 in, 2 out]
            n887 = Divide(x=w1404, y=w1403) -> (x/y=w1405:dbl)
            n888 = Number To Fractional String(number=w1405) -> (F-format string=w1406:string)  [unwired: 3 in]
            n889 = call "Applied Send Command.vi"("error in (no error)"=w1401, "Extra"=w1406, "VISA resource name"=w1402) -> ("error out"=w1407:errorcluster, "VISA resource name out"=w1399:refnum<visa-resource-name>)  [unwired: 4 in, 1 out]
            n890 = call "Time Delay54"("error in (no error)"=w1407, "Delay Time (s)"=w1398) -> ("error out"=w1400:errorcluster)  [unwired: 9 in]
          }
          frame #3 {
            # "Distance/Position"
            n891 = property on="R Step SP" class="DigNum (strict)"() -> ("Value"=w1414:i32)  [unwired: 2 in, 2 out]
            n892 = Number To Decimal String(number=w1414) -> (decimal integer string=w1415:string)  [unwired: 1 in]
            n893 = call "Applied Send Command.vi"("error in (no error)"=w1413, "Extra"=w1415, "Command"=T1."Distance or Position", "VISA resource name"=w1411) -> ("error out"=w1409:errorcluster, "VISA resource name out"=w1412:refnum<visa-resource-name>)  [unwired: 3 in, 1 out]
            n894 = call "Time Delay53"("error in (no error)"=w1409, "Delay Time (s)"=w1408) -> ("error out"=w1410:errorcluster)  [unwired: 9 in]
          }
          frame #4 {
            # "Feed to Position"
            n895 = call "Applied Send Command.vi"("error in (no error)"=w1417, "Command"=T1."Feed to Position", "VISA resource name"=w1420) -> ("error out"=w1418:errorcluster, "VISA resource name out"=w1419:refnum<visa-resource-name>)  [unwired: 4 in, 1 out]
            n896 = call "Time Delay29"("error in (no error)"=w1418, "Delay Time (s)"=w1422) -> ("error out"=w1423:errorcluster)  [unwired: 9 in]
          }
        }
      }
      event #15 {
        n897 = event-data() -> ()  [unwired: 1 in, 7 out]
        n898 = flat-sequence {
          tunnel: [w1439] -> w1435
          tunnel: [w1438] -> w1434
          tunnel: w1433 -> [w1439]
          tunnel: w1432 -> [w1438]
          tunnel: [w1444] -> w1437
          tunnel: [w1443] -> w1436
          tunnel: w1435 -> [w1446]
          tunnel: w1434 -> [w1445]
          tunnel: [w1465] -> w1429
          tunnel: [w1462] -> w1427
          tunnel: w1437 -> [w1466]
          tunnel: w1436 -> [w1467]
          tunnel: [w1461] -> w1425
          tunnel: w1429 -> [w1474]
          tunnel: [w1473] -> w1428
          tunnel: w1427 -> [w1475]
          tunnel: [w1476] -> w1426
          tunnel: w1425 -> [w1472]
          tunnel: [w1472] -> w1424
          tunnel: w1428 -> [w1486]
          tunnel: w1426 -> [w1485]
          tunnel: [w1484] -> w1431
          tunnel: [w1483] -> w1430
          tunnel: w1424 -> [w1481]
          frame #0 {
            n899 = property on="X Go" class="Bool"("DisabledEnum"=T2."Disabled and Grayed Out" ("Disabled")) -> ()  [unwired: 2 in, 2 out]
            n900 = property on="Scan Go" class="Bool"("DisabledEnum"=T2."Disabled and Grayed Out" ("Disabled")) -> ()  [unwired: 2 in, 2 out]
          }
          frame #1 {
            n901 = property on="X Step SP" class="DigNum (strict)"() -> ("Value"=w1454:i32)  [unwired: 2 in, 2 out]
            n902 = property on="X Step PV" class="DigNum (strict)"() -> ("Value"=w1453:i32)  [unwired: 2 in, 2 out]
            n903 = property on="X Backlash" class="DigNum (strict)"() -> ("Value"=w1442:i32)  [unwired: 2 in, 2 out]
            n904 = Subtract(x=w1454, y=w1453) -> (x-y=w1452:i32)
            n905 = Sign(1:w1442) -> (0:w1450:i32)
            n906 = Sign(1:w1452) -> (0:w1451:i32)
            n907 = Multiply(x=w1451, y=w1450) -> (x*y=w1449:i32)
            n908 = Equal?(x=w1449, y=1) -> (x = y?=w1447:bool)
            n909 = case shown="True" w1447 {
              tunnel: w1446 -> [w1457 w1459]
              tunnel: w1445 -> [w1456 w1458]
              tunnel: [w1456 w1458] -> w1444
              tunnel: [w1457 w1459] -> w1443
              frame #0 {
                n910 = property on="X Backlash corr" class="Bool (strict)"("Val(Sgnl)"=FALSE ("Value (Signaling)")) -> ()  [unwired: 2 in, 2 out]
              }
              frame #1 {
                n911 = property on="X Backlash corr" class="Bool (strict)"("Val(Sgnl)"=TRUE ("Value (Signaling)")) -> ()  [unwired: 2 in, 2 out]
              }
            }
          }
          frame #2 {
            w1461 = 0.1 ("Delay Time (s)")
            n912 = property on="X steps/rev" class="DigNum (strict)"() -> ("Value"=w1468:u32)  [unwired: 2 in, 2 out]
            n913 = property on="X Velocity SP step/sec" class="DigNum (strict)"() -> ("Value"=w1464:i32)  [unwired: 2 in, 2 out]
            n914 = Divide(x=w1464, y=w1468) -> (x/y=w1469:dbl)
            n915 = Number To Fractional String(number=w1469) -> (F-format string=w1470:string)  [unwired: 3 in]
            n916 = call "Applied Send Command.vi"("error in (no error)"=w1466, "Extra"=w1470, "Command"=T1."Velocity Setting", "VISA resource name"=w1467) -> ("error out"=w1463:errorcluster, "VISA resource name out"=w1465:refnum<visa-resource-name>)  [unwired: 3 in, 1 out]
            n917 = call "Time Delay14"("error in (no error)"=w1463, "Delay Time (s)"=w1461) -> ("error out"=w1462:errorcluster)  [unwired: 9 in]
          }
          frame #3 {
            # "Distance/Position"
            n918 = property on="X Step SP" class="DigNum (strict)"() -> ("Value"=w1477:i32)  [unwired: 2 in, 2 out]
            n919 = Number To Decimal String(number=w1477) -> (decimal integer string=w1479:string)  [unwired: 1 in]
            n920 = call "Applied Send Command.vi"("error in (no error)"=w1475, "Extra"=w1479, "Command"=T1."Distance or Position", "VISA resource name"=w1474) -> ("error out"=w1478:errorcluster, "VISA resource name out"=w1473:refnum<visa-resource-name>)  [unwired: 3 in, 1 out]
            n921 = call "Time Delay31"("error in (no error)"=w1478, "Delay Time (s)"=w1472) -> ("error out"=w1476:errorcluster)  [unwired: 9 in]
          }
          frame #4 {
            # "Feed to Position"
            n922 = call "Applied Send Command.vi"("error in (no error)"=w1485, "Command"=T1."Feed to Position", "VISA resource name"=w1486) -> ("error out"=w1482:errorcluster, "VISA resource name out"=w1484:refnum<visa-resource-name>)  [unwired: 4 in, 1 out]
            n923 = call "Time Delay15"("error in (no error)"=w1482, "Delay Time (s)"=w1481) -> ("error out"=w1483:errorcluster)  [unwired: 9 in]
          }
        }
      }
      event #16 {
        n924 = event-data() -> ()  [unwired: 1 in, 7 out]
        n925 = flat-sequence {
          tunnel: [w1503] -> w1495
          tunnel: [w1514] -> w1494
          tunnel: w1493 -> [w1511]
          tunnel: w1492 -> [w1510]
          tunnel: w1495 -> [w1521]
          tunnel: w1494 -> [w1520]
          tunnel: [w1521] -> w1489
          tunnel: [w1520] -> w1488
          tunnel: [w1523] -> w1490
          tunnel: [w1524] -> w1491
          tunnel: w1489 -> [w1524]
          tunnel: w1488 -> [w1523]
          frame #0 {
            # "VELOCITY"
            n926 = property on="X steps/rev" class="DigNum (strict)"() -> ("Value"=w1496:u32)  [unwired: 2 in, 2 out]
            n927 = property on="X Scan Velocity SP steps/sec" class="DigNum (strict)"() -> ("Value"=w1497:i32)  [unwired: 2 in, 2 out]
            n928 = Divide(x=w1497, y=w1496) -> (x/y=w1498:dbl)
            n929 = Number To Fractional String(number=w1498) -> (F-format string=w1512:string)  [unwired: 3 in]
            n930 = call "Applied Send Command.vi"("error in (no error)"=w1510, "Extra"=w1512, "Command"=T1."Velocity Setting", "VISA resource name"=w1511) -> ("error out"=w1499:errorcluster, "VISA resource name out"=w1500:refnum<visa-resource-name>)  [unwired: 3 in, 1 out]
            n931 = call "Time Delay9"("error in (no error)"=w1499) -> ("error out"=w1501:errorcluster)  [unwired: 10 in]
            n932 = call "Applied Send Command.vi"("error in (no error)"=w1501, "Extra"="", "Command"=T1."Velocity Setting", "VISA resource name"=w1500) -> ("error out"=w1502:errorcluster, "read buffer"=w1507:string, "VISA resource name out"=w1503:refnum<visa-resource-name>)  [unwired: 3 in]
            n933 = call "Time Delay10"("error in (no error)"=w1502) -> ("error out"=w1514:errorcluster)  [unwired: 10 in]
            n934 = Fract/Exp String To Number(string=w1507, offset=3) -> (number=w1505:dbl)  [unwired: 2 in, 1 out]
            n935 = Multiply(x=w1505, y=w1496) -> (x*y=w1504:dbl)
            n936 = property on="X velocity PV step/sec" class="DigNum (strict)"("Val(Sgnl)"=w1504) -> ()  [unwired: 2 in, 2 out]
          }
          frame #1 {
            n937 = property on="X Scan" class="Bool (strict)"("Val(Sgnl)"=TRUE ("Slew Ready 2")) -> ()  [unwired: 2 in, 2 out]
            n938 = property on="Scan Cancel" class="Bool"("DisabledEnum"=T2."Enabled" ("Disabled")) -> ()  [unwired: 2 in, 2 out]
            n939 = property on="Scan Go" class="Bool"("DisabledEnum"=T2."Enabled" ("Disabled")) -> ()  [unwired: 2 in, 2 out]
            n940 = property on="X Scan Length SP steps" class="DigNum (strict)"("DisabledEnum"=T2."Disabled and Grayed Out" ("Disabled")) -> ()  [unwired: 2 in, 2 out]
            n941 = property on="X Scan Velocity SP steps/sec" class="DigNum (strict)"("DisabledEnum"=T2."Disabled and Grayed Out" ("Disabled")) -> ()  [unwired: 2 in, 2 out]
          }
          frame #2 {
            n942 = property on="X Go" class="Bool"("DisabledEnum"=T2."Disabled and Grayed Out" ("Disabled")) -> ()  [unwired: 2 in, 2 out]
          }
        }
      }
      event #17 {
        n943 = event-data() -> ()  [unwired: 1 in, 7 out]
        n944 = flat-sequence {
          tunnel: w1532 -> [w1544]
          tunnel: w1531 -> [w1545]
          tunnel: [w1535] -> w1529
          tunnel: [w1551] -> w1528
          tunnel: w1529 -> [w1558]
          tunnel: w1528 -> [w1557]
          tunnel: [w1558] -> w1526
          tunnel: [w1557] -> w1525
          tunnel: [w1560] -> w1530
          tunnel: [w1561] -> w1527
          tunnel: w1526 -> [w1561]
          tunnel: w1525 -> [w1560]
          frame #0 {
            # "VELOCITY"
            n945 = property on="Y steps/rev" class="DigNum (strict)"() -> ("Value"=w1538:u32)  [unwired: 2 in, 2 out]
            n946 = property on="Y Scan Velocity SP steps/sec" class="DigNum (strict)"() -> ("Value"=w1547:i32)  [unwired: 2 in, 2 out]
            n947 = Divide(x=w1547, y=w1538) -> (x/y=w1548:dbl)
            n948 = Number To Fractional String(number=w1548) -> (F-format string=w1549:string)  [unwired: 3 in]
            n949 = call "Applied Send Command.vi"("error in (no error)"=w1544, "Extra"=w1549, "Command"=T1."Velocity Setting", "VISA resource name"=w1545) -> ("error out"=w1546:errorcluster, "VISA resource name out"=w1536:refnum<visa-resource-name>)  [unwired: 3 in, 1 out]
            n950 = call "Time Delay5"("error in (no error)"=w1546) -> ("error out"=w1537:errorcluster)  [unwired: 10 in]
            n951 = call "Applied Send Command.vi"("error in (no error)"=w1537, "Extra"="", "Command"=T1."Velocity Setting", "VISA resource name"=w1536) -> ("error out"=w1534:errorcluster, "read buffer"=w1541:string, "VISA resource name out"=w1535:refnum<visa-resource-name>)  [unwired: 3 in]
            n952 = Fract/Exp String To Number(string=w1541, offset=3) -> (number=w1540:dbl)  [unwired: 2 in, 1 out]
            n953 = call "Time Delay6"("error in (no error)"=w1534) -> ("error out"=w1551:errorcluster)  [unwired: 10 in]
            n954 = Multiply(x=w1540, y=w1538) -> (x*y=w1539:dbl)
            n955 = property on="Y velocity PV step/sec" class="DigNum (strict)"("Val(Sgnl)"=w1539) -> ()  [unwired: 2 in, 2 out]
          }
          frame #1 {
            n956 = property on="Y Scan" class="Bool (strict)"("Val(Sgnl)"=TRUE ("Slew Ready 2")) -> ()  [unwired: 2 in, 2 out]
            n957 = property on="Scan Cancel" class="Bool"("DisabledEnum"=T2."Enabled" ("Disabled")) -> ()  [unwired: 2 in, 2 out]
            n958 = property on="Scan Go" class="Bool"("DisabledEnum"=T2."Enabled" ("Disabled")) -> ()  [unwired: 2 in, 2 out]
            n959 = property on="Y Scan Length SP steps" class="DigNum (strict)"("DisabledEnum"=T2."Disabled and Grayed Out" ("Disabled")) -> ()  [unwired: 2 in, 2 out]
            n960 = property on="Y Scan Velocity SP steps/sec" class="DigNum (strict)"("DisabledEnum"=T2."Disabled and Grayed Out" ("Disabled")) -> ()  [unwired: 2 in, 2 out]
          }
          frame #2 {
            n961 = property on="Y Go" class="Bool"("DisabledEnum"=T2."Disabled and Grayed Out" ("Disabled")) -> ()  [unwired: 2 in, 2 out]
          }
        }
      }
      event #18 {
        n962 = event-data() -> ()  [unwired: 1 in, 7 out]
        n963 = flat-sequence {
          tunnel: [w1574] -> w1569
          tunnel: [w1588] -> w1568
          tunnel: w1565 -> [w1570]
          tunnel: w1564 -> [w1571]
          tunnel: w1569 -> [w1595]
          tunnel: w1568 -> [w1594]
          tunnel: [w1595] -> w1567
          tunnel: [w1594] -> w1566
          tunnel: [w1597] -> w1563
          tunnel: [w1598] -> w1562
          tunnel: w1567 -> [w1598]
          tunnel: w1566 -> [w1597]
          frame #0 {
            # "VELOCITY"
            n964 = property on="Z steps/rev" class="DigNum (strict)"() -> ("Value"=w1577:u32)  [unwired: 2 in, 2 out]
            n965 = property on="Z Scan Velocity SP steps/sec" class="DigNum (strict)"() -> ("Value"=w1584:i32)  [unwired: 2 in, 2 out]
            n966 = Divide(x=w1584, y=w1577) -> (x/y=w1585:dbl)
            n967 = Number To Fractional String(number=w1585) -> (F-format string=w1586:string)  [unwired: 3 in]
            n968 = call "Applied Send Command.vi"("error in (no error)"=w1571, "Extra"=w1586, "Command"=T1."Velocity Setting", "VISA resource name"=w1570) -> ("error out"=w1583:errorcluster, "VISA resource name out"=w1573:refnum<visa-resource-name>)  [unwired: 3 in, 1 out]
            n969 = call "Time Delay24"("error in (no error)"=w1583) -> ("error out"=w1572:errorcluster)  [unwired: 10 in]
            n970 = call "Applied Send Command.vi"("error in (no error)"=w1572, "Extra"="", "Command"=T1."Velocity Setting", "VISA resource name"=w1573) -> ("error out"=w1575:errorcluster, "read buffer"=w1580:string, "VISA resource name out"=w1574:refnum<visa-resource-name>)  [unwired: 3 in]
            n971 = call "Time Delay25"("error in (no error)"=w1575) -> ("error out"=w1588:errorcluster)  [unwired: 10 in]
            n972 = Fract/Exp String To Number(string=w1580, offset=3) -> (number=w1579:dbl)  [unwired: 2 in, 1 out]
            n973 = Multiply(x=w1579, y=w1577) -> (x*y=w1576:dbl)
            n974 = property on="Z  velocity PV step/sec" class="DigNum (strict)"("Val(Sgnl)"=w1576) -> ()  [unwired: 2 in, 2 out]
          }
          frame #1 {
            n975 = property on="Z Scan" class="Bool (strict)"("Val(Sgnl)"=TRUE ("Slew Ready 2")) -> ()  [unwired: 2 in, 2 out]
            n976 = property on="Scan Cancel" class="Bool"("DisabledEnum"=T2."Enabled" ("Disabled")) -> ()  [unwired: 2 in, 2 out]
            n977 = property on="Scan Go" class="Bool"("DisabledEnum"=T2."Enabled" ("Disabled")) -> ()  [unwired: 2 in, 2 out]
            n978 = property on="Z Scan Length SP steps" class="DigNum (strict)"("DisabledEnum"=T2."Disabled and Grayed Out" ("Disabled")) -> ()  [unwired: 2 in, 2 out]
            n979 = property on="Z Scan Velocity SP steps/sec" class="DigNum (strict)"("DisabledEnum"=T2."Disabled and Grayed Out" ("Disabled")) -> ()  [unwired: 2 in, 2 out]
          }
          frame #2 {
            n980 = property on="Z Go" class="Bool"("DisabledEnum"=T2."Disabled and Grayed Out" ("Disabled")) -> ()  [unwired: 2 in, 2 out]
          }
        }
      }
      event #19 {
        n981 = event-data() -> ()  [unwired: 1 in, 7 out]
        n982 = flat-sequence {
          tunnel: [w1610] -> w1606
          tunnel: [w1625] -> w1605
          tunnel: w1602 -> [w1618]
          tunnel: w1601 -> [w1619]
          tunnel: w1606 -> [w1632]
          tunnel: w1605 -> [w1631]
          tunnel: [w1632] -> w1604
          tunnel: [w1631] -> w1603
          tunnel: [w1634] -> w1599
          tunnel: [w1635] -> w1600
          tunnel: w1604 -> [w1635]
          tunnel: w1603 -> [w1634]
          frame #0 {
            # "VELOCITY"
            n983 = property on="R steps/rev" class="DigNum (strict)"() -> ("Value"=w1608:u32)  [unwired: 2 in, 2 out]
            n984 = property on="R Scan Velocity SP steps/sec" class="DigNum (strict)"() -> ("Value"=w1620:i32)  [unwired: 2 in, 2 out]
            n985 = Divide(x=w1620, y=w1608) -> (x/y=w1622:dbl)
            n986 = Number To Fractional String(number=w1622) -> (F-format string=w1623:string)  [unwired: 3 in]
            n987 = call "Applied Send Command.vi"("error in (no error)"=w1619, "Extra"=w1623, "Command"=T1."Velocity Setting", "VISA resource name"=w1618) -> ("error out"=w1621:errorcluster, "VISA resource name out"=w1612:refnum<visa-resource-name>)  [unwired: 3 in, 1 out]
            n988 = call "Time Delay26"("error in (no error)"=w1621) -> ("error out"=w1611:errorcluster)  [unwired: 10 in]
            n989 = call "Applied Send Command.vi"("error in (no error)"=w1611, "Extra"="", "Command"=T1."Velocity Setting", "VISA resource name"=w1612) -> ("error out"=w1609:errorcluster, "read buffer"=w1615:string, "VISA resource name out"=w1610:refnum<visa-resource-name>)  [unwired: 3 in]
            n990 = call "Time Delay27"("error in (no error)"=w1609) -> ("error out"=w1625:errorcluster)  [unwired: 10 in]
            n991 = Fract/Exp String To Number(string=w1615, offset=3) -> (number=w1614:dbl)  [unwired: 2 in, 1 out]
            n992 = Multiply(x=w1614, y=w1608) -> (x*y=w1607:dbl)
            n993 = property on="R velocity PV step/sec" class="DigNum (strict)"("Val(Sgnl)"=w1607) -> ()  [unwired: 2 in, 2 out]
          }
          frame #1 {
            n994 = property on="R Scan" class="Bool (strict)"("Val(Sgnl)"=TRUE ("Slew Ready 2")) -> ()  [unwired: 2 in, 2 out]
            n995 = property on="Scan Cancel" class="Bool"("DisabledEnum"=T2."Enabled" ("Disabled")) -> ()  [unwired: 2 in, 2 out]
            n996 = property on="Scan Go" class="Bool"("DisabledEnum"=T2."Enabled" ("Disabled")) -> ()  [unwired: 2 in, 2 out]
            n997 = property on="R Scan Length SP steps" class="DigNum (strict)"("DisabledEnum"=T2."Disabled and Grayed Out" ("Disabled")) -> ()  [unwired: 2 in, 2 out]
            n998 = property on="R Scan Velocity SP steps/sec" class="DigNum (strict)"("DisabledEnum"=T2."Disabled and Grayed Out" ("Disabled")) -> ()  [unwired: 2 in, 2 out]
          }
          frame #2 {
            n999 = property on="R Go" class="Bool"("DisabledEnum"=T2."Disabled and Grayed Out" ("Disabled")) -> ()  [unwired: 2 in, 2 out]
          }
        }
      }
      event #20 {
        n1000 = event-data() -> ()  [unwired: 1 in, 4 out]
        n1001 = event-data() -> ()  [unwired: 3 in, 1 out]
      }
      event #21 {
        n1002 = event-data() -> ()  [unwired: 1 in, 7 out]
        n1003 = flat-sequence {
          tunnel: [w1666] -> w1649
          tunnel: [w1665] -> w1648
          tunnel: w1647 -> [w1667]
          tunnel: w1646 -> [w1664]
          frame #0 {
            n1004 = call "Applied Send Command.vi"("error in (no error)"=w1664, "Command"=T1."Stop", "VISA resource name"=w1667) -> ("error out"=w1665:errorcluster, "VISA resource name out"=w1666:refnum<visa-resource-name>)  [unwired: 4 in, 1 out]
          }
        }
        n1005 = flat-sequence {
          tunnel: w1653 -> [w1670]
          tunnel: w1652 -> [w1669]
          tunnel: [w1671] -> w1651
          tunnel: [w1672] -> w1650
          frame #0 {
            n1006 = call "Applied Send Command.vi"("error in (no error)"=w1669, "Command"=T1."Stop", "VISA resource name"=w1670) -> ("error out"=w1672:errorcluster, "VISA resource name out"=w1671:refnum<visa-resource-name>)  [unwired: 4 in, 1 out]
          }
        }
        n1007 = flat-sequence {
          tunnel: [w1661] -> w1643
          tunnel: [w1662] -> w1642
          tunnel: w1645 -> [w1659]
          tunnel: w1644 -> [w1660]
          frame #0 {
            n1008 = call "Applied Send Command.vi"("error in (no error)"=w1660, "Command"=T1."Stop", "VISA resource name"=w1659) -> ("error out"=w1662:errorcluster, "VISA resource name out"=w1661:refnum<visa-resource-name>)  [unwired: 4 in, 1 out]
          }
        }
        n1009 = flat-sequence {
          tunnel: w1641 -> [w1654]
          tunnel: w1640 -> [w1655]
          tunnel: [w1657] -> w1639
          tunnel: [w1656] -> w1638
          frame #0 {
            n1010 = call "Applied Send Command.vi"("error in (no error)"=w1655, "Command"=T1."Stop", "VISA resource name"=w1654) -> ("error out"=w1656:errorcluster, "VISA resource name out"=w1657:refnum<visa-resource-name>)  [unwired: 4 in, 1 out]
          }
        }
      }
      event #22 {
        n1011 = event-data() -> ()  [unwired: 1 in, 7 out]
        n1012 = flat-sequence {
          tunnel: w1689 -> [w1727]
          tunnel: w1688 -> [w1726]
          tunnel: [w1729] -> w1691
          tunnel: [w1728] -> w1690
          tunnel: [w1737] -> w1686
          tunnel: [w1738] -> w1687
          tunnel: w1691 -> [w1738]
          tunnel: w1690 -> [w1737]
          frame #0 {
            n1013 = call "Applied Send Command.vi"("error in (no error)"=w1726, "Command"=T1."Stop", "VISA resource name"=w1727) -> ("error out"=w1728:errorcluster, "VISA resource name out"=w1729:refnum<visa-resource-name>)  [unwired: 4 in, 1 out]
          }
          frame #1 {
            n1014 = property on="X Scan" class="Bool (strict)"("Value"=FALSE ("Slew Ready")) -> ()  [unwired: 2 in, 2 out]
            n1015 = property on="X Scan set" class="Bool"("DisabledEnum"=T2."Enabled" ("Disabled")) -> ()  [unwired: 2 in, 2 out]
            n1016 = property on="X Scan Velocity SP steps/sec" class="DigNum (strict)"("DisabledEnum"=T2."Enabled" ("Disabled")) -> ()  [unwired: 2 in, 2 out]
            n1017 = property on="X Scan Length SP steps" class="DigNum (strict)"("DisabledEnum"=T2."Enabled" ("Disabled")) -> ()  [unwired: 2 in, 2 out]
            n1018 = property on="X Go" class="Bool"("DisabledEnum"=T2."Enabled" ("Disabled")) -> ()  [unwired: 2 in, 2 out]
            n1019 = property on="X Scan OK" class="Bool"("DisabledEnum"=T2."Enabled" ("Disabled")) -> ()  [unwired: 2 in, 2 out]
          }
        }
        n1020 = flat-sequence {
          tunnel: w1697 -> [w1740]
          tunnel: w1696 -> [w1739]
          tunnel: [w1742] -> w1693
          tunnel: [w1741] -> w1692
          tunnel: [w1750] -> w1698
          tunnel: [w1751] -> w1699
          tunnel: w1693 -> [w1751]
          tunnel: w1692 -> [w1750]
          frame #0 {
            n1021 = call "Applied Send Command.vi"("error in (no error)"=w1739, "Command"=T1."Stop", "VISA resource name"=w1740) -> ("error out"=w1741:errorcluster, "VISA resource name out"=w1742:refnum<visa-resource-name>)  [unwired: 4 in, 1 out]
          }
          frame #1 {
            n1022 = property on="Y Scan" class="Bool (strict)"("Value"=FALSE ("Slew Ready")) -> ()  [unwired: 2 in, 2 out]
            n1023 = property on="Y Go" class="Bool"("DisabledEnum"=T2."Enabled" ("Disabled")) -> ()  [unwired: 2 in, 2 out]
            n1024 = property on="Y Scan Velocity SP steps/sec" class="DigNum (strict)"("DisabledEnum"=T2."Enabled" ("Disabled")) -> ()  [unwired: 2 in, 2 out]
            n1025 = property on="Y Scan set" class="Bool"("DisabledEnum"=T2."Enabled" ("Disabled")) -> ()  [unwired: 2 in, 2 out]
            n1026 = property on="Y Scan OK" class="Bool"("DisabledEnum"=T2."Enabled" ("Disabled")) -> ()  [unwired: 2 in, 2 out]
            n1027 = property on="Y Scan Length SP steps" class="DigNum (strict)"("DisabledEnum"=T2."Enabled" ("Disabled")) -> ()  [unwired: 2 in, 2 out]
          }
        }
        n1028 = flat-sequence {
          tunnel: [w1716] -> w1685
          tunnel: [w1715] -> w1684
          tunnel: w1683 -> [w1714]
          tunnel: w1682 -> [w1713]
          tunnel: [w1724] -> w1680
          tunnel: [w1725] -> w1681
          tunnel: w1685 -> [w1725]
          tunnel: w1684 -> [w1724]
          frame #0 {
            n1029 = call "Applied Send Command.vi"("error in (no error)"=w1713, "Command"=T1."Stop", "VISA resource name"=w1714) -> ("error out"=w1715:errorcluster, "VISA resource name out"=w1716:refnum<visa-resource-name>)  [unwired: 4 in, 1 out]
          }
          frame #1 {
            n1030 = property on="Z Scan" class="Bool (strict)"("Value"=FALSE ("Slew Ready")) -> ()  [unwired: 2 in, 2 out]
            n1031 = property on="Z Scan set" class="Bool"("DisabledEnum"=T2."Enabled" ("Disabled")) -> ()  [unwired: 2 in, 2 out]
            n1032 = property on="Z Scan Velocity SP steps/sec" class="DigNum (strict)"("DisabledEnum"=T2."Enabled" ("Disabled")) -> ()  [unwired: 2 in, 2 out]
            n1033 = property on="Z Scan Length SP steps" class="DigNum (strict)"("DisabledEnum"=T2."Enabled" ("Disabled")) -> ()  [unwired: 2 in, 2 out]
            n1034 = property on="Z Go" class="Bool"("DisabledEnum"=T2."Enabled" ("Disabled")) -> ()  [unwired: 2 in, 2 out]
            n1035 = property on="Z Scan OK" class="Bool"("DisabledEnum"=T2."Enabled" ("Disabled")) -> ()  [unwired: 2 in, 2 out]
          }
        }
        n1036 = flat-sequence {
          tunnel: [w1703] -> w1679
          tunnel: [w1702] -> w1678
          tunnel: w1677 -> [w1700]
          tunnel: w1676 -> [w1701]
          tunnel: [w1711] -> w1674
          tunnel: [w1712] -> w1675
          tunnel: w1679 -> [w1712]
          tunnel: w1678 -> [w1711]
          frame #0 {
            n1037 = call "Applied Send Command.vi"("error in (no error)"=w1701, "Command"=T1."Stop", "VISA resource name"=w1700) -> ("error out"=w1702:errorcluster, "VISA resource name out"=w1703:refnum<visa-resource-name>)  [unwired: 4 in, 1 out]
          }
          frame #1 {
            n1038 = property on="R Scan" class="Bool (strict)"("Value"=FALSE ("Slew Ready")) -> ()  [unwired: 2 in, 2 out]
            n1039 = property on="R Scan Velocity SP steps/sec" class="DigNum (strict)"("DisabledEnum"=T2."Enabled" ("Disabled")) -> ()  [unwired: 2 in, 2 out]
            n1040 = property on="R Go" class="Bool"("DisabledEnum"=T2."Enabled" ("Disabled")) -> ()  [unwired: 2 in, 2 out]
            n1041 = property on="R Scan OK" class="Bool"("DisabledEnum"=T2."Enabled" ("Disabled")) -> ()  [unwired: 2 in, 2 out]
            n1042 = property on="R Scan Length SP steps" class="DigNum (strict)"("DisabledEnum"=T2."Enabled" ("Disabled")) -> ()  [unwired: 2 in, 2 out]
            n1043 = property on="R Scan set" class="Bool"("DisabledEnum"=T2."Enabled" ("Disabled")) -> ()  [unwired: 2 in, 2 out]
          }
        }
        n1044 = property on="Scan Go" class="Bool"("DisabledEnum"=T2."Disabled and Grayed Out" ("Disabled")) -> ()  [unwired: 2 in, 2 out]
        n1045 = property on="Scan Cancel" class="Bool"("DisabledEnum"=T2."Disabled and Grayed Out" ("Disabled")) -> ()  [unwired: 2 in, 2 out]
      }
      event #23 {
        n1046 = event-data() -> ()  [unwired: 1 in, 7 out]
        n1047 = flat-sequence {
          tunnel: w1787 -> [w1806]
          tunnel: w1786 -> [w1807]
          tunnel: w1785 -> [w1804]
          tunnel: w1784 -> [w1805]
          tunnel: w1783 -> [w1803]
          tunnel: w1782 -> [w1802]
          tunnel: w1781 -> [w1801]
          tunnel: w1780 -> [w1800]
          tunnel: [w1799] -> w1771
          tunnel: [w1798] -> w1769
          tunnel: [w1797] -> w1767
          tunnel: [w1796] -> w1765
          tunnel: [w1795] -> w1763
          tunnel: [w1794] -> w1761
          tunnel: [w1793] -> w1759
          tunnel: [w1792] -> w1757
          tunnel: [w1791] -> w1755
          tunnel: [w1790] -> w1754
          tunnel: [w1789] -> w1753
          tunnel: [w1788] -> w1752
          tunnel: w1771 -> [w1863]
          tunnel: [w1862] -> w1770
          tunnel: w1769 -> [w1861]
          tunnel: [w1860] -> w1768
          tunnel: w1767 -> [w1859]
          tunnel: [w1858] -> w1766
          tunnel: w1765 -> [w1857]
          tunnel: [w1856] -> w1764
          tunnel: w1763 -> [w1855]
          tunnel: [w1854] -> w1762
          tunnel: w1761 -> [w1852]
          tunnel: [w1853] -> w1760
          tunnel: w1759 -> [w1851]
          tunnel: [w1850] -> w1758
          tunnel: w1757 -> [w1849]
          tunnel: [w1848] -> w1756
          tunnel: w1755 -> [w1847]
          tunnel: w1754 -> [w1846]
          tunnel: w1753 -> [w1845]
          tunnel: w1752 -> [w1844]
          tunnel: [w1898] -> w1779
          tunnel: [w1897] -> w1778
          tunnel: [w1896] -> w1777
          tunnel: [w1895] -> w1776
          tunnel: [w1894] -> w1775
          tunnel: [w1893] -> w1774
          tunnel: [w1900] -> w1773
          tunnel: [w1899] -> w1772
          tunnel: w1770 -> [w1900]
          tunnel: w1768 -> [w1899]
          tunnel: w1766 -> [w1898]
          tunnel: w1764 -> [w1897]
          tunnel: w1762 -> [w1896]
          tunnel: w1760 -> [w1895]
          tunnel: w1758 -> [w1894]
          tunnel: w1756 -> [w1893]
          frame #0 {
            n1048 = property on="X Scan" class="Bool (strict)"() -> ("Value"=w1788:bool)  [unwired: 2 in, 2 out]
            n1049 = property on="Y Scan" class="Bool (strict)"() -> ("Value"=w1789:bool)  [unwired: 2 in, 2 out]
            n1050 = property on="Z Scan" class="Bool (strict)"() -> ("Value"=w1790:bool)  [unwired: 2 in, 2 out]
            n1051 = property on="R Scan" class="Bool (strict)"() -> ("Value"=w1791:bool)  [unwired: 2 in, 2 out]
            n1052 = case shown="True" w1788 {
              tunnel: w1807 -> [w1827 w1831]
              tunnel: [w1827 w1830] -> w1798
              tunnel: w1806 -> [w1826 w1829]
              tunnel: [w1826 w1828] -> w1799
              frame #0 {
              }
              frame #1 {
                n1053 = property on="X Scan Length SP steps" class="DigNum (strict)"() -> ("Value"=w1832:i32)  [unwired: 2 in, 2 out]
                n1054 = Number To Decimal String(number=w1832) -> (decimal integer string=w1833:string)  [unwired: 1 in]
                n1055 = call "Applied Send Command.vi"("error in (no error)"=w1831, "Extra"=w1833, "Command"=T1."Distance or Position", "VISA resource name"=w1829) -> ("error out"=w1830:errorcluster, "VISA resource name out"=w1828:refnum<visa-resource-name>)  [unwired: 3 in, 1 out]
              }
            }
            n1056 = case shown="True" w1789 {
              tunnel: w1804 -> [w1836 w1841]
              tunnel: w1805 -> [w1835 w1840]
              tunnel: [w1835 w1837] -> w1796
              tunnel: [w1836 w1838] -> w1797
              frame #0 {
              }
              frame #1 {
                n1057 = property on="Y Scan Length SP steps" class="DigNum (strict)"() -> ("Value"=w1839:i32)  [unwired: 2 in, 2 out]
                n1058 = Number To Decimal String(number=w1839) -> (decimal integer string=w1842:string)  [unwired: 1 in]
                n1059 = call "Applied Send Command.vi"("error in (no error)"=w1840, "Extra"=w1842, "Command"=T1."Distance or Position", "VISA resource name"=w1841) -> ("error out"=w1837:errorcluster, "VISA resource name out"=w1838:refnum<visa-resource-name>)  [unwired: 3 in, 1 out]
              }
            }
            n1060 = case shown="True" w1790 {
              tunnel: w1803 -> [w1818 w1822]
              tunnel: [w1818 w1821] -> w1795
              tunnel: [w1817 w1820] -> w1794
              tunnel: w1802 -> [w1817 w1819]
              frame #0 {
              }
              frame #1 {
                n1061 = property on="Z Scan Length SP steps" class="DigNum (strict)"() -> ("Value"=w1823:i32)  [unwired: 2 in, 2 out]
                n1062 = Number To Decimal String(number=w1823) -> (decimal integer string=w1824:string)  [unwired: 1 in]
                n1063 = call "Applied Send Command.vi"("error in (no error)"=w1819, "Extra"=w1824, "Command"=T1."Distance or Position", "VISA resource name"=w1822) -> ("error out"=w1820:errorcluster, "VISA resource name out"=w1821:refnum<visa-resource-name>)  [unwired: 3 in, 1 out]
              }
            }
            n1064 = case shown="True" w1791 {
              tunnel: w1801 -> [w1809 w1814]
              tunnel: [w1809 w1813] -> w1793
              tunnel: w1800 -> [w1808 w1812]
              tunnel: [w1808 w1811] -> w1792
              frame #0 {
              }
              frame #1 {
                n1065 = property on="R Scan Length SP steps" class="DigNum (strict)"() -> ("Value"=w1810:i32)  [unwired: 2 in, 2 out]
                n1066 = Number To Decimal String(number=w1810) -> (decimal integer string=w1815:string)  [unwired: 1 in]
                n1067 = call "Applied Send Command.vi"("error in (no error)"=w1812, "Extra"=w1815, "Command"=T1."Distance or Position", "VISA resource name"=w1814) -> ("error out"=w1811:errorcluster, "VISA resource name out"=w1813:refnum<visa-resource-name>)  [unwired: 3 in, 1 out]
              }
            }
          }
          frame #1 {
            n1068 = case shown="True" w1844 {
              tunnel: w1863 -> [w1886 w1890]
              tunnel: [w1886 w1889] -> w1862
              tunnel: w1861 -> [w1885 w1888]
              tunnel: [w1885 w1887] -> w1860
              frame #0 {
              }
              frame #1 {
                n1069 = call "Applied Send Command.vi"("error in (no error)"=w1888, "Command"=T1."Feed to Length", "VISA resource name"=w1890) -> ("error out"=w1887:errorcluster, "VISA resource name out"=w1889:refnum<visa-resource-name>)  [unwired: 4 in, 1 out]
              }
            }
            n1070 = case shown="True" w1845 {
              tunnel: w1859 -> [w1879 w1883]
              tunnel: [w1879 w1882] -> w1858
              tunnel: w1857 -> [w1878 w1881]
              tunnel: [w1878 w1880] -> w1856
              frame #0 {
              }
              frame #1 {
                n1071 = call "Applied Send Command.vi"("error in (no error)"=w1881, "Command"=T1."Feed to Length", "VISA resource name"=w1883) -> ("error out"=w1880:errorcluster, "VISA resource name out"=w1882:refnum<visa-resource-name>)  [unwired: 4 in, 1 out]
              }
            }
            n1072 = case shown="False" w1846 {
              tunnel: w1855 -> [w1872 w1876]
              tunnel: [w1872 w1875] -> w1854
              tunnel: [w1871 w1874] -> w1853
              tunnel: w1852 -> [w1871 w1873]
              frame #0 {
              }
              frame #1 {
                n1073 = call "Applied Send Command.vi"("error in (no error)"=w1873, "Command"=T1."Feed to Length", "VISA resource name"=w1876) -> ("error out"=w1874:errorcluster, "VISA resource name out"=w1875:refnum<visa-resource-name>)  [unwired: 4 in, 1 out]
              }
            }
            n1074 = case shown="False" w1847 {
              tunnel: w1851 -> [w1865 w1869]
              tunnel: [w1865 w1868] -> w1850
              tunnel: w1849 -> [w1864 w1867]
              tunnel: [w1864 w1866] -> w1848
              frame #0 {
              }
              frame #1 {
                n1075 = call "Applied Send Command.vi"("error in (no error)"=w1867, "Command"=T1."Feed to Length", "VISA resource name"=w1869) -> ("error out"=w1866:errorcluster, "VISA resource name out"=w1868:refnum<visa-resource-name>)  [unwired: 4 in, 1 out]
              }
            }
          }
          frame #2 {
            n1076 = call "Time Delay7"("Delay Time (s)"=0.1) -> ()  [unwired: 10 in, 1 out]
            n1077 = property on="R Scan" class="Bool (strict)"("Val(Sgnl)"=FALSE ("Slew Ready 2")) -> ()  [unwired: 2 in, 2 out]
            n1078 = property on="X Scan" class="Bool (strict)"("Val(Sgnl)"=FALSE ("Slew Ready 2")) -> ()  [unwired: 2 in, 2 out]
            n1079 = property on="Y Scan" class="Bool (strict)"("Val(Sgnl)"=FALSE ("Slew Ready 2")) -> ()  [unwired: 2 in, 2 out]
            n1080 = property on="Z Scan" class="Bool (strict)"("Val(Sgnl)"=FALSE ("Slew Ready 2")) -> ()  [unwired: 2 in, 2 out]
            n1081 = property on="Z Scan Velocity SP steps/sec" class="DigNum (strict)"("DisabledEnum"=T2."Enabled" ("Disabled")) -> ()  [unwired: 2 in, 2 out]
            n1082 = property on="Y Scan Length SP steps" class="DigNum (strict)"("DisabledEnum"=T2."Enabled" ("Disabled")) -> ()  [unwired: 2 in, 2 out]
            n1083 = property on="X Scan Velocity SP steps/sec" class="DigNum (strict)"("DisabledEnum"=T2."Enabled" ("Disabled")) -> ()  [unwired: 2 in, 2 out]
            n1084 = property on="R Scan Velocity SP steps/sec" class="DigNum (strict)"("DisabledEnum"=T2."Enabled" ("Disabled")) -> ()  [unwired: 2 in, 2 out]
            n1085 = property on="R Scan Length SP steps" class="DigNum (strict)"("DisabledEnum"=T2."Enabled" ("Disabled")) -> ()  [unwired: 2 in, 2 out]
            n1086 = property on="X Scan Length SP steps" class="DigNum (strict)"("DisabledEnum"=T2."Enabled" ("Disabled")) -> ()  [unwired: 2 in, 2 out]
            n1087 = property on="Y Scan Selocity SP steps/sec" class="DigNum (strict)"("DisabledEnum"=T2."Enabled" ("Disabled")) -> ()  [unwired: 2 in, 2 out]
            n1088 = property on="Z Scan Length SP steps" class="DigNum (strict)"("DisabledEnum"=T2."Enabled" ("Disabled")) -> ()  [unwired: 2 in, 2 out]
            n1089 = property on="Scan Go" class="Bool"("DisabledEnum"=T2."Disabled and Grayed Out" ("Disabled")) -> ()  [unwired: 2 in, 2 out]
            n1090 = property on="Scan Cancel" class="Bool"("DisabledEnum"=T2."Disabled and Grayed Out" ("Disabled")) -> ()  [unwired: 2 in, 2 out]
          }
        }
      }
      event #24 {
        n1091 = event-data() -> ()  [unwired: 1 in, 7 out]
        n1092 = flat-sequence {
          tunnel: [w1945] -> w1924
          tunnel: w1925 -> [w1947]
          tunnel: [w1946] -> w1923
          tunnel: w1926 -> [w1948]
          frame #0 {
            n1093 = property on="Reset X Motor Steps" class="DigNum (strict)"() -> ("Value"=w1951:i32)  [unwired: 2 in, 2 out]
            n1094 = Number To Decimal String(number=w1951) -> (decimal integer string=w1949:string)  [unwired: 1 in]
            n1095 = call "Applied Send Command.vi"("error in (no error)"=w1947, "Extra"=w1949, "Command"=T1."Set ABS Position", "VISA resource name"=w1948) -> ("error out"=w1946:errorcluster, "VISA resource name out"=w1945:refnum<visa-resource-name>)  [unwired: 3 in, 1 out]
          }
        }
        n1096 = flat-sequence {
          tunnel: w1930 -> [w1956]
          tunnel: w1929 -> [w1953]
          tunnel: [w1955] -> w1928
          tunnel: [w1954] -> w1927
          frame #0 {
            n1097 = property on="Reset Y Motor Steps" class="DigNum (strict)"() -> ("Value"=w1958:i32)  [unwired: 2 in, 2 out]
            n1098 = Number To Decimal String(number=w1958) -> (decimal integer string=w1957:string)  [unwired: 1 in]
            n1099 = call "Applied Send Command.vi"("error in (no error)"=w1953, "Extra"=w1957, "Command"=T1."Set ABS Position", "VISA resource name"=w1956) -> ("error out"=w1954:errorcluster, "VISA resource name out"=w1955:refnum<visa-resource-name>)  [unwired: 3 in, 1 out]
          }
        }
        n1100 = flat-sequence {
          tunnel: [w1936] -> w1918
          tunnel: [w1935] -> w1917
          tunnel: w1920 -> [w1934]
          tunnel: w1919 -> [w1933]
          frame #0 {
            n1101 = property on="Reset R Motor Steps" class="DigNum (strict)"() -> ("Value"=w1937:i32)  [unwired: 2 in, 2 out]
            n1102 = Number To Decimal String(number=w1937) -> (decimal integer string=w1932:string)  [unwired: 1 in]
            n1103 = call "Applied Send Command.vi"("error in (no error)"=w1933, "Extra"=w1932, "Command"=T1."Set ABS Position", "VISA resource name"=w1934) -> ("error out"=w1935:errorcluster, "VISA resource name out"=w1936:refnum<visa-resource-name>)  [unwired: 3 in, 1 out]
          }
        }
        n1104 = flat-sequence {
          tunnel: [w1943] -> w1916
          tunnel: [w1942] -> w1915
          tunnel: w1922 -> [w1940]
          tunnel: w1921 -> [w1941]
          frame #0 {
            n1105 = property on="Reset Z Motor Steps" class="DigNum (strict)"() -> ("Value"=w1944:i32)  [unwired: 2 in, 2 out]
            n1106 = Number To Decimal String(number=w1944) -> (decimal integer string=w1938:string)  [unwired: 1 in]
            n1107 = call "Applied Send Command.vi"("error in (no error)"=w1941, "Extra"=w1938, "Command"=T1."Set ABS Position", "VISA resource name"=w1940) -> ("error out"=w1942:errorcluster, "VISA resource name out"=w1943:refnum<visa-resource-name>)  [unwired: 3 in, 1 out]
          }
        }
      }
    }
    n1108 = case shown="True" "Set Button" {
      tunnel: "Preset positions" -> [_ w412]
      frame #0 {
      }
      frame #1 {
        n1109 = property on="Presets" class="Arr (strict)"() -> ("Value"=w409:i32[][])  [unwired: 2 in, 2 out]
        n1110 = Index Array(array=w409, index (row)=w412) -> (element=w411:i32[])  [unwired: 1 in]
        n1111 = Array To Cluster(array=w411) -> (cluster=w410:T4)
        n1112 = Unbundle(w410) -> ("Value[0]"=w408:i32, "Value[1]"=w407:i32, "Value[2]"=w406:i32, "Value[3]"=w405:i32)  [unwired: 5 out]
        n1113 = property on="X Step SP" class="DigNum (strict)"("Val(Sgnl)"=w408) -> ()  [unwired: 2 in, 2 out]
        n1114 = property on="Y Step SP" class="DigNum (strict)"("Val(Sgnl)"=w407) -> ()  [unwired: 2 in, 2 out]
        n1115 = property on="Z Step SP" class="DigNum (strict)"("Val(Sgnl)"=w406) -> ()  [unwired: 2 in, 2 out]
        n1116 = property on="R Step SP" class="DigNum (strict)"("Val(Sgnl)"=w405) -> ()  [unwired: 2 in, 2 out]
      }
    }
    n1117 = case shown="True" "Add Button" {
      tunnel: w369 -> [_ w404]
      frame #0 {
      }
      frame #1 {
        n1118 = property on="X Step PV" class="DigNum (strict)"() -> ("Value"=w399:i32)  [unwired: 2 in, 2 out]
        n1119 = property on="Y Step PV" class="DigNum (strict)"() -> ("Value"=w398:i32)  [unwired: 2 in, 2 out]
        n1120 = property on="Z Step PV" class="DigNum (strict)"() -> ("Value"=w397:i32)  [unwired: 2 in, 2 out]
        n1121 = property on="R Step PV" class="DigNum (strict)"() -> ("Value"=w396:i32)  [unwired: 2 in, 2 out]
        n1122 = Build Array(w399, w398, w397, w396) -> (w402:i32[])
        n1123 = Build Array (concatenate)(w404, "String") -> (w403:string[])
        n1124 = property on="Preset positions" class="Ring (strict)"("Strings []"=w403) -> ()  [unwired: 2 in, 2 out]
        n1125 = property on="Presets" class="Arr (strict)"() -> ("Value"=w401:i32[][])  [unwired: 2 in, 2 out]
        n1126 = Build Array (concatenate)(w401, w402) -> (w395:i32[][])
        n1127 = property on="Presets" class="Arr (strict)"("Val(Sgnl)"=w395) -> ()  [unwired: 2 in, 2 out]
      }
    }
    n1128 = case shown="True" "Delete Button" {
      tunnel: w369 -> [_ w394]
      frame #0 {
      }
      frame #1 {
        n1129 = property on="Preset positions" class="Ring (strict)"() -> ("Value"=w392:i32)  [unwired: 2 in, 2 out]
        n1130 = property on="Presets" class="Arr (strict)"() -> ("Value"=w391:i32[][])  [unwired: 2 in, 2 out]
        n1131 = Delete From Array(array=w394, index=w392) -> (array with subset deleted=w393:string[])  [unwired: 1 in, 1 out]
        n1132 = property on="Preset positions" class="Ring (strict)"("Strings []"=w393) -> ()  [unwired: 2 in, 2 out]
        n1133 = Delete From Array(array=w391, index (row)=w392) -> (array with subset deleted=w390:i32[][])  [unwired: 2 in, 1 out]
        n1134 = property on="Presets" class="Arr (strict)"("Val(Sgnl)"=w390) -> ()  [unwired: 2 in, 2 out]
      }
    }
  }
  n1135 = flat-sequence {
    tunnel: w70 -> [w1960]
    tunnel: w69 -> [w1959]
    tunnel: [w1971] -> w46
    frame #0 {
      # "GET CURRENT POSITION"
      n1136 = call "Applied Send Command.vi"("error in (no error)"=w1959, "Extra"="", "Command"=T1."Immediate Position?", "VISA resource name"=w1960) -> ("error out"=w1961:errorcluster, "read buffer"=w1966:string, "VISA resource name out"=w1962:refnum<visa-resource-name>)  [unwired: 3 in]
      n1137 = call "Applied Send Command.vi"("error in (no error)"=w1961, "Command"=T1."Stop & Kill Buffer", "VISA resource name"=w1962) -> ("error out"=w1968:errorcluster, "VISA resource name out"=w1969:refnum<visa-resource-name>)  [unwired: 4 in, 1 out]
      n1138 = Hexadecimal String To Number(string=w1966, offset=3) -> (number=w1963:u32)  [unwired: 1 in, 1 out]
      n1139 = VISA Close(VISA resource name=w1969, error in (no error)=w1968) -> ()  [unwired: 1 out]
      n1140 = To Long Integer(number=w1963) -> (32bit integer=w1971:i32)
    }
  }
  n1141 = flat-sequence {
    tunnel: w50 -> [w1974]
    tunnel: w49 -> [w1973]
    tunnel: [w1972] -> w45
    frame #0 {
      # "GET CURRENT POSITION"
      n1142 = call "Applied Send Command.vi"("error in (no error)"=w1973, "Extra"="", "Command"=T1."Immediate Position?", "VISA resource name"=w1974) -> ("error out"=w1975:errorcluster, "read buffer"=w1980:string, "VISA resource name out"=w1976:refnum<visa-resource-name>)  [unwired: 3 in]
      n1143 = call "Applied Send Command.vi"("error in (no error)"=w1975, "Command"=T1."Stop & Kill Buffer", "VISA resource name"=w1976) -> ("error out"=w1982:errorcluster, "VISA resource name out"=w1983:refnum<visa-resource-name>)  [unwired: 4 in, 1 out]
      n1144 = Hexadecimal String To Number(string=w1980, offset=3) -> (number=w1977:u32)  [unwired: 1 in, 1 out]
      n1145 = VISA Close(VISA resource name=w1983, error in (no error)=w1982) -> ()  [unwired: 1 out]
      n1146 = To Long Integer(number=w1977) -> (32bit integer=w1972:i32)
    }
  }
  n1147 = flat-sequence {
    tunnel: w52 -> [w1986]
    tunnel: w51 -> [w1985]
    tunnel: [w1987] -> w44
    frame #0 {
      # "GET CURRENT POSITION"
      n1148 = call "Applied Send Command.vi"("error in (no error)"=w1985, "Extra"="", "Command"=T1."Immediate Position?", "VISA resource name"=w1986) -> ("error out"=w1988:errorcluster, "read buffer"=w1993:string, "VISA resource name out"=w1989:refnum<visa-resource-name>)  [unwired: 3 in]
      n1149 = call "Applied Send Command.vi"("error in (no error)"=w1988, "Command"=T1."Stop & Kill Buffer", "VISA resource name"=w1989) -> ("error out"=w1995:errorcluster, "VISA resource name out"=w1996:refnum<visa-resource-name>)  [unwired: 4 in, 1 out]
      n1150 = Hexadecimal String To Number(string=w1993, offset=3) -> (number=w1990:u32)  [unwired: 1 in, 1 out]
      n1151 = VISA Close(VISA resource name=w1996, error in (no error)=w1995) -> ()  [unwired: 1 out]
      n1152 = To Long Integer(number=w1990) -> (32bit integer=w1987:i32)
    }
  }
  n1153 = flat-sequence {
    tunnel: w48 -> [w1999]
    tunnel: w47 -> [w1998]
    tunnel: [w2000] -> w43
    frame #0 {
      # "GET CURRENT POSITION"
      n1154 = call "Applied Send Command.vi"("error in (no error)"=w1998, "Extra"="", "Command"=T1."Immediate Position?", "VISA resource name"=w1999) -> ("error out"=w2001:errorcluster, "read buffer"=w2006:string, "VISA resource name out"=w2002:refnum<visa-resource-name>)  [unwired: 3 in]
      n1155 = call "Applied Send Command.vi"("error in (no error)"=w2001, "Command"=T1."Stop & Kill Buffer", "VISA resource name"=w2002) -> ("error out"=w2008:errorcluster, "VISA resource name out"=w2009:refnum<visa-resource-name>)  [unwired: 4 in, 1 out]
      n1156 = Hexadecimal String To Number(string=w2006, offset=3) -> (number=w2003:u32)  [unwired: 1 in, 1 out]
      n1157 = VISA Close(VISA resource name=w2009, error in (no error)=w2008) -> ()  [unwired: 1 out]
      n1158 = To Long Integer(number=w2003) -> (32bit integer=w2000:i32)
    }
  }
  n1159 = flat-sequence {
    tunnel: w46 -> [w2016]
    tunnel: w45 -> [w2015]
    tunnel: w44 -> [w2014]
    tunnel: w43 -> [w2013]
    frame #0 {
      n1160 = Build Array(w2016, w2015, w2014, w2013) -> (w2011:i32[])
      n1161 = call-poly <vilib>:"Write To Spreadsheet File.vi"("1D data"=w2011, "file path (dialog if empty)"=path "S:/LV codes/SCL2/POS.TXT") -> ()  [unwired: 6 in, 1 out]
    }
    frame #1 {
      n1162 = property on="Presets" class="Arr (strict)"() -> ("Value"=w2023:i32[][])  [unwired: 2 in, 2 out]
      n1163 = property on="Preset positions" class="Ring (strict)"() -> ("Strings []"=w2019:string[])  [unwired: 2 in, 2 out]
      n1164 = Number To Decimal String(number=w2023) -> (decimal integer string=w2017:string[][])  [unwired: 1 in]
      n1165 = Transpose 2D Array(2D array=w2017) -> (transposed array=w2018:string[][])
      n1166 = Build Array (concatenate)(w2019, w2018) -> (w2020:string[][])
      n1167 = Transpose 2D Array(2D array=w2020) -> (transposed array=w2021:string[][])
      n1168 = call-poly <vilib>:"Write To Spreadsheet File.vi"("2D data"=w2021, "file path (dialog if empty)"=path "S:/LV codes/SCL2/PRESET.TXT") -> ()  [unwired: 6 in, 1 out]
    }
  }
